vi "Tracker.vi"(8 "error in (no error)":errorcluster, 11 "Settings file path":path=path "D:/Users/Dmitriy/CData/CloudStation/Tracker_repository/SubVi's/Tracker_settings.tcf") -> (0 "error out":errorcluster)   [LabVIEW 2016]
uses:
  <vilib>/Utility/config.llb/Config Data RefNum.ctl
  <vilib>/Utility/miscctls.llb/LVPoint32TypeDef.ctl
  <vilib>/Utility/miscctls.llb/LVPointTypeDef.ctl
  <vilib>/Instr/_visa.llb/VISA Flush IO Buffer Mask.ctl
  <vilib>/Utility/miscctls.llb/LVRangeTypeDef.ctl
  <vilib>/Utility/miscctls.llb/LVBoundsTypeDef.ctl
  <vilib>/Utility/miscctls.llb/LVStringsAndValuesArrayTypeDef_U16.ctl
  <extravilib>/ChannelInstances/Lossy Stream-a[.,.](str)/Write With Abort.vi
  <extravilib>/ChannelInstances/Lossy Stream-a[.,.](str)/Read With Abort.vi
  <extravilib>/ChannelInstances/Lossy Stream-a[.,.](str)/Endpoint.vi
  SubVi's/SW_Globals.vi
  <vilib>/Utility/file.llb/Write Delimited Spreadsheet (string).vi
  <vilib>/Utility/file.llb/Read Delimited Spreadsheet (string).vi
  <extravilib>/ChannelInstances/Lossy Stream-a[.,.](str)/Instantiate.vi
  <extravilib>/ChannelInstances/Lossy Stream-a[.,.](str)/)Channel.vi
  <resource>/ChannelSupport/_ChannelSupport/WaitIfNeeded.vi
  <vilib>/Utility/config.llb/NI_LVConfig.lvlib
  <vilib>/Analysis/NI_AALBase.lvlib
  <extravilib>/ChannelInstances/Lossy Stream-a[.,.](str).lvlib
panel:
  in  "Map index (analysis)":i32
  in  "Full trace color":u32(colorbox)=16757314
  out "Current TTL status":u8
  out "TTL inputs":u8[](array[numeric])
  out "TTL outputs":u8[](array[numeric])
  out "Start/Stop in config":u32
  out "Start/Stop out pulses config":u32
  out "Changed IO":bool
  out "Sync capability":u8
  in  "IO parameters string":string
  out "Reset STIM":bool
  out "Reset REG":bool
  out "Init plot":bool=TRUE
  in  "Back to Settings":bool
  out "Zones preference array (loaded)":dbl[][](array[numeric])
  out "Current segment":dbl[](array[numeric])
  out "Absolute timestamp (rec)":dbl[](array[numeric])
  in  "Colors for Stim. setup":T1(array[cluster])=[{"Not Selected"=1143775, "Not Selected"=1143775}, {"Not Selected"=14517504, "Not Selected"=14517504}, {"Not Selected"=1976113, "Not Selected"=1976113}, {"Not Selected"=2575993, "Not Selected"=2575993}]
  out "Record":bool
  out "Stopped":bool
  out "Reset starting pulse":bool
  out "TTL is long enough":bool
  out "Started":bool
  out "Coords":T2={"Horizontal"=316, "Vertical"=127}
  out "Button":u16=1
  out "Settings file path":path
  out "Track path":path
  out "Index of the last recorded timepoint":i32
  out "ceil(x): smallest int >= x":dbl
  out "Application Directory":path
  out "Path to the settings file":path=path "D:/Users/Dmitriy/CData/CloudStation/Tracker_repository/Tracker_settings.tcf"
  out "Estim. res":dbl=0.2677563343586869
  in  "SD calc buffer length":u32=100
  out "Eff. save interval":sgl=7.981
  out "Relative timestamp (rec)":dbl[](array[numeric])
  out "FPS":dbl=27.77777777777778
  out "alpha rot. angle":dbl[](array[numeric])
  out "Y coord":dbl[](array[numeric])
  out "X coord":dbl[](array[numeric])
  out "Data column names":string[](array[string])
  out "Zones allocation array":i32[](array[numeric])
  out "Zones presence array":bool[](array[boolean])
  in  "Stop Button":bool
  out "Path to the latest saved temp file":path
  out "Temp file ready":bool
  out "Pixels per mm":dbl=1.1663076923076923
  out "Settings file refnum out":T3
  out "Current User":string="Researcher"
  in  "Main tab control":enum32{"Settings", "Recording", "Analysis"}(tab)
  out "IO status indicator":T4
  in  "Set IO config":bool
  in  "Jump to Analysis":bool
  in  "Reset stimuli":bool
  in  "Stimulus presets":T5(array[cluster]) {"TTL out" items=["1"=1, "2"=2, "1 + 2"=3]; "Stimulus, s" min=0 max=10000 step=0.1; "Time, s" min=0 max=10000 step=0.1; "Event type" items=["Time spent in zone", "Future options"]}
  in  "Stim. setup":T6(radio)=enum."Zone 13"
  out "Ready":bool=TRUE
  in  "Re-check HW connection":bool
  out "Board size":string="Large"
  in  "Reset regions":bool
  in  "Cage diameter, mm":u16(ring)=333 items=["180 mm"=180, "325 mm"=325, "333 mm"=333]
  in  "Start Tracking button":bool
  in  "Starting angle BORDER":i16
  in  "N segments BORDER":u8=5 max=8
  in  "N segments MIDFIELD":u8=3 min=1 max=4
  in  "Starting angle MIDFIELD":i16=30
  in  "Radius, mm MIDFIELD":u16=110
  in  "Radius, mm CENTER":u16=50 min=5 step=1
  out "Segments diagram":picture
  out "HW info":string
  out "Port":string="Large"
  in  "Bridge swap":bool
  in  "Reset barplot":bool
  out "Mouse speed digi":dbl=0.28949046360238656 caption="Mouse speed" format="%05.1f"
  out "Zone preference (normalized)":dbl[](graph)=[0.0, 0.0, 0.0, 0.0, 0.0, 0.0, 1.0, 0.0, 0.0, 0.0, 0.0]
  in  "Multiplyer of chart RX":u8(slide)=1 min=1 max=10 step=1 scale=1.0..6.0
  in  "Zones presence indicator":T7={"01"=TRUE, "02"=TRUE, "03"=TRUE, "04"=TRUE, "05"=TRUE, "06"=TRUE, "07"=TRUE, "08"=TRUE, "09"=TRUE, "10"=TRUE, "11"=TRUE, "12"=TRUE, "13"=TRUE}
  in  "Zones":bool=TRUE
  in  "Record/Stop":bool
  out "Diagram at recording":picture caption="Mouse track"
  in  "Trace, s":u16(slide)=5 max=30 step=1 scale=0.0..30.0
  in  "Data filtering":u16(ring)=5 items=["None"=0, "Kalman 1/3"=2, "Kalman 1/8"=3, "SG 3/5"=4, "SG 3/11"=5]
  out "Record timestamp":dbl format="%<%H:%M:%S%3u>t"
  out "Current Time":timestamp=timestamp(3610093053.229 s since 1904-01-01) format="%<%H:%M:%S %d.%m.%Y>T"
  in  "Exit 2":bool
  out "Mouse speed":waveform(dbl)(graph)={"t0"=timestamp(3610093053.229 s since 1904-01-01), "dt"=1.0, "Y"=[0.28949046360238656]}
  in  "Vertical offset":sgl caption="Bridge offset" min=-60 max=60 step=0.1 format="%#.1g"
  out "TTL IO 1 (recording)":bool caption="IO 1"
  out "TTL IO 2 (recording)":bool caption="IO 2"
  out "TTL IO 3 (recording)":bool caption="IO 3"
  out "TTL IO 4 (recording)":bool caption="IO 4"
  out "TTL REC":bool
  out "Data loading progress":dbl(slide) scale=0.0..100.0
  in  "Speed":u16(ring)=3 items=["25"=75, "10"=30, "6"=18, "4"=12, "2"=6, "1"=3, "2/3"=2, "1/3"=1]
  in  "Timeline":dbl(slide) min=0.0 step=1.0 scale=0.0..5.043 scale format="%<%H:%M:%S>t"
  in  "Multiplyer of chart RX 2":u8(slide)=1 min=1 max=10 step=1 scale=1.0..6.0
  out "Diagram at analysis":picture caption="Mouse track"
  in  "Play/Pause":bool
  out "Recorded at time":timestamp format="%<%H:%M:%S %d.%m.%Y>T"
  out "Recorded timestamp":dbl format="%<%H:%M:%S%3u>t"
  in  "Zones (analysis)":bool=TRUE caption="Zones"
  out "Mouse speed 2":waveform(dbl)(graph) caption="Mouse speed"
  out "Mouse speed digi 2":dbl format="%05.1f"
  out "Zones allocation (normalized) in analysis":dbl[](graph) caption="Zone preference (normalized)"
  out "Recorded by":string
  in  "Trace in analysis, s":u16(slide)=5 caption="Trace, s" max=30 step=1 scale=0.0..30.0
  in  "Open File":bool
  out "Mouse snout orientation swap (analysis)":bool caption="Swapped"
  in  "Show heatmap (analysis)":bool caption="Heat map"
  in  "Show full track (analysis)":bool caption="Full track"
  out "Vertical offset (analysis)":sgl caption="V. offset" min=-60 max=60 step=0.1 format="%#.1g"
  out "TTL IO 2 (analysis)":bool
  out "TTL IO 1 (analysis)":bool
  out "TTL IO 3 (analysis)":bool
  out "TTL IO 4 (analysis)":bool
  # "v.2.1.0"
  # "Cage segmentation"
  # "BORDER"
  # "CENTER"
  # "MIDFIELD"
  # "v.2.1.0"
  # "v.2.1.0"
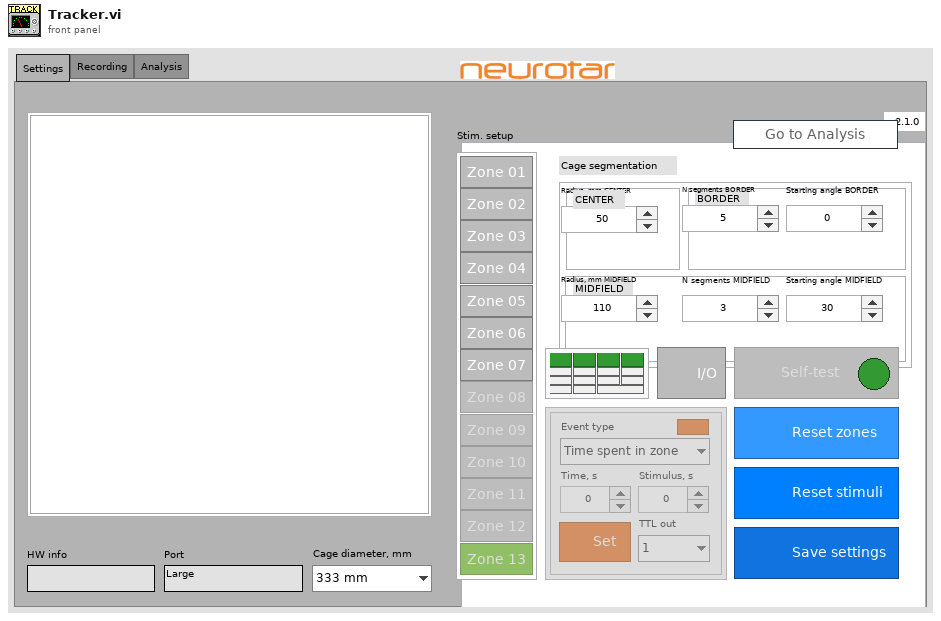
[diagram p1: front panel]
types:
  T1 = cluster{"Not Selected":u32, "Not Selected":u32}[]
  T2 = typedef "LVPoint32TypeDef.ctl" = cluster{"Horizontal":i32, "Vertical":i32}
  T3 = typedef "NI_LVConfig.lvlib/Config Data RefNum.ctl" = refnum<k1>
  T4 = cluster{"IO1":bool, "IO2":bool, "IO3":bool, "IO4":bool, "Z1":bool, "Z2":bool, "Z3":bool, "Z4":bool, "St1":bool, "St2":bool, "St3":bool, "St4":bool, "Syn1":bool, "Syn2":bool, "RS-232 ext. activated":bool}
  T5 = cluster{"Event type":u16, "Time, s":sgl, "Stimulus, s":sgl, "Set/Clear":bool, "TTL out":u16, "Stim. has been set":bool}[]
  T6 = enum32{"No Selection", "Zone 01", "Zone 02", "Zone 03", "Zone 04", "Zone 05", "Zone 06", "Zone 07", "Zone 08", "Zone 09", "Zone 10", "Zone 11", "Zone 12", "Zone 13"}
  T7 = cluster{"01":bool, "02":bool, "03":bool, "04":bool, "05":bool, "06":bool, "07":bool, "08":bool, "09":bool, "10":bool, "11":bool, "12":bool, "13":bool}
  T8 = cluster{"Numeric Control":u32, "Numeric Control":u32}[]
  T9 = enum8{"Enabled", "Disabled", "Disabled and Grayed Out"}
  T10 = cluster{"Read buffer":string, "Timestamp":timestamp}
  T11 = cluster{"Data acquisition status":refnum<notifier>, "Play/Pause status":refnum<notifier>, "Complete stop":refnum<notifier>, "Temp file ready for processing":refnum<notifier>, "Has been recorded":refnum<notifier>, "Recording now":refnum<notifier>, "Path to the latest complete temp file":refnum<notifier>, "Final CSV saved":refnum<notifier>, "Data loaded":refnum<notifier>}
  T12 = cluster{"SYNC configuration":u16, "IO 1 configuration":u16, "IO 2 configuration":u16, "IO 3 configuration":u16, "IO 4 configuration":u16, "Activate ext. RS-232":u16}
  T13 = typedef "VISA Flush IO Buffer Mask.ctl" = u16
  T14 = typedef "LVBoundsTypeDef.ctl" = cluster{"Width":u32, "Height":u32}
  T15 = cluster{"Amount of border segments":u8, "Border segments starting angle":i16, "Amount of midfield segments":u8, "Midfield segments starting angle":i16, "Midfield segments outer radius, mm":u16, "Amount of central segments":u8, "Center segment outer radius, mm":u16, "Diameter of the cage, mm":u16, "R-gap between segments, mm":u8}
  T16 = typedef "LVRangeTypeDef.ctl" = cluster{"Minimum":dbl, "Maximum":dbl, "Increment":dbl, "Minor Increment":dbl, "Start":dbl}
  T17 = cluster{"Width":u16, "Style":enum32{"Solid", "Dash", "Dot", "DashDot", "DashDotDot"}}
  T18 = cluster{"Temporary file output path":path, "Temporary csv output path":path, "Recording settings output path":path, "Final csv output path":path, "Background picture output path":path, "Path to the settings file":path}
  T19 = cluster{"Event type":u16, "Dur., s":sgl, "Stim., s":sgl, "Set/Clear":bool, "TTL out N":u16, "Stim. has been set":bool}[]
  T20 = cluster{"Researcher name":string, "Amount of midfield segments":u32, "Amount of border segments":u32, "Center segment outer radius, mm":u32, "Midfield segments outer radius, mm":u32, "Midfield segments starting angle":i32, "Border segments starting angle":i32, "Cage diameter, mm":u32, "Mouse snout orientation swap?":bool, "Vertical offset":dbl, "Settings loaded OK":bool}
  T21 = typedef "imagedata.ctl" = cluster{"image type":i32, "image depth":i32, "image":u8[], "mask":u8[], "colors":u32[], "Rectangle":cluster{"left":i16, "top":i16, "right":i16, "bottom":i16}}
  T22 = cluster{"Fonts scale factor":dbl, "Pixels per mm":dbl, "Radius of displayed outer segments, pix":dbl, "Radius of displayed midfield segments, pix":dbl, "Radius of displayed central segment, pix":dbl}
  T23 = typedef "Lossy Stream-a[.,.](str).lvlib/)Channel.ctl" = refnum<queue>
  T24 = cluster{"Read buffer":string, "Timestamp":timestamp}[]
  T25 = enum32{"No Selection", "Zone 01", "Zone 02", "Zone 03", "Zone 04", "Zone 05", "Zone 06", "Zone 07", "Zone 08", "Zone 09", "Zone 10", "Zone 11", "Zone 12", "Zone 13", "Zone 14"}
  T26 = enum32{"Page Enabled", "Page Disabled", "Page Disabled & Grayed"}
  T27 = typedef "LVPointTypeDef.ctl" = cluster{"Horizontal":i16, "Vertical":i16}
  T28 = enum32{"invalid app kind", "Development System", "Run Time System", "Student Edition", "Embedded LabVIEW", "Evaluation", "Custom"}
  T29 = cluster{"N segments BORDER":u8, "Starting angle BORDER":i16, "N segments MIDFIELD":u8, "Starting angle MIDFIELD":i16, "Radius, mm MIDFIELD":u16, "Amount of central segments":u8, "Radius, mm CENTER":u16}
  T30 = cluster{"Event type":u16, "Cond., s":sgl, "Stim., s":sgl, "Set/Clear":bool, "TTL out N":u16, "Stim. has been set":bool}
  T31 = cluster{"SYNC configuration":bool, "IO 1 configuration":bool, "IO 2 configuration":bool, "IO 3 configuration":bool, "IO 4 configuration":bool, "Activate ext. RS-232":bool}
  T32 = cluster{"Event type":u16, "Time, s":sgl, "Stimulus, s":sgl, "Set/Clear":bool, "TTL out":u16, "Stim. has been set":bool}
  T33 = typedef "LVStringsAndValuesArrayTypeDef_U16.ctl" = cluster{"String":string, "Value":u16}[]
  T34 = cluster{"N segments BORDER":u8, "Starting angle BORDER":i16, "N segments MIDFIELD":u8, "Starting angle MIDFIELD":i16, "Radius, mm MIDFIELD":u16, u8, "Radius, mm CENTER":u16, "Cage diameter, mm":u16, i32}
  T35 = cluster{"N segments BORDER":u8, "Starting angle BORDER":i16, "N segments MIDFIELD":u8, "Starting angle MIDFIELD":i16, "Radius, mm MIDFIELD":u16, "N segments CENTER":u8, "Radius, mm CENTER":u16, "Cage diameter, mm":u16, "R-gap":i32}
  T36 = cluster{"Zone[1]":bool, "Zone[2]":bool, "Zone[3]":bool, "Zone[4]":bool, "Zone[5]":bool, "Zone[6]":bool, "Zone[7]":bool, "Zone[8]":bool, "Zone[9]":bool, "Zone[10]":bool, "Zone[11]":bool, "Zone[12]":bool, "Zone[13]":bool}
  T37 = cluster{"Temporary file output path":path, "Temporary csv output path":path, "Recording settings output path":path, "Final output path":path, "Background picture output path":path, "Path to the settings file":path}
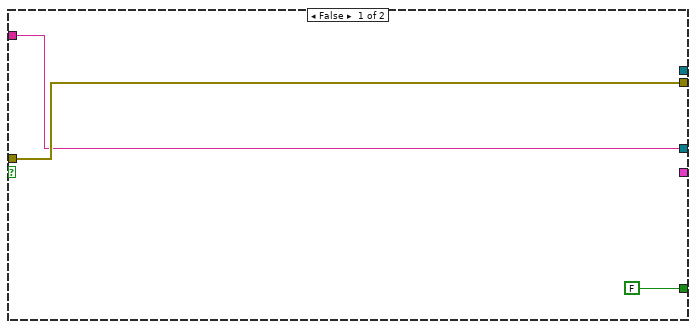
[diagram p2: hidden frame]
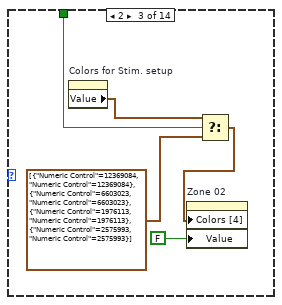
[diagram p4: hidden frame]
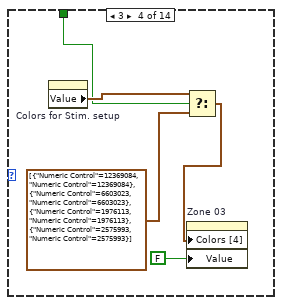
[diagram p5: hidden frame]
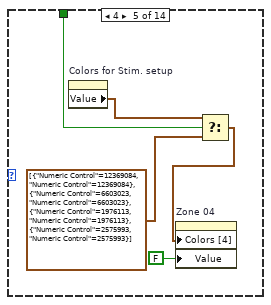
[diagram p6: hidden frame]
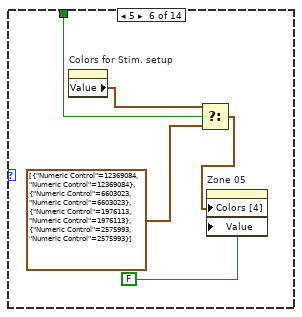
[diagram p7: hidden frame]
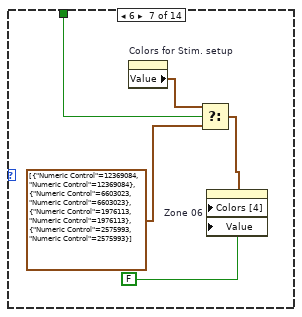
[diagram p8: hidden frame]
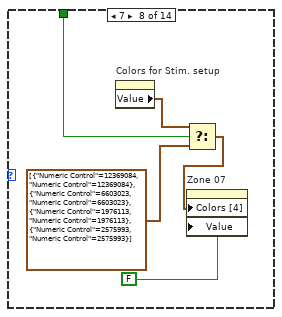
[diagram p9: hidden frame]
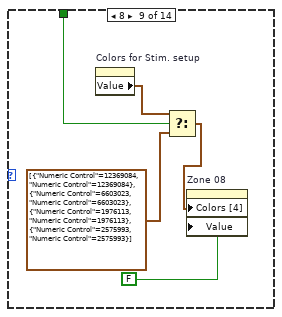
[diagram p10: hidden frame]
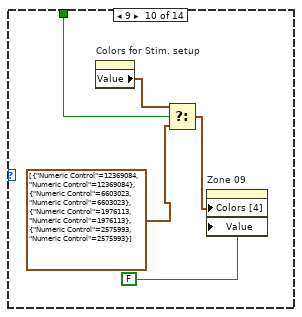
[diagram p11: hidden frame]
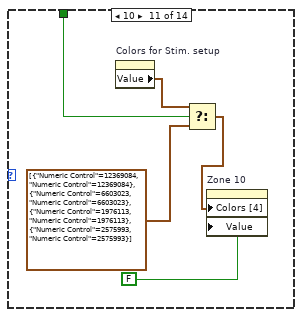
[diagram p12: hidden frame]
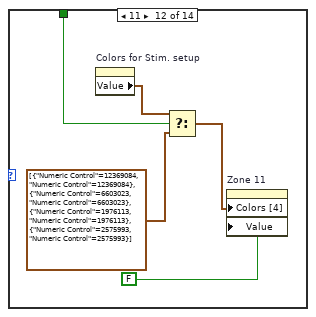
[diagram p13: hidden frame]
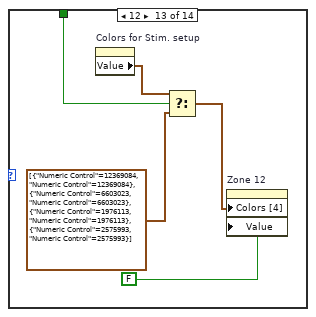
[diagram p14: hidden frame]
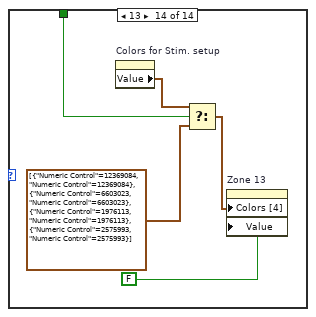
[diagram p15: hidden frame]
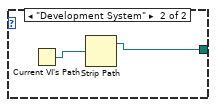
[diagram p16: hidden frame]
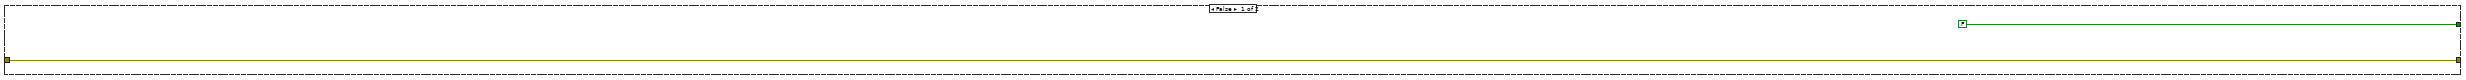
[diagram p20: hidden frame]
diagram:
  n1 = property on="Re-check HW connection" class="Bool"("DisabledEnum"=T9."Disabled and Grayed Out" ("Disabled")) -> (error out=w10:errorcluster)  [unwired: 2 in, 1 out]
  n2 = property on="Ready" class="Bool (strict)"(error in=w10, "Value"=FALSE ("Ready"), "Colors [4]"=T8 [{"Numeric Control"=16749459, "Numeric Control"=16749459}, {"Numeric Control"=1988894, "Numeric Control"=3381555}, {"Numeric Control"=4934475, "Numeric Control"=7895160}, {"Numeric Control"=994319, "Numeric Control"=1657881}]) -> (error out=w6:errorcluster)  [unwired: 1 in, 1 out]
  n3 = while {
    tunnel: w19 -> [w39]
    tunnel: [w36] -> w18
    tunnel: [w38] -> w3
    tunnel: [w21] -> w12
    tunnel: [w37] -> w5
    tunnel: w6 -> [w31]
    tunnel: [w24] -> w2
    stop <- w36 stop-if-true
    n4 = Wait Until Next ms Multiple(millisecond multiple=u32 1201) -> ()  [unwired: 1 out]
    n5 = property on="Re-check HW connection" class="Bool"(error in=w31, "DisabledEnum"=T9."Enabled" ("Disabled")) -> (error out=w30:errorcluster)  [unwired: 1 in, 1 out]
    n6 = First Call?() -> (First Call?: T/F=w22:bool)
    n7 = property on="Ready" class="Bool (strict)"(error in=w30) -> (error out=w35:errorcluster, "Value"=w34:bool)  [unwired: 1 in, 1 out]
    n8 = Or(x=w22, y="Re-check HW connection") -> (x .or. y?=w23:bool)
    n9 = Not(x=w34) -> (.not. x?=w29:bool)
    n10 = And(x=w29, y=w23) -> (x .and. y?=w28:bool)
    n11 = case shown="True" w28 {
      tunnel: w39 -> [w41 w68]
      tunnel: [_ w67] -> w38
      tunnel: [w41 w66] -> w21
      tunnel: [_ w65] -> w37
      tunnel: [w42 w51] -> w25
      tunnel: [FALSE ("Instrument OK?") w55] -> w36
      tunnel: w35 -> [w42 w53]
      frame False {
      }
      frame True {
        w64 = T10 {"Read buffer"="", "Timestamp"=timestamp(3605695211.9516535 s since 1904-01-01)}  # Data frame example
        n12 = property on="Ready" class="Bool (strict)"(error in=w53, "Colors [4]"=T8 [{"Numeric Control"=16749459, "Numeric Control"=16176658}, {"Numeric Control"=1988894, "Numeric Control"=3381555}, {"Numeric Control"=4934475, "Numeric Control"=7895160}, {"Numeric Control"=994319, "Numeric Control"=1657881}]) -> (error out=w52:errorcluster)  [unwired: 1 in, 1 out]
        n13 = Obtain Queue(name (unnamed)="Data flow", element data type=w64, error in (no error)=w52) -> (queue out=w67:refnum<queue>, error out=w62:errorcluster)  [unwired: 2 in, 1 out]
        n14 = call "HW_Setup.vi"("VISA resource name in"=w68, "Traget FPS"=80, "error in"=w62) -> ("error out"=w51:errorcluster, "Sensor board size"=w43:string, "VISA resource name out"=w66:refnum<visa-resource-name>, "Data flow controls"=w65:T11, "Version information"=w50:string, "Instrument OK?"=w55:bool)  [unwired: 1 in, 1 out]
        "Ready" <- w55
        "Board size" <- w43
        n15 = String Length(string=w50) -> (length=w59:i32)
        n16 = Equal?(x=w50, y="1.1.4") -> (x = y?=w47:bool)
        n17 = Greater Than 0?(x=w59) -> (x > 0?=w58:bool)
        n18 = Concatenate Strings(w43, ", FW: " ("string"), w50) -> (w57:string)
        n19 = Select(t=u8 0, s=w47, f=u8 1) -> (s? t:f=→"Sync capability":u8)
        n20 = Select(t=w57, s=w58, f="Not connected") -> (s? t:f=→"HW info":string)
      }
    }
    n21 = global write "SW_Globals.vi" "VISA resource name out"(w21) -> ()
    n22 = property on="Ready" class="Bool (strict)"(error in=w25, "Colors [4]"=T8 [{"Numeric Control"=16749459, "Numeric Control"=16749459}, {"Numeric Control"=1988894, "Numeric Control"=3381555}, {"Numeric Control"=4934475, "Numeric Control"=7895160}, {"Numeric Control"=994319, "Numeric Control"=1657881}]) -> (error out=w24:errorcluster)  [unwired: 1 in, 1 out]
  }
  n23 = property on="Re-check HW connection" class="Bool"(error in=w2, "DisabledEnum"=T9."Disabled and Grayed Out" ("Disabled")) -> (error out=w7:errorcluster)  [unwired: 1 in, 1 out]
  n24 = while "In this loop raw data from the device is obtained and TTLs are fired" {
    tunnel: w12 -> [w86]
    tunnel: w7 -> [w84]
    tunnel: [w93] -> w17
    tunnel: [w94] -> w16
    tunnel: [w107] -> w20
    tunnel: w5 -> [w105]
    tunnel: w3 -> [w87]
    stop <- w97 stop-if-true
    w74 = u16 4 ("y")
    n25 = Unbundle By Name(w105) -> ("Complete stop"=w104:refnum<notifier>, "Recording now"=w101:refnum<notifier>, "Has been recorded"=w100:refnum<notifier>)
    n26 = global read "SW_Globals.vi" "IO parameters cluster"() -> (w77:T12)
    n27 = property on="Start/Stop out pulses config" class="DigNum (strict)"() -> ("Value"=w78:u32)  [unwired: 2 in, 2 out]
    n28 = Greater Than 0?(x=w78) -> (x > 0?=w79:bool)
    n29 = Get Notifier Status(notifier=w100) -> (current notification=w99:bool)  [unwired: 1 in, 4 out]
    n30 = Get Notifier Status(notifier=w104) -> (current notification=w97:bool)  [unwired: 1 in, 4 out]
    n31 = Get Notifier Status(notifier=w101) -> (current notification=w88:bool)  [unwired: 1 in, 4 out]
    n32 = Unbundle By Name(w77) -> ("IO 1 configuration"=w76:u16, "IO 2 configuration"=w75:u16)
    n33 = local read "Sync capability"() -> (w73:u8)
    n34 = Not(x=w88) -> (.not. x?=w81:bool)
    n35 = And(x=w81, y=w99) -> (x .and. y?=w98:bool)
    n36 = Or(x=w98, y=w97) -> (x .or. y?=w92:bool)
    n37 = Greater Than 0?(x=w73) -> (x > 0?=w72:bool)
    n38 = Equal?(x=w76, y=w74) -> (x = y?=w71:bool)
    n39 = Equal?(x=w75, y=w74) -> (x = y?=w70:bool)
    n40 = Or(x=w71, y=w70) -> (x .or. y?=w69:bool)
    n41 = Compound Arithmetic op=AND(w81, w69, w72) -> (w82:bool)
    n42 = case shown="True" w82 {
      tunnel: w86 -> [w109 w114]
      tunnel: w84 -> [w108 w115]
      tunnel: [w109 w113] -> w85
      tunnel: [w108 w112] -> w83
      tunnel: w71 -> [_ w111]
      tunnel: w70 -> [_ w110]
      frame False {
      }
      frame True {
        n43 = First Call?() -> (First Call?: T/F=w116:bool)
        n44 = case shown="True" w116 {
          tunnel: w115 -> [w117 w134]
          tunnel: w114 -> [w118 w133]
          tunnel: [w118 w129] -> w113
          tunnel: [w117 w131] -> w112
          tunnel: w111 -> [_ w123]
          tunnel: w110 -> [_ w122]
          frame False {
          }
          frame True {
            w128 = T13 16 items=["Flush Receive Buffer"=16, "Write Transmit Buffer to Device"=32, "Flush Receive Buffer (No I/O)"=64, "Flush Transmit Buffer"=128] ("Mask")
            n45 = And(x=w123, y=w122) -> (x .and. y?=w127:bool)
            n46 = Greater?(x=w123, y=w122) -> (0:w121:bool)
            n47 = Select(t="SYNC=1" ("string"), s=w121, f="SYNC=2" ("string")) -> (s? t:f=w119:string)
            n48 = Select(t="SYNC=3" ("string"), s=w127, f=w119) -> (s? t:f=w125:string)
            n49 = Concatenate Strings(w125, "\r") -> (w136:string)
            n50 = VISA Write(VISA resource name=w133, write buffer=w136, error in (no error)=w134) -> (VISA resource name out=w130:refnum<visa-resource-name>, error out=w132:errorcluster)  [unwired: 1 out]
            n51 = VISA Flush I/O Buffer(VISA resource name=w130, mask (16)=w128, error in (no error)=w132) -> (VISA resource name out=w129:refnum<visa-resource-name>, error out=w131:errorcluster)
          }
        }
      }
    }
    n52 = case "Inside this case structure TTL can be fired at the start of the recording" shown="True" w88 {
      tunnel: w79 -> [_ w168]
      tunnel: w83 -> [w158 w167]
      tunnel: [w158 w166] -> w89
      tunnel: w85 -> [w159 w165]
      tunnel: [w159 w164] -> w91
      tunnel: [w157 w163] -> w90
      tunnel: w87 -> [w157 w162]
      tunnel: w78 -> [_ w161]
      frame False {
        n53 = First Call?() -> (First Call?: T/F=w156:bool)
        n54 = case shown="True" w156 {
          frame False {
          }
          frame True {
            n55 = Get Date/Time In Seconds() -> (seconds since 1Jan1904=w160:timestamp)
            n56 = global write "SW_Globals.vi" "Recording start timestamp"(w160) -> ()
          }
        }
      }
      frame True {
        n57 = First Call?() -> (First Call?: T/F=w169:bool)
        n58 = case shown="True" w169 {
          tunnel: w168 -> [_ w188]
          tunnel: w167 -> [w172 w187]
          tunnel: [w172 w182] -> w166
          tunnel: w165 -> [w171 w186]
          tunnel: [w171 w185] -> w164
          tunnel: [w170 w183] -> w163
          tunnel: w162 -> [w170 w184]
          tunnel: w161 -> [_ w174]
          tunnel: w161 -> [_ w173]
          frame False {
          }
          frame True {
            n59 = flat-sequence {
              tunnel: w184 -> [w201]
              tunnel: w186 -> [w202]
              tunnel: w187 -> [w199]
              tunnel: w188 -> [w200]
              tunnel: [w200] -> w181
              tunnel: [w199] -> w180
              tunnel: [w202] -> w179
              tunnel: [w201] -> w178
              tunnel: w173 -> [w189]
              tunnel: [w207] -> w177
              tunnel: [w212] -> w176
              tunnel: [w211] -> w175
              tunnel: w181 -> [w204]
              tunnel: w180 -> [w210]
              tunnel: w179 -> [w209]
              tunnel: w178 -> [w213]
              tunnel: w174 -> [w203]
              tunnel: [w224] -> w182
              tunnel: [w226] -> w183
              tunnel: [w227] -> w185
              tunnel: w175 -> [w224]
              tunnel: w176 -> [w226]
              tunnel: w177 -> [w227]
              frame #0 {
                n60 = Number To Boolean Array(number=w189) -> (Boolean array=w193:bool[])
                n61 = Index Array(array=w193, index=3) -> (element=w195:bool)
                n62 = Index Array(array=w193, index=2) -> (element=w196:bool)
                n63 = Index Array(array=w193, index=1) -> (element=w197:bool)
                n64 = Index Array(array=w193, index=0) -> (element=w198:bool)
                n65 = property on="TTL IO 4 (recording)" class="Bool (strict)"("Value"=w195) -> ()  [unwired: 2 in, 2 out]
                n66 = property on="TTL IO 3 (recording)" class="Bool (strict)"("Value"=w196) -> ()  [unwired: 2 in, 2 out]
                n67 = property on="TTL IO 2 (recording)" class="Bool (strict)"("Value"=w197) -> ()  [unwired: 2 in, 2 out]
                n68 = property on="TTL IO 1 (recording)" class="Bool (strict)"("Value"=w198) -> ()  [unwired: 2 in, 2 out]
              }
              frame #1 {
                n69 = call "SW_Fire_TTL_at_start_universal.vi"("TTL port(s) config to fire"=w203, "TTL pulse length, ms"=100.0, "error in (no error)"=w210, "Serial Port In"=w209, "Close VISA (T)"=FALSE, "Start/stop signaling (F)"=w204) -> ("error out"=w208:errorcluster, "Serial Port Out"=w207:refnum<visa-resource-name>)  [unwired: 3 in, 1 out]
                n70 = Flush Queue(queue=w213, error in (no error)=w208) -> (queue out=w212:refnum<queue>, error out=w211:errorcluster)  [unwired: 1 out]
              }
              frame #2 {
                n71 = Get Date/Time In Seconds() -> (seconds since 1Jan1904=w225:timestamp)
                n72 = Number To Boolean Array(number=u32 0) -> (Boolean array=w220:bool[])
                n73 = global write "SW_Globals.vi" "Recording start timestamp"(w225) -> ()
                n74 = Index Array(array=w220, index=3) -> (element=w218:bool)
                n75 = Index Array(array=w220, index=2) -> (element=w217:bool)
                n76 = Index Array(array=w220, index=1) -> (element=w216:bool)
                n77 = Index Array(array=w220, index=0) -> (element=w215:bool)
                n78 = property on="TTL IO 4 (recording)" class="Bool (strict)"("Value"=w218) -> ()  [unwired: 2 in, 2 out]
                n79 = property on="TTL IO 3 (recording)" class="Bool (strict)"("Value"=w217) -> ()  [unwired: 2 in, 2 out]
                n80 = property on="TTL IO 2 (recording)" class="Bool (strict)"("Value"=w216) -> ()  [unwired: 2 in, 2 out]
                n81 = property on="TTL IO 1 (recording)" class="Bool (strict)"("Value"=w215) -> ()  [unwired: 2 in, 2 out]
              }
            }
          }
        }
      }
    }
    n82 = call "HW_Stream_raw_data_enq.vi"("error in"=w89, "Queue in"=w90, "Data flow controls in"=w105, "VISA resource name in"=w91) -> ("error out"=w102:errorcluster, "Data flow controls out"=w107:T11, "VISA resource name out"=w103:refnum<visa-resource-name>)  [unwired: 4 in, 1 out]
    n83 = case "Inside this case structure TTL can be fired at the end of the recording" shown="True" w92 {
      selector: w92 -> [w228 w233]
      tunnel: w103 -> [w229 w237]
      tunnel: [w230 w239] -> w96
      tunnel: w102 -> [w230 w238]
      tunnel: [w229 w236] -> w95
      tunnel: w79 -> [_ w235]
      tunnel: [w228 w233] -> w80
      tunnel: w78 -> [_ w232]
      tunnel: w78 -> [_ w231]
      frame False {
      }
      frame True {
        n84 = First Call?() -> (First Call?: T/F=w234:bool)
        n85 = case shown="True" w234 {
          tunnel: [w241 w253] -> w239
          tunnel: w238 -> [w241 w252]
          tunnel: w237 -> [w240 w251]
          tunnel: [w240 w250] -> w236
          tunnel: w235 -> [_ w249]
          tunnel: w232 -> [_ w242]
          tunnel: w231 -> [_ w243]
          frame False {
          }
          frame True {
            n86 = flat-sequence {
              tunnel: w249 -> [w265]
              tunnel: w251 -> [w266]
              tunnel: w252 -> [w264]
              tunnel: [w264] -> w246
              tunnel: [w266] -> w245
              tunnel: [w265] -> w244
              tunnel: w243 -> [w254]
              tunnel: [w274] -> w248
              tunnel: [w273] -> w247
              tunnel: w246 -> [w271]
              tunnel: w245 -> [w268]
              tunnel: w244 -> [w269]
              tunnel: w242 -> [w267]
              tunnel: [w286] -> w250
              tunnel: [w285] -> w253
              tunnel: w248 -> [w285]
              tunnel: w247 -> [w286]
              frame #0 {
                n87 = Number To Boolean Array(number=w254) -> (Boolean array=w260:bool[])
                n88 = Index Array(array=w260, index=3) -> (element=w258:bool)
                n89 = Index Array(array=w260, index=2) -> (element=w257:bool)
                n90 = Index Array(array=w260, index=1) -> (element=w256:bool)
                n91 = Index Array(array=w260, index=0) -> (element=w255:bool)
                n92 = property on="TTL IO 4 (recording)" class="Bool (strict)"("Value"=w258) -> ()  [unwired: 2 in, 2 out]
                n93 = property on="TTL IO 3 (recording)" class="Bool (strict)"("Value"=w257) -> ()  [unwired: 2 in, 2 out]
                n94 = property on="TTL IO 2 (recording)" class="Bool (strict)"("Value"=w256) -> ()  [unwired: 2 in, 2 out]
                n95 = property on="TTL IO 1 (recording)" class="Bool (strict)"("Value"=w255) -> ()  [unwired: 2 in, 2 out]
              }
              frame #1 {
                n96 = call "SW_Fire_TTL_at_stop_universal.vi"("TTL port(s) config to fire"=w267, "TTL pulse length, ms"=200.0, "error in (no error)"=w271, "Serial Port In"=w268, "Close VISA (T)"=FALSE, "Start/stop signaling (F)"=w269) -> ("error out"=w274:errorcluster, "Serial Port Out"=w273:refnum<visa-resource-name>)  [unwired: 3 in, 1 out]
              }
              frame #2 {
                n97 = Number To Boolean Array(number=u32 0) -> (Boolean array=w278:bool[])
                n98 = Index Array(array=w278, index=3) -> (element=w280:bool)
                n99 = Index Array(array=w278, index=2) -> (element=w281:bool)
                n100 = Index Array(array=w278, index=1) -> (element=w282:bool)
                n101 = Index Array(array=w278, index=0) -> (element=w283:bool)
                n102 = property on="TTL IO 4 (recording)" class="Bool (strict)"("Value"=w280) -> ()  [unwired: 2 in, 2 out]
                n103 = property on="TTL IO 3 (recording)" class="Bool (strict)"("Value"=w281) -> ()  [unwired: 2 in, 2 out]
                n104 = property on="TTL IO 2 (recording)" class="Bool (strict)"("Value"=w282) -> ()  [unwired: 2 in, 2 out]
                n105 = property on="TTL IO 1 (recording)" class="Bool (strict)"("Value"=w283) -> ()  [unwired: 2 in, 2 out]
              }
            }
          }
        }
      }
    }
    n106 = Wait Until Next ms Multiple(millisecond multiple=u32 1) -> ()  [unwired: 1 out]
    n107 = case shown="True" w80 {
      tunnel: w95 -> [w138 w141]
      tunnel: w96 -> [w137 w142]
      tunnel: [w138 w140] -> w94
      tunnel: [w137 w139] -> w93
      frame False {
      }
      frame True {
        n108 = First Call?() -> (First Call?: T/F=w143:bool)
        n109 = case shown="True" w143 {
          tunnel: w142 -> [w144 w152]
          tunnel: w141 -> [w145 w151]
          tunnel: [w145 w147] -> w140
          tunnel: [w144 w149] -> w139
          frame False {
          }
          frame True {
            w146 = T13 16 items=["Flush Receive Buffer"=16, "Write Transmit Buffer to Device"=32, "Flush Receive Buffer (No I/O)"=64, "Flush Transmit Buffer"=128] ("Mask")
            n110 = Concatenate Strings("SYNC=0" ("string"), "\r") -> (w155:string)
            n111 = VISA Write(VISA resource name=w151, write buffer=w155, error in (no error)=w152) -> (VISA resource name out=w148:refnum<visa-resource-name>, error out=w150:errorcluster)  [unwired: 1 out]
            n112 = VISA Flush I/O Buffer(VISA resource name=w148, mask (16)=w146, error in (no error)=w150) -> (VISA resource name out=w147:refnum<visa-resource-name>, error out=w149:errorcluster)
          }
        }
      }
    }
  }
  n113 = case shown="False" w18 {
    frame False {
      n114 = property on="Start Tracking button" class="Bool"("DisabledEnum"=T9."Disabled and Grayed Out" ("Disabled")) -> ()  [unwired: 2 in, 2 out]
    }
    frame True {
      n115 = property on="Start Tracking button" class="Bool"("DisabledEnum"=T9."Enabled" ("Disabled")) -> ()  [unwired: 2 in, 2 out]
    }
  }
  n116 = call "HW_Stop_acq_and_close_VISA.vi"("error in"=w17, "Data flow controls in"=w20, "VISA resource name in"=w16) -> ()  [unwired: 2 out]
  n117 = while "This loop is used only for data loading purposes (that is why it is made relatively slow)" {
    tunnel: w5 -> [w294]
    stop <- w290 stop-if-true
    n118 = Unbundle By Name(w294) -> ("Has been recorded"=w292:refnum<notifier>, "Final CSV saved"=w300:refnum<notifier>, "Data loaded"=w299:refnum<notifier>, "Complete stop"=w291:refnum<notifier>)
    n119 = Wait Until Next ms Multiple(millisecond multiple=u32 139) -> ()  [unwired: 1 out]
    n120 = Get Notifier Status(notifier=w292) -> (current notification=w296:bool)  [unwired: 1 in, 4 out]
    n121 = Get Notifier Status(notifier=w300) -> (current notification=w298:bool)  [unwired: 1 in, 4 out]
    n122 = Get Notifier Status(notifier=w299) -> (current notification=w295:bool)  [unwired: 1 in, 4 out]
    n123 = Get Notifier Status(notifier=w291) -> (current notification=w290:bool)  [unwired: 1 in, 4 out]
    n124 = Not(x=w295) -> (.not. x?=w297:bool)
    n125 = Compound Arithmetic op=AND(w296, w298, w297) -> (w289:bool)
    n126 = case shown="True" w289 {
      tunnel: w294 -> [_ w391]
      frame False {
      }
      frame True {
        w303 = T17 {"Width"=2, "Style"=enum."Solid"} ("pen")
        n127 = property on="Zones (analysis)" class="Bool (strict)"("DisabledEnum"=T9."Enabled" ("Disabled")) -> (error out=w346:errorcluster)  [unwired: 2 in, 1 out]
        n128 = global read "SW_Globals.vi" "Array of the presence count"() -> (w322:u32[][])
        n129 = for {
          N: 256 -> [w417]
          tunnel: [w413] -> w353 mode=indexing
          i -> [w418]
          n130 = Decrement(x=w417) -> (x-1=w414:i32)
          n131 = Divide(x=w418, y=w414) -> (x/y=w416:dbl)
          n132 = Interpolate 1D Array(1:w416, 2:dbl[] [0.0, 4000000000.0] ("array of numbers or points")) -> (0:w415:dbl)
          n133 = To Unsigned Byte Integer(number=w415) -> (unsigned 8bit integer=w413:u8)
        }
        n134 = property on="Data loading progress" class="Slide (strict)"(error in=w346, "DisabledEnum"=T9."Disabled" ("Disabled"), "Value"=0.0 ("Data loading progress")) -> (error out=w389:errorcluster)  [unwired: 1 in, 1 out]
        n135 = control-ref of="Data loading progress"() -> (w393:refnum<vi>)
        n136 = Array Max & Min(array=w322) -> (max value=w358:u32)  [unwired: 3 out]
        n137 = global read "SW_Globals.vi" "Cluster of paths"() -> (w392:T18)
        n138 = Divide(x=w322, y=w358) -> (x/y=w357:dbl[][])
        n139 = property on="Play/Pause" class="Bool (strict)"(error in=w389, "DisabledEnum"=T9."Disabled and Grayed Out" ("Disabled")) -> (error out=w387:errorcluster)  [unwired: 1 in, 1 out]
        n140 = call "SW_Load_data_for_Analysis.vi"("Data flow controls"=w391, "Cluster of paths input"=w392, "Progress bar reference"=w393, "error in (no error)"=w387) -> ("Data column names"=→"Data column names":string[], "Stimulus presets array (loaded)"=w328:T19, "TTL inputs"=→"TTL inputs":u8[], "TTL outputs"=→"TTL outputs":u8[], "Absolute timestamp"=→"Absolute timestamp (rec)":dbl[], "Zones preference array (loaded)"=→"Zones preference array (loaded)":dbl[][], "Relative timestamp"=w381:dbl[], "Acquisition settings cluster out"=w374:T20, "X coord"=w313:dbl[], "Y coord"=w312:dbl[], "alpha rot. angle"=→"alpha rot. angle":dbl[], "Current zone"=→"Current segment":dbl[], "error out"=w326:errorcluster)  [unwired: 3 in]
        "Y coord" <- w312
        "X coord" <- w313
        "Relative timestamp (rec)" <- w381
        n141 = for {
          tunnel: w328 -> [w412] mode=indexing
          tunnel: [w410] -> w327 mode=indexing if=w409
          i -> [w411]
          n142 = Unbundle By Name(w412) -> ("Stim. has been set"=w409:bool)
          n143 = To Unsigned Byte Integer(number=w411) -> (unsigned 8bit integer=w410:u8)
        }
        n144 = global write "SW_Globals.vi" "Regions to track"(w327) -> ()
        n145 = Multiply(x=w357, y=255) -> (x*y=w355:dbl[][])
        n146 = call <vilib>:"Flatten Pixmap.vi"("colors"=w353, "8-bit pixmap"=w355) -> ("image data"=w323:T21)  [unwired: 9 in]
        n147 = property on="Data loading progress" class="Slide (strict)"(error in=w326, "DisabledEnum"=T9."Disabled and Grayed Out" ("Disabled")) -> (error out=w384:errorcluster)  [unwired: 1 in, 1 out]
        n148 = Unbundle By Name(w374) -> ("Vertical offset"=w344:dbl, "Mouse snout orientation swap?"=→"Mouse snout orientation swap (analysis)":bool, "Cage diameter, mm"=w338:u32, "Amount of border segments"=w337:u32, "Border segments starting angle"=w336:i32, "Amount of midfield segments"=w335:u32, "Midfield segments starting angle"=w334:i32, "Midfield segments outer radius, mm"=w332:u32, "Center segment outer radius, mm"=w331:u32, "Researcher name"=w371:string)
        "Vertical offset (analysis)" <- w344
        n149 = call <vilib>:"Draw Flattened Pixmap.vi"("image data"=w323) -> ("new picture"=w321:picture)  [unwired: 8 in]
        n150 = Array Max & Min(array=w381) -> (max value=w379:dbl, max index (indices)=→"Index of the last recorded timepoint":i32, min value=w378:dbl)  [unwired: 1 out]
        n151 = property on="Diagram at analysis" class="Pict"() -> ("Bounds"=w307:T14)  [unwired: 2 in, 2 out]
        n152 = property on="Vertical offset" class="DigNum (strict)"("Value"=w344) -> ()  [unwired: 2 in, 2 out]
        n153 = call <vilib>:"Picture to Pixmap.vi"("picture"=w321) -> ("image data"=w320:T21)  [unwired: 9 in, 1 out]
        n154 = call <vilib>:"Unflatten Pixmap.vi"("image data"=w320) -> ("24-bit pixmap"=w319:u32[][])  [unwired: 4 in, 6 out]
        n155 = Quotient & Remainder(x=w307, y=T14 {"Width"=2, "Height"=2}) -> (floor(x/y)=w306:T14)  [unwired: 1 out]
        n156 = Compound Arithmetic op=ADD(w337, w335, u32 1 ("value")) -> (w349:u32)
        n157 = global write "SW_Globals.vi" "Active segments amount"(w349) -> ()
        n158 = Increment(x=w349) -> (x+1=w348:u32)
        n159 = property on="Play/Pause" class="Bool (strict)"(error in=w384, "DisabledEnum"=T9."Enabled" ("Disabled")) -> (error out=w380:errorcluster)  [unwired: 1 in, 1 out]
        n160 = Concatenate Strings("Recorded by " ("string"), w371) -> (→"Recorded by":string)
        n161 = Round To Nearest(number=w378) -> (nearest integer value=w376:dbl)
        n162 = Bundle By Name(cluster=T16 {"Minimum"=0.0, "Maximum"=14.0, "Increment"=1.0, "Minor Increment"=1.0, "Start"=0.0} ("X Scale.Range"), "Maximum"=w348) -> (w347:T16)
        n163 = property on="Timeline" class="Slide (strict)"(error in=w380, "Scale.Maximum"=w379, "Scale.Minimum"=w376, "Value"=w376, "DisabledEnum"=T9."Disabled and Grayed Out" ("Disabled")) -> (error out=w372:errorcluster)  [unwired: 1 in, 1 out]
        n164 = property on="Zones allocation (normalized) in analysis" class="WFGraph (strict)"("XScale.Range"=w347) -> ()  [unwired: 2 in, 2 out]
        n165 = control-ref of="Zones allocation array"() -> (w362:refnum<vi>)
        n166 = property on="Diagram at analysis" class="Pict"(error in=w372) -> (error out=w330:errorcluster, "Bounds"=w340:T14)  [unwired: 1 in, 1 out]
        n167 = Bundle By Name(cluster=T15 {"Amount of border segments"=8, "Border segments starting angle"=0, "Amount of midfield segments"=4, "Midfield segments starting angle"=0, "Midfield segments outer radius, mm"=60, "Amount of central segments"=1, "Center segment outer radius, mm"=30, "Diameter of the cage, mm"=180, "R-gap between segments, mm"=10} ("Input cluster of parameters"), "Diameter of the cage, mm"=w338, "Amount of border segments"=w337, "Border segments starting angle"=w336, "Amount of midfield segments"=w335, "Midfield segments starting angle"=w334, "Midfield segments outer radius, mm"=w332, "Center segment outer radius, mm"=w331) -> (w333:T15)
        n168 = call "SW_Generate_Segmented_Plot_v3.vi"("Draw Area Size"=w340, "Regions to mark set"=w327, "Input cluster of parameters"=w333, "Error In"=w330) -> ("Zones layout output"=w311:picture, "No zones image"=w301:picture, "Array of the pixel to color correspondences"=w342:u32[][], "Array of the segment to color correspondences"=w343:u32[][], "Cluster of image geometrical and scaling parameters"=w341:T22, "Error Out"=w329:errorcluster)  [unwired: 6 in]
        n169 = call <vilib>:"Picture to Pixmap.vi"("picture"=w311) -> ("image data"=w318:T21)  [unwired: 9 in, 1 out]
        n170 = call <vilib>:"Unflatten Pixmap.vi"("image data"=w318) -> ("24-bit pixmap"=w317:u32[][])  [unwired: 4 in, 6 out]
        n171 = for {
          tunnel: w319 -> [w404] mode=indexing
          tunnel: w317 -> [w403] mode=indexing
          tunnel: [w402] -> w316 mode=indexing
          n172 = for {
            tunnel: w404 -> [w407] mode=indexing
            tunnel: w403 -> [w406] mode=indexing
            tunnel: [w405] -> w402 mode=indexing
            n173 = Greater Than 0?(x=w407) -> (x > 0?=w408:bool)
            n174 = Select(t=w407, s=w408, f=w406) -> (s? t:f=w405:u32)
          }
        }
        n175 = call <vilib>:"Flatten Pixmap.vi"("24-bit pixmap"=w316) -> ("image data"=w315:T21)  [unwired: 10 in]
        n176 = call <vilib>:"Draw Flattened Pixmap.vi"("image data"=w315) -> ("new picture"=w314:picture)  [unwired: 8 in]
        n177 = global write "SW_Globals.vi" "Density map"(w314) -> ()
        n178 = property class="Arr (strict)"(reference=w362, error in=w329) -> (reference out=w360:refnum<vi>, error out=w359:errorcluster, "Value"=w363:i32[])
        n179 = global write "SW_Globals.vi" "Diagram"(w311) -> ()
        n180 = Array Size(array=w363) -> (size(s)=w365:i32)
        n181 = global write "SW_Globals.vi" "Diagram no zones"(w301) -> ()
        n182 = global write "SW_Globals.vi" "Array of the segment to color correspondences"(w343) -> ()
        n183 = global write "SW_Globals.vi" "Array of the pixel to color correspondences"(w342) -> ()
        n184 = Unbundle By Name(w341) -> ("Pixels per mm"=w309:dbl)
        n185 = for {
          tunnel: w313 -> [w401] mode=indexing
          tunnel: w312 -> [w400] mode=indexing
          tunnel: [w395] -> w305 mode=indexing
          tunnel: w309 -> [w398]
          tunnel: w306 -> [w394]
          n186 = Multiply(x=w398, y=w401) -> (x*y=w397:dbl)
          n187 = Multiply(x=w398, y=w400) -> (x*y=w396:dbl)
          n188 = Bundle(w397, w396) -> (w399:cluster{dbl, dbl})  [unwired: 1 in]
          n189 = Add(x=w399, y=w394) -> (x+y=w395:cluster{dbl, dbl})
        }
        n190 = call <vilib>:"Draw Multiple Lines.vi"("picture"=w311, "line endpoints"=w305, "color(black)"="Full trace color", "pen"=w303) -> ("new picture"=w310:picture)  [unwired: 5 in]
        n191 = global write "SW_Globals.vi" "Full track with zones"(w310) -> ()
        n192 = call <vilib>:"Draw Multiple Lines.vi"("picture"=w301, "line endpoints"=w305, "color(black)"="Full trace color", "pen"=w303) -> ("new picture"=w302:picture)  [unwired: 5 in]
        n193 = global write "SW_Globals.vi" "Full track with no zones"(w302) -> ()
        n194 = Initialize Array(0 ("element"), w365) -> (w361:i32[])
        n195 = property class="Arr (strict)"(reference=w360, error in=w359, "Value"=w361) -> ()  [unwired: 2 out]
        n196 = local write "Pixels per mm"(w309) -> ()
      }
    }
  }
  n197 = while "This loop is all about temporary data processing and streaming to the interface part" {
    tunnel: w5 -> [w435]
    tunnel: w3 -> [w434]
    tunnel: [w420] -> w14
    i -> [w432]
    stop <- w429 stop-if-true
    w433 = u32 23 ("millisecond multiple")
    n198 = Unbundle By Name(w435) -> ("Complete stop"=w436:refnum<notifier>, "Play/Pause status"=w427:refnum<notifier>)
    n199 = Wait Until Next ms Multiple(millisecond multiple=w433) -> ()  [unwired: 1 out]
    n200 = flat-sequence {
      tunnel: w435 -> [w446]
      tunnel: w433 -> [w445]
      tunnel: w432 -> [w444]
      tunnel: w430 -> [w443]
      tunnel: w428 -> [w442]
      tunnel: [w441] -> w426
      tunnel: w424 -> [w440]
      tunnel: w423 -> [w439]
      tunnel: w421 -> [w438]
      tunnel: [w437] -> w420
      tunnel: w427 -> [w511]
      tunnel: w426 -> [w510]
      tunnel: [w509] -> w425
      frame #0 {
        n201 = case shown="\"Play\"" w440 {
          tunnel: w446 -> [_ w489]
          tunnel: w445 -> [_ w488]
          tunnel: w444 -> [_ w487]
          tunnel: w443 -> [_ w486]
          tunnel: w442 -> [_ w483]
          tunnel: [w447 w468] -> w441
          tunnel: w439 -> [w447 w479]
          tunnel: w438 -> [_ w482]
          tunnel: [_ w476] -> w437
          frame "Pause", Default {
          }
          frame "Play" {
            n202 = property on="Bridge swap" class="Bool (strict)"(error in=w479) -> (error out=w478:errorcluster, "Value"=w477:bool)  [unwired: 1 in, 1 out]
            n203 = local read "Pixels per mm"() -> (w480:dbl)
            n204 = property on="Diagram at recording" class="Pict"() -> ("Bounds"=w481:T14)  [unwired: 2 in, 2 out]
            n205 = call "FL_Preprocess_and_save_incrementally.vi"("Temporary file output path"=w483, "Loop iteration"=w487, "Mouse face dir. swap"=w477, "Loop speed in ms"=w488, "Save every N seconds"=u32 8, "error in (no error)"=w478, "Filter type"="Data filtering", "Sensor read input"=w486, "Offset"="Vertical offset", "Pixels per mm"=w480, "Data flow controls in"=w489, "Diagram at recording bounds"=w481, "Sensor board size"=w482) -> ("Eff. save interval"=→"Eff. save interval":sgl, "Latest sensor output (decoded)"=w459:string[][], "Fire TTL"=w466:bool, "TTL out N"=w465:u8, "Current TTL status"=w457:u8, "error out"=w469:errorcluster)  [unwired: 1 in]
            "Current TTL status" <- w457
            n206 = Index Array "TTL inputs"(array=w459, index (col)=14) -> (element=w460:string[])  [unwired: 1 in]
            n207 = property on="Start/Stop in config" class="DigNum (strict)"() -> ("Value"=w463:u32)  [unwired: 2 in, 2 out]
            n208 = Decimal String To Number(string=w460, default (0L)=u8 0 ("default (0 I32)")) -> (number=w464:u8[])  [unwired: 1 in, 1 out]
            n209 = call <extravilib>:"Write.vi"("size (1)"=5, "element"=w459) -> ("channel"=w476:T23)  [unwired: 7 in, 2 out]
            n210 = Greater Than 0?(x=w463) -> (x > 0?=w467:bool)
            n211 = Search 1D Array(1D array=w464, element=w463) -> (index of element=w462:i32)  [unwired: 1 in]
            n212 = Greater Or Equal To 0?(x=w462) -> (x >= 0?=w461:bool)
            n213 = And(x=w467, y=w461) -> (x .and. y?=w472:bool)
            n214 = case shown="True" w472 {
              tunnel: w460 -> [_ w508]
              frame False {
              }
              frame True {
                n215 = call "FL_Get_TTL_in_pulse_length.vi"("Latest sensor input (decoded)"=w508) -> ("TTL pulse length, ms"=w507:u32)
                n216 = global read "SW_Globals.vi" "TTL recording start signal has been successfully reset"() -> (w498:bool)
                n217 = global read "SW_Globals.vi" "Recording has been started with TTL"() -> (w501:bool)
                n218 = global read "SW_Globals.vi" "Recording has been stopped with TTL"() -> (w495:bool)
                n219 = feedback #1(FALSE) -> (w504:bool)
                n220 = Not(x=w504) -> (.not. x?=w505:bool)
                n221 = Greater Or Equal?(x=w507, y=u32 225) -> (x >= y?=w497:bool)
                "TTL is long enough" <- w497
                n222 = And(x=w505, y=w497) -> (x .and. y?=w502:bool)
                n223 = Not(x=w497) -> (.not. x?=w500:bool)
                n224 = And(x=w501, y=w500) -> (x .and. y?=w499:bool)
                n225 = Or(x=w502, y=w501) -> (x .or. y?=w494:bool)
                "Started" <- w494
                n226 = feedback-in #1(w494) -> ()
                n227 = Or(x=w498, y=w499) -> (x .or. y?=w493:bool)
                "Reset starting pulse" <- w493
                n228 = global write "SW_Globals.vi" "TTL recording start signal has been successfully reset"(w493) -> ()
                n229 = global write "SW_Globals.vi" "Recording has been started with TTL"(w494) -> ()
                n230 = Compound Arithmetic op=AND(w493, w494, w497) -> (w496:bool)
                n231 = Or(x=w496, y=w495) -> (x .or. y?=w492:bool)
                "Stopped" <- w492
                n232 = Not(x=w492) -> (.not. x?=w491:bool)
                n233 = global write "SW_Globals.vi" "Recording has been stopped with TTL"(w492) -> ()
                n234 = Compound Arithmetic op=AND(w494, w493, w491) -> (w490:bool)
                "Record" <- w490
                n235 = property on="Record/Stop" class="Bool (strict)"("Value"=w490) -> ()  [unwired: 2 in, 2 out]
                n236 = property on="TTL REC" class="Bool (strict)"("Value"=w490) -> ()  [unwired: 2 in, 2 out]
              }
            }
            n237 = Number To Boolean Array(number=w457) -> (Boolean array=w450:bool[])
            n238 = Index Array(array=w450, index=0) -> (element=→"TTL IO 1 (recording)":bool)
            n239 = Index Array(array=w450, index=1) -> (element=→"TTL IO 2 (recording)":bool)
            n240 = Index Array(array=w450, index=2) -> (element=→"TTL IO 3 (recording)":bool)
            n241 = Index Array(array=w450, index=3) -> (element=→"TTL IO 4 (recording)":bool)
            n242 = global read "SW_Globals.vi" "VISA resource name out"() -> (w470:refnum<visa-resource-name>)
            n243 = call "SW_Fire_TTL_during_the_acquisition_universal.vi"("error in (no error)"=w469, "Serial Port In"=w470, "TTL port(s) config to fire"=w465, "Fire TTL"=w466) -> ("error out"=w468:errorcluster)  [unwired: 7 in]
          }
        }
      }
      frame #1 {
        n244 = Get Notifier Status(notifier=w511, error in (no error)=w510) -> (current notification=w509:string)  [unwired: 4 out]
      }
    }
    n245 = Flush Queue(queue=w434) -> (remaining elements=w430:T24, error out=w423:errorcluster)  [unwired: 1 in, 1 out]
    n246 = local read "Board size"() -> (w421:string)
    n247 = global read "SW_Globals.vi" "Cluster of paths"() -> (w431:T18)
    n248 = Get Notifier Status(notifier=w436) -> (current notification=w429:bool)  [unwired: 1 in, 4 out]
    n249 = Unbundle By Name(w431) -> ("Temporary file output path"=w428:path)
    n250 = feedback-in #2(w425) -> ()
    n251 = feedback #2("Pause" ("String")) -> (w424:string)
  }
  n252 = flat-sequence "Things to run at the very beginning of the program" {
    tunnel: [w558] -> w19
    tunnel: [w570] -> w1
    frame #0 {
      w516 = T8 [{"Numeric Control"=9868950, "Numeric Control"=15790320}, {"Numeric Control"=8388608, "Numeric Control"=8388608}, {"Numeric Control"=4934475, "Numeric Control"=7895160}, {"Numeric Control"=994319, "Numeric Control"=1657881}]  # TTL IO In colors
      w517 = T8 [{"Numeric Control"=9868950, "Numeric Control"=15790320}, {"Numeric Control"=1988894, "Numeric Control"=3381555}, {"Numeric Control"=4934475, "Numeric Control"=7895160}, {"Numeric Control"=994319, "Numeric Control"=1657881}]  # TTL IO Out colors
      w545 = T9."Enabled" ("Disabled")
      w580 = FALSE ("Recording has been started with TTL")
      w598 = "Researcher"
      w621 = enum32{"Settings", "Recording", "Analysis"}."Settings" ("Main tab control")
      w628 = enum32{"Settings", "Recording", "Analysis"}."Analysis" ("Main tab control")
      w636 = enum32{"Settings", "Recording", "Analysis"}."Recording" ("Main tab control")
      n253 = property on="IO parameters string" class="Str"(error in="error in (no error)", "Value"="[12,1,1,0,0,0]" ("IO parameters string")) -> (error out=w541:errorcluster)  [unwired: 1 in, 1 out]
      n254 = property on="Pane" class="Pane"(error in=w541) -> (error out=w554:errorcluster, "Decos[]"=w555:refnum<vi>[])  [unwired: 1 in, 1 out]
      n255 = for {
        tunnel: w555 -> [w652] mode=indexing
        tunnel: w554 -> [w650]
        tunnel: [w649] -> w547
        n256 = property class="Decor"(reference=w652, error in=w650, "Visible"=FALSE) -> (error out=w649:errorcluster)  [unwired: 1 out]
      }
      n257 = property on="Vertical offset" class="DigNum (strict)"(error in=w547, "DisabledEnum"=w545) -> (error out=w546:errorcluster)  [unwired: 1 in, 1 out]
      n258 = property on="Back to Settings" class="Bool"(error in=w546, "DisabledEnum"=w545, "Visible"=FALSE) -> (error out=w557:errorcluster)  [unwired: 1 in, 1 out]
      n259 = property class="App"() -> ("App.Kind"=w596:T28)  [unwired: 2 in, 2 out]
      n260 = property on="Ready" class="Bool (strict)"(error in=w557, "Value"=FALSE ("Ready")) -> (error out=w544:errorcluster)  [unwired: 1 in, 1 out]
      n261 = case shown="\"invalid app kind\", Default" w596 {
        tunnel: [w732 w733] -> w588
        frame "invalid app kind", Default {
          n262 = call <vilib>:"Application Directory.vi"() -> ("Application Directory"=w732:path)
          "Application Directory" <- w732
        }
        frame "Development System" {
          n263 = Current VI's Path() -> (path=w734:path)
          n264 = Strip Path(path=w734) -> (stripped path=w733:path)  [unwired: 1 out]
        }
      }
      n265 = property on="Start Tracking button" class="Bool"(error in=w544, "DisabledEnum"=T9."Disabled and Grayed Out" ("Disabled")) -> (error out=w579:errorcluster)  [unwired: 1 in, 1 out]
      n266 = call "SW_Generate_Color_Ramp.vi"() -> ("Colors array"=w604:u32[])  [unwired: 2 in]
      n267 = property on="Stim. setup" class="RadioBtnsControl (strict)"(error in=w579, "Value"=T25."No Selection" ("Stimulus")) -> (error out=w578:errorcluster)  [unwired: 1 in, 1 out]
      n268 = property on="Pane" class="Pane"("Origin"=T27 {"Horizontal"=0, "Vertical"=0}) -> ()  [unwired: 2 in, 2 out]
      n269 = global write "SW_Globals.vi" "Color ramp array"(w604) -> ()
      n270 = Build Path(base path=w588, name or relative path=path "Tracker_settings.tcf") -> (appended path=w582:path)
      "Path to the settings file" <- w582
      n271 = global read "SW_Globals.vi" "Cluster of paths"() -> (w583:T18)
      n272 = global write "SW_Globals.vi" "Recording start timestamp"(timestamp(0 s since 1904-01-01) ("Recording start timestamp")) -> ()
      n273 = call <vilib>:"Open Config Data.vi"("error in (no error)"=w578, "create file if necessary (T)"=FALSE, "configuration file path"=w582) -> ("error out"=w646:errorcluster, "refnum"=w645:T3)  [unwired: 6 in, 1 out]
      n274 = Bundle By Name(cluster=w583, "Path to the settings file"=w582) -> (w581:T18)
      n275 = call <vilib>:"Get Key Names.vi"("section"="Users", "error in (no error)"=w646, "refnum"=w645) -> ("error out"=w642:errorcluster, "key names"=w638:string[], "refnum out"=w643:T3)  [unwired: 5 in, 1 out]
      n276 = call <vilib>:"Read Key (U32).vi"("section"="Defaults", "error in (no error)"=w642, "key"="Default User", "refnum"=w643) -> ("error out"=w617:errorcluster, "value"=w639:u32, "refnum out"=w616:T3)  [unwired: 4 in, 1 out]
      n277 = global write "SW_Globals.vi" "Cluster of paths"(w581) -> ()
      n278 = Index Array(array=w638, index=w639) -> ()  [unwired: 1 out]
      n279 = call "SW_Load_settings_to_main_tab.vi"("Refnum in"=w616, "User Name"=w598, "error in (no error)"=w617) -> ("VISA resource name"=w558:string, "Vertical offset"=w548:dbl, "Midfield segments outer radius, mm"=w605:i32, "Cage diameter, mm"=w612:i32, "Midfield segments starting angle"=w607:i32, "Border segments starting angle"=w608:i32, "Stimulus presets array"=w536:T19, "IO parameters cluster"=w528:T12, "Refnum out"=→"Settings file refnum out":T3, "Amount of midfield segments"=w614:i32, "Mouse snout orientation swap?"=w586:bool, "Amount of border segments"=w613:i32, "Center segment outer radius, mm"=w606:i32, "error out"=w532:errorcluster)  [unwired: 11 in]
      "Port" <- w558
      n280 = local write "Vertical offset"(w548) -> ()
      n281 = Unbundle By Name(w528) -> ("SYNC configuration"=w535:u16)
      n282 = local write "Radius, mm CENTER"(w606) -> ()
      n283 = local write "Radius, mm MIDFIELD"(w605) -> ()
      n284 = local write "Cage diameter, mm"(w612) -> ()
      n285 = local write "Starting angle BORDER"(w608) -> ()
      n286 = local write "N segments MIDFIELD"(w614) -> ()
      n287 = local write "N segments BORDER"(w613) -> ()
      n288 = local write "Starting angle MIDFIELD"(w607) -> ()
      n289 = call "SW_get_config_of_Zones_and_IO.vi"("Sync parameters cluster input"=w528) -> ("Zones out config bin"=w527:bool[], "Ports IO config (OUT is FALSE)"=w525:bool[])  [unwired: 1 out]
      n290 = property on="Bridge swap" class="Bool (strict)"(error in=w532, "DisabledEnum"=T9."Enabled" ("Disabled"), "Value"=w586) -> (error out=w585:errorcluster)  [unwired: 1 in, 1 out]
      n291 = call "SW_get_config_for_Start_Stop_pulses.vi"("Sync parameters cluster input"=w528) -> ("Start/Stop out pulses config"=→"Start/Stop out pulses config":u32, "Start/Stop in config"=→"Start/Stop in config":u32, "Start/Stop in config bin"=w530:bool[], "Start/Stop out pulses config bin"=w529:bool[])
      n292 = call "SW_Gen_Available_TTL_outputs_array.vi"("SYNC configuration"=w535) -> ("Available TTL outputs array"=w534:cluster{"String":string, "Value":i32}[])
      n293 = global write "SW_Globals.vi" "IO parameters cluster"(w528) -> ()
      n294 = global write "SW_Globals.vi" "Start/Stop out pulses config bin"(w529) -> ()
      n295 = property on="TTL out" class="Ring (strict)"("StringsAndValues[]"=w534) -> ()  [unwired: 2 in, 2 out]
      n296 = global write "SW_Globals.vi" "Zones out config bin"(w527) -> ()
      n297 = global write "SW_Globals.vi" "Start/Stop in config bin"(w530) -> ()
      n298 = global write "SW_Globals.vi" "IO ports config"(w525) -> ()
      n299 = call "SW_get_IO_ports_representation.vi"("Sync parameters cluster input"=w528) -> ("IO status indicator"=→"IO status indicator":T4)
      n300 = property on="Main tab control" class="TabCtl (strict)"(error in=w585, "Value"=w636) -> (error out=w633:errorcluster, "Pages"=w637:refnum<vi>[])  [unwired: 1 in, 1 out]
      n301 = Index Array(array=w525, index=0) -> (element=w521:bool)
      n302 = Index Array(array=w525, index=1) -> (element=w520:bool)
      n303 = Index Array(array=w525, index=2) -> (element=w519:bool)
      n304 = Index Array(array=w525, index=3) -> (element=w518:bool)
      n305 = To Long Integer(number=w636) -> (32bit integer=w635:i32)
      n306 = Select(t=w516, s=w521, f=w517) -> (s? t:f=w515:T8)
      n307 = Select(t=w516, s=w520, f=w517) -> (s? t:f=w514:T8)
      n308 = Select(t=w516, s=w518, f=w517) -> (s? t:f=w512:T8)
      n309 = Index Array(array=w637, index=w635) -> (element=w634:refnum<vi>)
      n310 = Select(t=w516, s=w519, f=w517) -> (s? t:f=w513:T8)
      n311 = property class="Page"(reference=w634, error in=w633, "PageEnb"=T26."Page Disabled & Grayed" ("Page Enabled State")) -> (error out=w631:errorcluster)  [unwired: 1 out]
      n312 = property on="TTL IO 1 (recording)" class="Bool (strict)"("Colors [4]"=w515) -> ()  [unwired: 2 in, 2 out]
      n313 = property on="TTL IO 3 (recording)" class="Bool (strict)"("Colors [4]"=w513) -> ()  [unwired: 2 in, 2 out]
      n314 = property on="TTL IO 2 (recording)" class="Bool (strict)"("Colors [4]"=w514) -> ()  [unwired: 2 in, 2 out]
      n315 = property on="TTL IO 1 (analysis)" class="Bool"("Colors [4]"=w515) -> ()  [unwired: 2 in, 2 out]
      n316 = property on="TTL IO 4 (recording)" class="Bool (strict)"("Colors [4]"=w512) -> ()  [unwired: 2 in, 2 out]
      n317 = property on="Main tab control" class="TabCtl (strict)"(error in=w631, "Value"=w628) -> (error out=w630:errorcluster, "Pages"=w629:refnum<vi>[])  [unwired: 1 in, 1 out]
      n318 = To Long Integer(number=w628) -> (32bit integer=w627:i32)
      n319 = property on="TTL IO 3 (analysis)" class="Bool"("Colors [4]"=w513) -> ()  [unwired: 2 in, 2 out]
      n320 = property on="TTL IO 2 (analysis)" class="Bool"("Colors [4]"=w514) -> ()  [unwired: 2 in, 2 out]
      n321 = Index Array(array=w629, index=w627) -> (element=w626:refnum<vi>)
      n322 = property on="TTL IO 4 (analysis)" class="Bool"("Colors [4]"=w512) -> ()  [unwired: 2 in, 2 out]
      n323 = global write "SW_Globals.vi" "TTL recording start signal has been successfully reset"(w580) -> ()
      n324 = property class="Page"(reference=w626, error in=w630, "PageEnb"=T26."Page Disabled & Grayed" ("Page Enabled State")) -> (error out=w618:errorcluster)  [unwired: 1 out]
      n325 = global write "SW_Globals.vi" "Recording has been stopped with TTL"(w580) -> ()
      n326 = global write "SW_Globals.vi" "Recording has been started with TTL"(w580) -> ()
      n327 = property on="Main tab control" class="TabCtl (strict)"(error in=w618, "Value"=w621) -> (error out=w619:errorcluster, "Pages"=w620:refnum<vi>[])  [unwired: 1 in, 1 out]
      n328 = To Long Integer(number=w621) -> (32bit integer=w622:i32)
      n329 = for {
        N: 14 -> [_]
        tunnel: w536 -> [w656] mode=indexing
        tunnel: [w654] -> w559 mode=indexing if=w653
        i -> [w655]
        n330 = Unbundle By Name(w656) -> ("Stim. has been set"=w653:bool)
        n331 = case shown="1" w655 {
          tunnel: w653 -> [_ w657 w662 w667 w672 w677 w682 w687 w692 w697 w703 w707 w713 w718]
          frame 0, Default {
          }
          frame 1 {
            n332 = property on="Colors for Stim. setup" class="Arr (strict)"() -> ("Value"=w660:T1)  [unwired: 2 in, 2 out]
            n333 = Select(t=w660, s=w657, f=T8 [{"Numeric Control"=12369084, "Numeric Control"=12369084}, {"Numeric Control"=6603023, "Numeric Control"=6603023}, {"Numeric Control"=1976113, "Numeric Control"=1976113}, {"Numeric Control"=2575993, "Numeric Control"=2575993}] ("Colors [4] 2")) -> (s? t:f=w658:T8)
            n334 = property on="Zone 01" class="Bool (strict)"("Colors [4]"=w658, "Value"=FALSE) -> ()  [unwired: 2 in, 2 out]
          }
          frame 2 {
            n335 = property on="Colors for Stim. setup" class="Arr (strict)"() -> ("Value"=w665:T1)  [unwired: 2 in, 2 out]
            n336 = Select(t=w665, s=w662, f=T8 [{"Numeric Control"=12369084, "Numeric Control"=12369084}, {"Numeric Control"=6603023, "Numeric Control"=6603023}, {"Numeric Control"=1976113, "Numeric Control"=1976113}, {"Numeric Control"=2575993, "Numeric Control"=2575993}] ("Colors [4] 2")) -> (s? t:f=w663:T8)
            n337 = property on="Zone 02" class="Bool (strict)"("Colors [4]"=w663, "Value"=FALSE) -> ()  [unwired: 2 in, 2 out]
          }
          frame 3 {
            n338 = property on="Colors for Stim. setup" class="Arr (strict)"() -> ("Value"=w670:T1)  [unwired: 2 in, 2 out]
            n339 = Select(t=w670, s=w667, f=T8 [{"Numeric Control"=12369084, "Numeric Control"=12369084}, {"Numeric Control"=6603023, "Numeric Control"=6603023}, {"Numeric Control"=1976113, "Numeric Control"=1976113}, {"Numeric Control"=2575993, "Numeric Control"=2575993}] ("Colors [4] 2")) -> (s? t:f=w668:T8)
            n340 = property on="Zone 03" class="Bool (strict)"("Colors [4]"=w668, "Value"=FALSE) -> ()  [unwired: 2 in, 2 out]
          }
          frame 4 {
            n341 = property on="Colors for Stim. setup" class="Arr (strict)"() -> ("Value"=w675:T1)  [unwired: 2 in, 2 out]
            n342 = Select(t=w675, s=w672, f=T8 [{"Numeric Control"=12369084, "Numeric Control"=12369084}, {"Numeric Control"=6603023, "Numeric Control"=6603023}, {"Numeric Control"=1976113, "Numeric Control"=1976113}, {"Numeric Control"=2575993, "Numeric Control"=2575993}] ("Colors [4] 2")) -> (s? t:f=w673:T8)
            n343 = property on="Zone 04" class="Bool (strict)"("Colors [4]"=w673, "Value"=FALSE) -> ()  [unwired: 2 in, 2 out]
          }
          frame 5 {
            n344 = property on="Colors for Stim. setup" class="Arr (strict)"() -> ("Value"=w680:T1)  [unwired: 2 in, 2 out]
            n345 = Select(t=w680, s=w677, f=T8 [{"Numeric Control"=12369084, "Numeric Control"=12369084}, {"Numeric Control"=6603023, "Numeric Control"=6603023}, {"Numeric Control"=1976113, "Numeric Control"=1976113}, {"Numeric Control"=2575993, "Numeric Control"=2575993}] ("Colors [4] 2")) -> (s? t:f=w678:T8)
            n346 = property on="Zone 05" class="Bool (strict)"("Colors [4]"=w678, "Value"=FALSE) -> ()  [unwired: 2 in, 2 out]
          }
          frame 6 {
            n347 = property on="Colors for Stim. setup" class="Arr (strict)"() -> ("Value"=w685:T1)  [unwired: 2 in, 2 out]
            n348 = Select(t=w685, s=w682, f=T8 [{"Numeric Control"=12369084, "Numeric Control"=12369084}, {"Numeric Control"=6603023, "Numeric Control"=6603023}, {"Numeric Control"=1976113, "Numeric Control"=1976113}, {"Numeric Control"=2575993, "Numeric Control"=2575993}] ("Colors [4] 2")) -> (s? t:f=w683:T8)
            n349 = property on="Zone 06" class="Bool (strict)"("Colors [4]"=w683, "Value"=FALSE) -> ()  [unwired: 2 in, 2 out]
          }
          frame 7 {
            n350 = property on="Colors for Stim. setup" class="Arr (strict)"() -> ("Value"=w690:T1)  [unwired: 2 in, 2 out]
            n351 = Select(t=w690, s=w687, f=T8 [{"Numeric Control"=12369084, "Numeric Control"=12369084}, {"Numeric Control"=6603023, "Numeric Control"=6603023}, {"Numeric Control"=1976113, "Numeric Control"=1976113}, {"Numeric Control"=2575993, "Numeric Control"=2575993}] ("Colors [4] 2")) -> (s? t:f=w688:T8)
            n352 = property on="Zone 07" class="Bool (strict)"("Colors [4]"=w688, "Value"=FALSE) -> ()  [unwired: 2 in, 2 out]
          }
          frame 8 {
            n353 = property on="Colors for Stim. setup" class="Arr (strict)"() -> ("Value"=w695:T1)  [unwired: 2 in, 2 out]
            n354 = Select(t=w695, s=w692, f=T8 [{"Numeric Control"=12369084, "Numeric Control"=12369084}, {"Numeric Control"=6603023, "Numeric Control"=6603023}, {"Numeric Control"=1976113, "Numeric Control"=1976113}, {"Numeric Control"=2575993, "Numeric Control"=2575993}] ("Colors [4] 2")) -> (s? t:f=w693:T8)
            n355 = property on="Zone 08" class="Bool (strict)"("Colors [4]"=w693, "Value"=FALSE) -> ()  [unwired: 2 in, 2 out]
          }
          frame 9 {
            n356 = property on="Colors for Stim. setup" class="Arr (strict)"() -> ("Value"=w700:T1)  [unwired: 2 in, 2 out]
            n357 = Select(t=w700, s=w697, f=T8 [{"Numeric Control"=12369084, "Numeric Control"=12369084}, {"Numeric Control"=6603023, "Numeric Control"=6603023}, {"Numeric Control"=1976113, "Numeric Control"=1976113}, {"Numeric Control"=2575993, "Numeric Control"=2575993}] ("Colors [4] 2")) -> (s? t:f=w698:T8)
            n358 = property on="Zone 09" class="Bool (strict)"("Colors [4]"=w698, "Value"=FALSE) -> ()  [unwired: 2 in, 2 out]
          }
          frame 10 {
            n359 = property on="Colors for Stim. setup" class="Arr (strict)"() -> ("Value"=w705:T1)  [unwired: 2 in, 2 out]
            n360 = Select(t=w705, s=w703, f=T8 [{"Numeric Control"=12369084, "Numeric Control"=12369084}, {"Numeric Control"=6603023, "Numeric Control"=6603023}, {"Numeric Control"=1976113, "Numeric Control"=1976113}, {"Numeric Control"=2575993, "Numeric Control"=2575993}] ("Colors [4] 2")) -> (s? t:f=w702:T8)
            n361 = property on="Zone 10" class="Bool (strict)"("Colors [4]"=w702, "Value"=FALSE) -> ()  [unwired: 2 in, 2 out]
          }
          frame 11 {
            n362 = property on="Colors for Stim. setup" class="Arr (strict)"() -> ("Value"=w710:T1)  [unwired: 2 in, 2 out]
            n363 = Select(t=w710, s=w707, f=T8 [{"Numeric Control"=12369084, "Numeric Control"=12369084}, {"Numeric Control"=6603023, "Numeric Control"=6603023}, {"Numeric Control"=1976113, "Numeric Control"=1976113}, {"Numeric Control"=2575993, "Numeric Control"=2575993}] ("Colors [4] 2")) -> (s? t:f=w709:T8)
            n364 = property on="Zone 11" class="Bool (strict)"("Colors [4]"=w709, "Value"=FALSE) -> ()  [unwired: 2 in, 2 out]
          }
          frame 12 {
            n365 = property on="Colors for Stim. setup" class="Arr (strict)"() -> ("Value"=w715:T1)  [unwired: 2 in, 2 out]
            n366 = Select(t=w715, s=w713, f=T8 [{"Numeric Control"=12369084, "Numeric Control"=12369084}, {"Numeric Control"=6603023, "Numeric Control"=6603023}, {"Numeric Control"=1976113, "Numeric Control"=1976113}, {"Numeric Control"=2575993, "Numeric Control"=2575993}] ("Colors [4] 2")) -> (s? t:f=w712:T8)
            n367 = property on="Zone 12" class="Bool (strict)"("Colors [4]"=w712, "Value"=FALSE) -> ()  [unwired: 2 in, 2 out]
          }
          frame 13 {
            n368 = property on="Colors for Stim. setup" class="Arr (strict)"() -> ("Value"=w720:T1)  [unwired: 2 in, 2 out]
            n369 = Select(t=w720, s=w718, f=T8 [{"Numeric Control"=12369084, "Numeric Control"=12369084}, {"Numeric Control"=6603023, "Numeric Control"=6603023}, {"Numeric Control"=1976113, "Numeric Control"=1976113}, {"Numeric Control"=2575993, "Numeric Control"=2575993}] ("Colors [4] 2")) -> (s? t:f=w717:T8)
            n370 = property on="Zone 13" class="Bool (strict)"("Colors [4]"=w717, "Value"=FALSE) -> ()  [unwired: 2 in, 2 out]
          }
        }
        n371 = To Unsigned Byte Integer(number=w655) -> (unsigned 8bit integer=w654:u8)
      }
      n372 = global write "SW_Globals.vi" "Regions to track"(u8[] [] ("Regions to track")) -> ()
      n373 = Index Array(array=w620, index=w622) -> (element=w623:refnum<vi>)
      n374 = property class="Page"(reference=w623, error in=w619, "PageEnb"=T26."Page Enabled" ("Page Enabled State")) -> (error out=w611:errorcluster)  [unwired: 1 out]
      n375 = property on="Record/Stop" class="Bool (strict)"(error in=w611, "Value"=FALSE ("Record/Stop")) -> (error out=w610:errorcluster)  [unwired: 1 in, 1 out]
      n376 = Flatten To String(anything="Zones presence indicator") -> (data string=w593:string)  [unwired: 3 in, 2 out]
      n377 = String Length(string=w593) -> (length=w591:i32)
      n378 = global write "SW_Globals.vi" "Regions to track"(w559) -> ()
      n379 = property on="Play/Pause" class="Bool (strict)"(error in=w610, "Value"=FALSE ("Play/Pause")) -> (error out=w587:errorcluster)  [unwired: 1 in, 1 out]
      n380 = property on="Stimulus presets" class="Arr (strict)"("Value"=w536) -> (error out=w565:errorcluster)  [unwired: 2 in, 1 out]
      n381 = global write "SW_Globals.vi" "Stimulus presets"(w536) -> ()
      n382 = Initialize Array(FALSE, w591) -> (→"Zones presence array":bool[])
      n383 = Initialize Array(0, w591) -> (→"Zones allocation array":i32[])
      n384 = property on="Stimulus presets" class="Arr (strict)"(error in=w565, "Index Values"=u32[] [0], "DisabledEnum"=T9."Disabled and Grayed Out" ("Disabled")) -> (error out=w540:errorcluster)  [unwired: 1 in, 1 out]
      n385 = property on="Record timestamp" class="DigNum (strict)"(error in=w587, "DisabledEnum"=T9."Disabled and Grayed Out" ("Disabled"), "Value"=0.0 ("Record timestamp")) -> (error out=w570:errorcluster)  [unwired: 1 in, 1 out]
      n386 = property on="Data filtering" class="Ring (strict)"(error in=w540, "DisabledEnum"=T9."Enabled" ("Disabled")) -> (error out=w539:errorcluster)  [unwired: 1 in, 1 out]
      n387 = property on="N segments BORDER" class="DigNum (strict)"(error in=w539) -> (error out=w571:errorcluster, "Value"=w575:u8)  [unwired: 1 in, 1 out]
      n388 = property on="N segments MIDFIELD" class="DigNum (strict)"(error in=w571) -> (error out=w562:errorcluster, "Value"=w574:u8)  [unwired: 1 in, 1 out]
      n389 = property on="Stim. setup" class="RadioBtnsControl (strict)"(error in=w562) -> (error out=w568:errorcluster, "Controls[]"=w573:refnum<vi>[])  [unwired: 1 in, 1 out]
      n390 = Compound Arithmetic op=ADD(w575, w574, u8 1 ("value")) -> (w572:u8)
      n391 = for {
        tunnel: w573 -> [w731] mode=indexing
        tunnel: w572 -> [w727]
        tunnel: w568 -> [w722]
        tunnel: [w724] -> w567
        i -> [w723]
        n392 = Increment(x=w723) -> (x+1=w726:i32)
        n393 = Greater Or Equal?(x=w727, y=w726) -> (x >= y?=w725:bool)
        n394 = Select(t=T9."Enabled" ("Disabled"), s=w725, f=T9."Disabled and Grayed Out") -> (s? t:f=w729:T9)
        n395 = property class="Ctl"(reference=w731, error in=w722, "DisabledEnum"=w729) -> (error out=w724:errorcluster)  [unwired: 1 out]
      }
      n396 = property on="Stim. setup" class="RadioBtnsControl (strict)"(error in=w567, "Value"=T6."No Selection" ("Stim. setup")) -> (error out=w553:errorcluster)  [unwired: 1 in, 1 out]
      n397 = property on="Pane" class="Pane"(error in=w553) -> ("Decos[]"=w552:refnum<vi>[])  [unwired: 1 in, 2 out]
      n398 = Index Array(array=w552, index=2) -> (element=w550:refnum<vi>)
      n399 = property class="Decor"(reference=w550, "Visible"=TRUE) -> ()  [unwired: 1 in, 2 out]
      "Current User" <- w598
    }
  }
  n400 = while "Loop where temporary files are transferred to permanent location and data saved" {
    tunnel: w5 -> [w760]
    tunnel: [w745] -> w13
    stop <- w746 stop-if-true
    n401 = flat-sequence {
      tunnel: w760 -> [w975]
      tunnel: [w975] -> w759
      tunnel: w759 -> [w976]
      tunnel: [w978] -> w757
      tunnel: [w977] -> w756
      tunnel: [w976] -> w758
      frame #0 {
        n402 = Wait (ms)(milliseconds to wait=u32 521) -> ()  [unwired: 1 out]
      }
      frame #1 {
        n403 = Unbundle By Name(w976) -> ("Path to the latest complete temp file"=w978:refnum<notifier>, "Temp file ready for processing"=w977:refnum<notifier>)
      }
    }
    n404 = Get Notifier Status(notifier=w756) -> (error out=w755:errorcluster)  [unwired: 1 in, 4 out]
    n405 = Get Notifier Status(notifier=w757, error in (no error)=w755) -> (current notification=w751:path)  [unwired: 4 out]
    n406 = feedback-in #3(w751) -> ()
    n407 = feedback #3(path "") -> (w753:path)
    n408 = local read "Starting angle MIDFIELD"() -> (w741:i16)
    n409 = local read "Starting angle BORDER"() -> (w743:i16)
    n410 = local read "N segments MIDFIELD"() -> (w742:u8)
    n411 = local read "Radius, mm MIDFIELD"() -> (w740:u16)
    n412 = local read "N segments BORDER"() -> (w744:u8)
    n413 = local read "Radius, mm CENTER"() -> (w738:u16)
    n414 = Not Equal?(x=w753, y=w751) -> (x != y?=w752:bool)
    n415 = Not Equal?(x=path "", y=w751) -> (x != y?=w750:bool)
    n416 = Bundle By Name(cluster=T29 {"N segments BORDER"=0, "Starting angle BORDER"=0, "N segments MIDFIELD"=0, "Starting angle MIDFIELD"=0, "Radius, mm MIDFIELD"=0, "Amount of central segments"=0, "Radius, mm CENTER"=0} ("output cluster 2"), "N segments BORDER"=w744, "Starting angle BORDER"=w743, "N segments MIDFIELD"=w742, "Starting angle MIDFIELD"=w741, "Radius, mm MIDFIELD"=w740, "Amount of central segments"=u8 1, "Radius, mm CENTER"=w738) -> (w737:T29)
    n417 = And(x=w750, y=w752) -> (x .and. y?=w747:bool)
    n418 = local read "Cage diameter, mm"() -> (w736:u16)
    n419 = global read "SW_Globals.vi" "Cluster of paths"() -> (w761:T18)
    n420 = case shown="True" w747 {
      tunnel: w761 -> [_ w778]
      tunnel: w758 -> [_ w777]
      tunnel: errorcluster {"status"=FALSE, "code"=0, "source"=""} ("error constant") -> [w763 w776]
      tunnel: w747 -> [_ w775]
      tunnel: w751 -> [_ w774]
      tunnel: [FALSE w770] -> w746
      tunnel: [w763 w769] -> w745
      tunnel: w737 -> [_ w765]
      tunnel: w736 -> [_ w764]
      frame False {
      }
      frame True {
        n421 = flat-sequence {
          tunnel: w774 -> [w819]
          tunnel: w775 -> [w818]
          tunnel: w778 -> [w803]
          tunnel: w776 -> [w817]
          tunnel: [w816] -> w782
          tunnel: w777 -> [w815]
          tunnel: [w815] -> w781
          tunnel: [w803] -> w768
          tunnel: w765 -> [w802]
          tunnel: w764 -> [w801]
          tunnel: w782 -> [w954]
          tunnel: [w954] -> w780
          tunnel: [w953] -> w779
          tunnel: w781 -> [w953]
          tunnel: w768 -> [w952]
          tunnel: [w952] -> w767
          tunnel: [w963] -> w771
          tunnel: [w966] -> w773
          tunnel: w780 -> [w962]
          tunnel: [w961] -> w772
          tunnel: w779 -> [w961]
          tunnel: w767 -> [w958]
          tunnel: [w958] -> w766
          frame #0 {
            n422 = Unbundle By Name(w803) -> ("Temporary csv output path"=w808:path, "Background picture output path"=w811:path, "Recording settings output path"=w810:path, "Final csv output path"=w809:path, "Path to the settings file"=w800:path)
            n423 = First Call?() -> (First Call?: T/F=w814:bool)
            n424 = case shown="True" w814 {
              selector: w814 -> [w820 w824]
              tunnel: [w823 w931] -> w807
              tunnel: w819 -> [w823 w931]
              tunnel: w808 -> [w821 w917]
              tunnel: w811 -> [_ w915]
              tunnel: w810 -> [_ w913]
              tunnel: w809 -> [_ w885]
              tunnel: w817 -> [w822 w882]
              tunnel: [w822 w881] -> w806
              tunnel: [w821 w880] -> w804
              tunnel: w802 -> [_ w841]
              tunnel: w801 -> [_ w839]
              tunnel: w800 -> [_ w860]
              tunnel: [w820 w824] -> w799
              frame False {
              }
              frame True {
                w859 = "Vertical offset" ("key")
                w852 = "Mouse snout orientation swap?" ("key")
                w825 = "Recording settings" ("key")
                n425 = Unbundle By Name(w841) -> ("N segments BORDER"=w840:u8, "Starting angle BORDER"=w838:i16, "N segments MIDFIELD"=w837:u8, "Starting angle MIDFIELD"=w836:i16, "Radius, mm MIDFIELD"=w835:u16, "Radius, mm CENTER"=w833:u16)
                n426 = Build Array("X1_raw", "Y1_raw", "X2_raw", "Y2_raw", "Absolute_timestamp", "Relative_timestamp", "R", "phi", "alpha", "X", "Y", "w", "Current_zone", "Zones_preference", "TTL_inputs", "TTL_outputs", "Frame_OK") -> (w918:string[])
                n427 = Bundle By Name(cluster=T15 {"Amount of border segments"=8, "Border segments starting angle"=0, "Amount of midfield segments"=4, "Midfield segments starting angle"=0, "Midfield segments outer radius, mm"=60, "Amount of central segments"=1, "Center segment outer radius, mm"=30, "Diameter of the cage, mm"=180, "R-gap between segments, mm"=10} ("Input cluster of parameters"), "Diameter of the cage, mm"=w839, "Amount of border segments"=w840, "Border segments starting angle"=w838, "Amount of midfield segments"=w837, "Midfield segments starting angle"=w836, "Midfield segments outer radius, mm"=w835, "Center segment outer radius, mm"=w833) -> (w834:T15)
                n428 = call-poly <vilib>:"Write Delimited Spreadsheet.vi"("file path (dialog if empty)"=w917, "1D data"=w918, "append to file? (new file:F)"=FALSE, "error in (no error)"=w882) -> ("new file path (Not A Path if cancelled)"=w880:path, "error out"=w847:errorcluster)  [unwired: 10 in]
                n429 = global read "SW_Globals.vi" "Regions to track"() -> (w844:u8[])
                n430 = call "SW_Generate_Segmented_Plot_v3.vi"("Draw Area Size"=cluster{"Width":dbl, "Height":dbl} {"Width"=1200.0, "Height"=1200.0}, "Regions to mark set"=w844, "Input cluster of parameters"=w834, "Error In"=w847) -> ("Zones layout output"=w845:picture, "Error Out"=w846:errorcluster)  [unwired: 6 in, 4 out]
                n431 = call <vilib>:"Picture to Pixmap.vi"("picture"=w845) -> ("image data"=w914:T21)  [unwired: 9 in, 1 out]
                n432 = local read "Current User"() -> (w888:string)
                n433 = call <vilib>:"Write PNG File.vi"("error in (no error)"=w846, "image data"=w914, "path to PNG file"=w915) -> ("error out"=w895:errorcluster)  [unwired: 7 in, 1 out]
                n434 = call <vilib>:"Open Config Data.vi"("error in (no error)"=w895, "configuration file path"=w913) -> ("refnum"=w893:T3)  [unwired: 7 in, 2 out]
                n435 = Strip Path(path=w885) -> (name=w884:string)  [unwired: 1 out]
                n436 = call <vilib>:"Write Key (String).vi"("section"=w825, "value"=w888, "key"="Researcher", "refnum"=w893) -> ("error out"=w890:errorcluster, "refnum out"=w892:T3)  [unwired: 5 in, 1 out]
                n437 = Unbundle By Name(w841) -> ("N segments MIDFIELD"=w879:u8, "N segments BORDER"=w878:u8, "Radius, mm CENTER"=w877:u16, "Radius, mm MIDFIELD"=w876:u16, "Starting angle MIDFIELD"=w875:i16, "Starting angle BORDER"=w874:i16)
                n438 = call <vilib>:"Write Key (String).vi"("section"=w825, "error in (no error)"=w890, "value"=w884, "key"="Track name", "refnum"=w892) -> ("error out"=w889:errorcluster, "refnum out"=w891:T3)  [unwired: 4 in, 1 out]
                n439 = call <vilib>:"Write Key (I32).vi"("section"=w825, "error in (no error)"=w889, "value"=w879, "key"="Amount of midfield segments", "refnum"=w891) -> ("error out"=w911:errorcluster, "refnum out"=w910:T3)  [unwired: 4 in, 1 out]
                n440 = call <vilib>:"Write Key (I32).vi"("section"=w825, "error in (no error)"=w911, "value"=w878, "key"="Amount of border segments", "refnum"=w910) -> ("error out"=w907:errorcluster, "refnum out"=w908:T3)  [unwired: 4 in, 1 out]
                n441 = call <vilib>:"Write Key (I32).vi"("section"=w825, "error in (no error)"=w907, "value"=w877, "key"="Center segment outer radius, mm", "refnum"=w908) -> ("error out"=w904:errorcluster, "refnum out"=w905:T3)  [unwired: 4 in, 1 out]
                n442 = call <vilib>:"Write Key (I32).vi"("section"=w825, "error in (no error)"=w904, "value"=w876, "key"="Midfield segments outer radius, mm", "refnum"=w905) -> ("error out"=w901:errorcluster, "refnum out"=w902:T3)  [unwired: 4 in, 1 out]
                n443 = call <vilib>:"Write Key (I32).vi"("section"=w825, "error in (no error)"=w901, "value"=w875, "key"="Midfield segments starting angle", "refnum"=w902) -> ("error out"=w899:errorcluster, "refnum out"=w898:T3)  [unwired: 4 in, 1 out]
                n444 = call <vilib>:"Write Key (I32).vi"("section"=w825, "error in (no error)"=w899, "value"=w874, "key"="Border segments starting angle", "refnum"=w898) -> ("error out"=w897:errorcluster, "refnum out"=w896:T3)  [unwired: 4 in, 1 out]
                n445 = local read "Current User"() -> (w851:string)
                n446 = call <vilib>:"Write Key (I32).vi"("section"=w825, "error in (no error)"=w897, "value"=w839, "key"="Cage diameter, mm", "refnum"=w896) -> ("error out"=w865:errorcluster, "refnum out"=w862:T3)  [unwired: 4 in, 1 out]
                n447 = property on="Vertical offset" class="DigNum (strict)"() -> ("Value"=w858:sgl)  [unwired: 2 in, 2 out]
                n448 = call <vilib>:"Open Config Data.vi"("configuration file path"=w860) -> ("error out"=w857:errorcluster, "refnum"=w855:T3)  [unwired: 8 in, 1 out]
                n449 = call <vilib>:"Write Key (Double).vi"("use system decimal point (T)"=FALSE, "section"=w825, "error in (no error)"=w865, "value"=w858, "key"=w859, "refnum"=w862) -> ("error out"=w864:errorcluster, "refnum out"=w863:T3)  [unwired: 3 in, 1 out]
                n450 = call <vilib>:"Write Key (Double).vi"("use system decimal point (T)"=FALSE, "section"=w851, "error in (no error)"=w857, "value"=w858, "key"=w859, "refnum"=w855) -> ("error out"=w854:errorcluster, "refnum out"=w850:T3)  [unwired: 3 in, 1 out]
                n451 = property on="Bridge swap" class="Bool (strict)"() -> ("Value"=w853:bool)  [unwired: 2 in, 2 out]
                n452 = call <vilib>:"Write Key (Boolean).vi"("section"=w851, "error in (no error)"=w854, "value"=w853, "key"=w852, "refnum"=w850) -> ("error out"=w849:errorcluster, "refnum out"=w848:T3)  [unwired: 4 in, 1 out]
                n453 = call <vilib>:"Write Key (Boolean).vi"("section"=w825, "error in (no error)"=w864, "value"=w853, "key"=w852, "refnum"=w863) -> ("error out"=w870:errorcluster, "refnum out"=w871:T3)  [unwired: 4 in, 1 out]
                n454 = call <vilib>:"Close Config Data.vi"("error in (no error)"=w849, "refnum"=w848) -> ()  [unwired: 8 in, 2 out]
                n455 = property on="Stimulus presets" class="Arr (strict)"(error in=w870) -> (error out=w828:errorcluster, "Value"=w872:T5)  [unwired: 1 in, 1 out]
                n456 = for {
                  tunnel: w872 -> [w944] mode=indexing
                  tunnel: w871 -> [w937]
                  tunnel: [w941] -> w829
                  tunnel: w825 -> [w932]
                  i -> [w940]
                  n457 = Unbundle By Name(w944) -> ("Stim. has been set"=w942:bool)
                  n458 = Flatten To JSON(anything=w944) -> (JSON string=w943:string, 11:w934:errorcluster)  [unwired: 2 in]
                  n459 = Format Value(string ("")="Zone " ("string"), format string="%02d", value (0)=w940) -> (output string=w935:string)
                  n460 = call <vilib>:"Remove Key.vi"("section"=w932, "error in (no error)"=w934, "key"=w935, "refnum"=w937) -> ("error out"=w933:errorcluster, "refnum out"=w936:T3)  [unwired: 5 in, 1 out]
                  n461 = case shown="True" w942 {
                    tunnel: w943 -> [_ w951]
                    tunnel: w933 -> [_ w950]
                    tunnel: [w945 w949] -> w941
                    tunnel: w935 -> [_ w948]
                    tunnel: w936 -> [w945 w947]
                    tunnel: w932 -> [_ w946]
                    frame False {
                    }
                    frame True {
                      n462 = call <vilib>:"Write Key (String).vi"("section"=w946, "error in (no error)"=w950, "value"=w951, "key"=w948, "refnum"=w947) -> ("refnum out"=w949:T3)  [unwired: 4 in, 2 out]
                    }
                  }
                }
                n463 = property on="IO parameters string" class="Str"(error in=w828) -> (error out=w830:errorcluster, "Value"=w831:string)  [unwired: 1 in, 1 out]
                n464 = call <vilib>:"Write Key (String).vi"("section"=w825, "error in (no error)"=w830, "value"=w831, "key"="IO ports configuration", "refnum"=w829) -> ("error out"=w827:errorcluster, "refnum out"=w826:T3)  [unwired: 4 in, 1 out]
                n465 = call <vilib>:"Close Config Data.vi"("error in (no error)"=w827, "refnum"=w826) -> ("error out"=w881:errorcluster)  [unwired: 8 in, 1 out]
              }
            }
            n466 = call-poly <vilib>:"Read Delimited Spreadsheet.vi"("file path (dialog if empty)"=w807, "error in (no error)"=w806) -> ("all rows"=w797:string[][], "error out"=w805:errorcluster)  [unwired: 8 in, 4 out]
            n467 = Array Subset(array=w797, index (row)=1 ("index")) -> (w796:string[][])  [unwired: 3 in]
            n468 = Select(t=w796, s=w799, f=w797) -> (s? t:f=w798:string[][])
            n469 = call-poly <vilib>:"Write Delimited Spreadsheet.vi"("file path (dialog if empty)"=w804, "format (%s)"="%s", "2D data"=w798, "append to file? (new file:F)"=TRUE, "error in (no error)"=w805) -> ("error out"=w816:errorcluster)  [unwired: 9 in, 1 out]
            "Path to the latest saved temp file" <- w819
            "Temp file ready" <- w818
          }
          frame #1 {
            n470 = Wait (ms)(milliseconds to wait=u32 257 ("millisecond multiple")) -> ()  [unwired: 1 out]
          }
          frame #2 {
            n471 = Unbundle By Name(w961) -> ("Recording now"=w957:refnum<notifier>, "Has been recorded"=w956:refnum<notifier>, "Path to the latest complete temp file"=w972:refnum<notifier>, "Temp file ready for processing"=w973:refnum<notifier>)
            n472 = Send Notification(notification=FALSE, notifier=w973, error in (no error)=w962) -> (error out=w971:errorcluster)  [unwired: 1 out]
            n473 = Get Notifier Status(notifier=w972, error in (no error)=w971) -> (current notification=w959:path, error out=w970:errorcluster)  [unwired: 3 out]
            n474 = Delete(path (use dialog)=w959, error in=w970) -> (error out=w965:errorcluster)  [unwired: 3 in, 2 out]
            n475 = Get Notifier Status(notifier=w956, error in (no error)=w965) -> (current notification=w967:bool, error out=w964:errorcluster)  [unwired: 3 out]
            n476 = Get Notifier Status(notifier=w957, error in (no error)=w964) -> (current notification=w969:bool, error out=w963:errorcluster)  [unwired: 3 out]
            n477 = Not(x=w969) -> (.not. x?=w968:bool)
            n478 = And(x=w968, y=w967) -> (x .and. y?=w966:bool)
          }
        }
        n479 = case "Here data saving will be finalized" shown="True" w773 {
          selector: w773 -> [w784 w794]
          tunnel: [w784 w794] -> w770
          tunnel: w771 -> [w783 w792]
          tunnel: [w783 w786] -> w769
          tunnel: w772 -> [_ w790]
          tunnel: w766 -> [_ w785]
          frame False {
          }
          frame True {
            n480 = Unbundle By Name(w785) -> ("Final csv output path"=w793:path, "Temporary csv output path"=w791:path)
            n481 = Unbundle By Name(w790) -> ("Final CSV saved"=w789:refnum<notifier>)
            n482 = Move(source path=w791, error in=w792, 10:w793) -> (error out=w787:errorcluster)  [unwired: 2 in, 2 out]
            n483 = Send Notification(notification=TRUE, notifier=w789, error in (no error)=w787) -> (error out=w786:errorcluster)  [unwired: 1 out]
          }
        }
      }
    }
  }
  "error out" <- w13
  n484 = Tick Count (ms)() -> (millisecond timer value=w15:u32)
  n485 = while {
    tunnel: w5 -> [w989]
    tunnel: w3 -> [w993]
    tunnel: w5 -> [w990]
    tunnel: w5 -> [w988]
    tunnel: w1 -> [w987]
    tunnel: w15 -> [w986]
    tunnel: w14 -> [w985]
    i -> [w991]
    stop <- w982 stop-if-true
    w992 = u32 37 ("milliseconds to wait")
    n486 = property on="Main tab control" class="TabCtl (strict)"(error in=w987) -> (error out=w994:errorcluster, "Value"=w995:enum32{"Settings", "Recording", "Analysis"})  [unwired: 1 in, 1 out]
    n487 = case shown="\"Analysis\"" w995 {
      tunnel: w994 -> [w1000 _ _]
      tunnel: w993 -> [_ w1503 _]
      tunnel: w992 -> [_ w1505 w1670]
      tunnel: w991 -> [_ _ _]
      tunnel: w990 -> [_ w1488 w1672]
      tunnel: w989 -> [w998 _ _]
      tunnel: w986 -> [_ w1500 _]
      tunnel: w985 -> [_ w1492 _]
      frame "Settings", Default {
        n488 = flat-sequence {
          tunnel: w1000 -> [w1002]
          tunnel: [w1002] -> w996
          tunnel: [w1024] -> w997
          tunnel: w996 -> [w1024]
          tunnel: [w1209] -> w999
          tunnel: w997 -> [w1209]
          tunnel: w999 -> [w1242]
          tunnel: w998 -> [w1241]
          frame #0 {
            n489 = case shown="True" "Set IO config" {
              frame False {
              }
              frame True {
                n490 = global read "SW_Globals.vi" "IO parameters cluster"() -> (w1016:T12)
                n491 = local read "Sync capability"() -> (w1017:u8)
                n492 = call "HW_set_IO_ports_3-pos.vi"("Sync capability"=w1017, "Sync parameters cluster input"=w1016) -> ("Sync parameters cluster output"=w1006:T12)
                n493 = call "SW_get_config_of_Zones_and_IO.vi"("Sync parameters cluster input"=w1006) -> ("Zones out config bin"=w1005:bool[], "Ports IO config (OUT is FALSE)"=w1004:bool[])  [unwired: 1 out]
                n494 = global write "SW_Globals.vi" "IO ports config"(w1004) -> ()
                n495 = global write "SW_Globals.vi" "Zones out config bin"(w1005) -> ()
                n496 = global write "SW_Globals.vi" "IO parameters cluster"(w1006) -> ()
                n497 = call "SW_get_config_for_Start_Stop_pulses.vi"("Sync parameters cluster input"=w1006) -> ("Start/Stop out pulses config"=w1010:u32, "Start/Stop in config"=w1009:u32, "Start/Stop in config bin"=w1008:bool[], "Start/Stop out pulses config bin"=w1007:bool[])
                n498 = global write "SW_Globals.vi" "Start/Stop out pulses config bin"(w1007) -> ()
                n499 = global write "SW_Globals.vi" "Start/Stop in config bin"(w1008) -> ()
                n500 = Cluster To Array(cluster=w1006) -> (array=w1003:u16[])
                n501 = call "SW_get_IO_ports_representation.vi"("Sync parameters cluster input"=w1006) -> ("IO status indicator"=w1019:T4)
                n502 = property on="Start/Stop out pulses config" class="DigNum (strict)"("Value"=w1010) -> ()  [unwired: 2 in, 2 out]
                n503 = Equal?(x=w1016, y=w1006) -> (x = y?=w1015:T31)
                n504 = property on="Start/Stop in config" class="DigNum (strict)"("Value"=w1009) -> ()  [unwired: 2 in, 2 out]
                n505 = Cluster To Array(cluster=w1015) -> (array=w1014:bool[])
                n506 = Not(x=w1014) -> (.not. x?=w1013:bool[])
                n507 = Boolean Array To Number(Boolean array=w1013) -> (number=w1012:u32)
                n508 = To Variant(anything=w1019) -> (Variant=w1018:variant)
                n509 = Flatten To JSON(anything=w1003) -> (JSON string=w1021:string, 11:w1020:errorcluster)  [unwired: 2 in]
                n510 = Equal To 0?(x=w1012) -> (x = 0?=w1011:bool)
                n511 = property on="IO status indicator" class="Clust"("Value"=w1018) -> ()  [unwired: 2 in, 2 out]
                n512 = property on="IO parameters string" class="Str"(error in=w1020, "Value"=w1021) -> ()  [unwired: 1 in, 2 out]
                n513 = case shown="False" w1011 {
                  frame False {
                    n514 = property on="Changed IO" class="Bool (strict)"("Val(Sgnl)"=TRUE ("Value (Signaling)")) -> ()  [unwired: 2 in, 2 out]
                  }
                  frame True {
                  }
                }
              }
            }
          }
          frame #1 {
            n515 = event shown="[5] \"Reset stimuli\", \"Changed IO\": Value Change" {
              selector: _ -> [_ _ _ _ _ _ _]
              dyn-events: _ -> [_ _ _ _ _ _ _]
              timeout: 1 -> [_ _ _ _ _ _ _]
              event Timeout {
                n516 = event-data() -> ()  [unwired: 1 in, 3 out]
              }
              event "Segments diagram": Mouse Down {
                n517 = event-data() -> ("Coords"=→"Coords":T2, "Button"=→"Button":u16)  [unwired: 1 in, 6 out]
              }
              event "N segments BORDER", "N segments MIDFIELD": Value Change {
                n518 = event-data() -> ()  [unwired: 1 in, 6 out]
                n519 = property on="N segments BORDER" class="DigNum (strict)"() -> (error out=w1029:errorcluster, "Value"=w1032:u8)  [unwired: 2 in, 1 out]
                n520 = property on="N segments MIDFIELD" class="DigNum (strict)"(error in=w1029) -> (error out=w1028:errorcluster, "Value"=w1031:u8)  [unwired: 1 in, 1 out]
                n521 = property on="Stim. setup" class="RadioBtnsControl (strict)"(error in=w1028) -> ("Controls[]"=w1030:refnum<vi>[])  [unwired: 1 in, 2 out]
                n522 = Compound Arithmetic op=ADD(w1032, w1031, u8 1 ("value")) -> (w1027:u8)
                n523 = for {
                  tunnel: w1030 -> [w1041] mode=indexing
                  tunnel: w1027 -> [w1037]
                  i -> [w1036]
                  n524 = Increment(x=w1036) -> (x+1=w1035:i32)
                  n525 = Greater Or Equal?(x=w1037, y=w1035) -> (x >= y?=w1034:bool)
                  n526 = Select(t=T9."Enabled" ("Disabled"), s=w1034, f=T9."Disabled and Grayed Out") -> (s? t:f=w1039:T9)
                  n527 = property class="Ctl"(reference=w1041, "DisabledEnum"=w1039) -> ()  [unwired: 1 in, 2 out]
                }
              }
              event "Stim. setup": Value Change {
                n528 = event-data() -> ("NewVal"=w1043:T6)  [unwired: 1 in, 5 out]
                n529 = To Unsigned Byte Integer(number=w1043) -> (unsigned 8bit integer=w1042:u8)
                n530 = case shown="1.." w1042 {
                  selector: w1042 -> [w1044 w1047]
                  frame 0, Default {
                    n531 = Build Array(w1044) -> (w1046:u8[])
                    n532 = property on="Stimulus presets" class="Arr (strict)"("Index Values"=w1046, "DisabledEnum"=T9."Disabled and Grayed Out" ("Disabled")) -> ()  [unwired: 2 in, 2 out]
                  }
                  frame 1.. {
                    n533 = Build Array(w1047) -> (w1049:u8[])
                    n534 = property on="Stimulus presets" class="Arr (strict)"("Index Values"=w1049, "DisabledEnum"=T9."Enabled" ("Disabled")) -> ()  [unwired: 2 in, 2 out]
                  }
                }
              }
              event "Stimulus presets": Value Change {
                n535 = event-data() -> ("NewVal"=w1065:T5)  [unwired: 1 in, 5 out]
                n536 = property on="Stimulus presets" class="Arr (strict)"() -> ("Index Values"=w1067:u32[])  [unwired: 2 in, 2 out]
                n537 = Index Array(array=w1067, index=0) -> (element=w1050:u32)
                n538 = Index Array(array=w1065, index=w1050) -> (element=w1059:T32)
                n539 = Unbundle By Name(w1059) -> ("Set/Clear"=w1060:bool, "Time, s"=w1054:sgl, "Stimulus, s"=w1052:sgl)
                n540 = property on="Stim. setup" class="RadioBtnsControl (strict)"() -> ("Value"=w1064:T6)  [unwired: 2 in, 2 out]
                n541 = Format Into String(w1064) -> ()  [unwired: 3 in, 2 out]
                n542 = Greater Than 0?(x=w1054) -> (x > 0?=w1062:bool)
                n543 = Greater Than 0?(x=w1052) -> (x > 0?=w1061:bool)
                n544 = expression code="floor(x * 100) / 100"(w1054) -> (w1053:sgl)
                n545 = expression code="floor(x * 100) / 100"(w1052) -> (w1051:sgl)
                n546 = To Unsigned Byte Integer(number=w1064) -> (unsigned 8bit integer=w1063:u8)
                n547 = Compound Arithmetic op=AND(w1060, w1062, w1061) -> (w1057:bool)
                n548 = case shown="1" w1063 {
                  tunnel: w1057 -> [_ w1073 w1077 w1081 w1085 w1089 w1093 w1097 w1101 w1105 w1109 w1113 w1117 w1121]
                  frame 0, Default {
                  }
                  frame 1 {
                    n549 = property on="Colors for Stim. setup" class="Arr (strict)"() -> ("Value"=w1072:T1)  [unwired: 2 in, 2 out]
                    n550 = Select(t=w1072, s=w1073, f=T8 [{"Numeric Control"=12369084, "Numeric Control"=12369084}, {"Numeric Control"=6603023, "Numeric Control"=6603023}, {"Numeric Control"=1976113, "Numeric Control"=1976113}, {"Numeric Control"=2575993, "Numeric Control"=2575993}] ("Colors [4] 2")) -> (s? t:f=w1075:T8)
                    n551 = property on="Zone 01" class="Bool (strict)"("Colors [4]"=w1075) -> ()  [unwired: 2 in, 2 out]
                  }
                  frame 2 {
                    n552 = property on="Colors for Stim. setup" class="Arr (strict)"() -> ("Value"=w1076:T1)  [unwired: 2 in, 2 out]
                    n553 = Select(t=w1076, s=w1077, f=T8 [{"Numeric Control"=12369084, "Numeric Control"=12369084}, {"Numeric Control"=6603023, "Numeric Control"=6603023}, {"Numeric Control"=1976113, "Numeric Control"=1976113}, {"Numeric Control"=2575993, "Numeric Control"=2575993}] ("Colors [4] 2")) -> (s? t:f=w1079:T8)
                    n554 = property on="Zone 02" class="Bool (strict)"("Colors [4]"=w1079) -> ()  [unwired: 2 in, 2 out]
                  }
                  frame 3 {
                    n555 = property on="Colors for Stim. setup" class="Arr (strict)"() -> ("Value"=w1080:T1)  [unwired: 2 in, 2 out]
                    n556 = Select(t=w1080, s=w1081, f=T8 [{"Numeric Control"=12369084, "Numeric Control"=12369084}, {"Numeric Control"=6603023, "Numeric Control"=6603023}, {"Numeric Control"=1976113, "Numeric Control"=1976113}, {"Numeric Control"=2575993, "Numeric Control"=2575993}] ("Colors [4] 2")) -> (s? t:f=w1083:T8)
                    n557 = property on="Zone 03" class="Bool (strict)"("Colors [4]"=w1083) -> ()  [unwired: 2 in, 2 out]
                  }
                  frame 4 {
                    n558 = property on="Colors for Stim. setup" class="Arr (strict)"() -> ("Value"=w1084:T1)  [unwired: 2 in, 2 out]
                    n559 = Select(t=w1084, s=w1085, f=T8 [{"Numeric Control"=12369084, "Numeric Control"=12369084}, {"Numeric Control"=6603023, "Numeric Control"=6603023}, {"Numeric Control"=1976113, "Numeric Control"=1976113}, {"Numeric Control"=2575993, "Numeric Control"=2575993}] ("Colors [4] 2")) -> (s? t:f=w1087:T8)
                    n560 = property on="Zone 04" class="Bool (strict)"("Colors [4]"=w1087) -> ()  [unwired: 2 in, 2 out]
                  }
                  frame 5 {
                    n561 = property on="Colors for Stim. setup" class="Arr (strict)"() -> ("Value"=w1088:T1)  [unwired: 2 in, 2 out]
                    n562 = Select(t=w1088, s=w1089, f=T8 [{"Numeric Control"=12369084, "Numeric Control"=12369084}, {"Numeric Control"=6603023, "Numeric Control"=6603023}, {"Numeric Control"=1976113, "Numeric Control"=1976113}, {"Numeric Control"=2575993, "Numeric Control"=2575993}] ("Colors [4] 2")) -> (s? t:f=w1091:T8)
                    n563 = property on="Zone 05" class="Bool (strict)"("Colors [4]"=w1091) -> ()  [unwired: 2 in, 2 out]
                  }
                  frame 6 {
                    n564 = property on="Colors for Stim. setup" class="Arr (strict)"() -> ("Value"=w1092:T1)  [unwired: 2 in, 2 out]
                    n565 = Select(t=w1092, s=w1093, f=T8 [{"Numeric Control"=12369084, "Numeric Control"=12369084}, {"Numeric Control"=6603023, "Numeric Control"=6603023}, {"Numeric Control"=1976113, "Numeric Control"=1976113}, {"Numeric Control"=2575993, "Numeric Control"=2575993}] ("Colors [4] 2")) -> (s? t:f=w1095:T8)
                    n566 = property on="Zone 06" class="Bool (strict)"("Colors [4]"=w1095) -> ()  [unwired: 2 in, 2 out]
                  }
                  frame 7 {
                    n567 = property on="Colors for Stim. setup" class="Arr (strict)"() -> ("Value"=w1096:T1)  [unwired: 2 in, 2 out]
                    n568 = Select(t=w1096, s=w1097, f=T8 [{"Numeric Control"=12369084, "Numeric Control"=12369084}, {"Numeric Control"=6603023, "Numeric Control"=6603023}, {"Numeric Control"=1976113, "Numeric Control"=1976113}, {"Numeric Control"=2575993, "Numeric Control"=2575993}] ("Colors [4] 2")) -> (s? t:f=w1099:T8)
                    n569 = property on="Zone 07" class="Bool (strict)"("Colors [4]"=w1099) -> ()  [unwired: 2 in, 2 out]
                  }
                  frame 8 {
                    n570 = property on="Colors for Stim. setup" class="Arr (strict)"() -> ("Value"=w1100:T1)  [unwired: 2 in, 2 out]
                    n571 = Select(t=w1100, s=w1101, f=T8 [{"Numeric Control"=12369084, "Numeric Control"=12369084}, {"Numeric Control"=6603023, "Numeric Control"=6603023}, {"Numeric Control"=1976113, "Numeric Control"=1976113}, {"Numeric Control"=2575993, "Numeric Control"=2575993}] ("Colors [4] 2")) -> (s? t:f=w1103:T8)
                    n572 = property on="Zone 08" class="Bool (strict)"("Colors [4]"=w1103) -> ()  [unwired: 2 in, 2 out]
                  }
                  frame 9 {
                    n573 = property on="Colors for Stim. setup" class="Arr (strict)"() -> ("Value"=w1104:T1)  [unwired: 2 in, 2 out]
                    n574 = Select(t=w1104, s=w1105, f=T8 [{"Numeric Control"=12369084, "Numeric Control"=12369084}, {"Numeric Control"=6603023, "Numeric Control"=6603023}, {"Numeric Control"=1976113, "Numeric Control"=1976113}, {"Numeric Control"=2575993, "Numeric Control"=2575993}] ("Colors [4] 2")) -> (s? t:f=w1107:T8)
                    n575 = property on="Zone 09" class="Bool (strict)"("Colors [4]"=w1107) -> ()  [unwired: 2 in, 2 out]
                  }
                  frame 10 {
                    n576 = property on="Colors for Stim. setup" class="Arr (strict)"() -> ("Value"=w1108:T1)  [unwired: 2 in, 2 out]
                    n577 = Select(t=w1108, s=w1109, f=T8 [{"Numeric Control"=12369084, "Numeric Control"=12369084}, {"Numeric Control"=6603023, "Numeric Control"=6603023}, {"Numeric Control"=1976113, "Numeric Control"=1976113}, {"Numeric Control"=2575993, "Numeric Control"=2575993}] ("Colors [4] 2")) -> (s? t:f=w1111:T8)
                    n578 = property on="Zone 10" class="Bool (strict)"("Colors [4]"=w1111) -> ()  [unwired: 2 in, 2 out]
                  }
                  frame 11 {
                    n579 = property on="Colors for Stim. setup" class="Arr (strict)"() -> ("Value"=w1112:T1)  [unwired: 2 in, 2 out]
                    n580 = Select(t=w1112, s=w1113, f=T8 [{"Numeric Control"=12369084, "Numeric Control"=12369084}, {"Numeric Control"=6603023, "Numeric Control"=6603023}, {"Numeric Control"=1976113, "Numeric Control"=1976113}, {"Numeric Control"=2575993, "Numeric Control"=2575993}] ("Colors [4] 2")) -> (s? t:f=w1115:T8)
                    n581 = property on="Zone 11" class="Bool (strict)"("Colors [4]"=w1115) -> ()  [unwired: 2 in, 2 out]
                  }
                  frame 12 {
                    n582 = property on="Colors for Stim. setup" class="Arr (strict)"() -> ("Value"=w1116:T1)  [unwired: 2 in, 2 out]
                    n583 = Select(t=w1116, s=w1117, f=T8 [{"Numeric Control"=12369084, "Numeric Control"=12369084}, {"Numeric Control"=6603023, "Numeric Control"=6603023}, {"Numeric Control"=1976113, "Numeric Control"=1976113}, {"Numeric Control"=2575993, "Numeric Control"=2575993}] ("Colors [4] 2")) -> (s? t:f=w1119:T8)
                    n584 = property on="Zone 12" class="Bool (strict)"("Colors [4]"=w1119) -> ()  [unwired: 2 in, 2 out]
                  }
                  frame 13 {
                    n585 = property on="Colors for Stim. setup" class="Arr (strict)"() -> ("Value"=w1120:T1)  [unwired: 2 in, 2 out]
                    n586 = Select(t=w1120, s=w1121, f=T8 [{"Numeric Control"=12369084, "Numeric Control"=12369084}, {"Numeric Control"=6603023, "Numeric Control"=6603023}, {"Numeric Control"=1976113, "Numeric Control"=1976113}, {"Numeric Control"=2575993, "Numeric Control"=2575993}] ("Colors [4] 2")) -> (s? t:f=w1123:T8)
                    n587 = property on="Zone 13" class="Bool (strict)"("Colors [4]"=w1123) -> ()  [unwired: 2 in, 2 out]
                  }
                }
                n588 = Bundle By Name(cluster=w1059, "Stim. has been set"=w1057, "Set/Clear"=w1057, "Time, s"=w1053, "Stimulus, s"=w1051) -> (w1058:T32)
                n589 = Replace Array Subset(array=w1065, new element=w1058, index=w1050) -> (w1055:T5)
                n590 = global write "SW_Globals.vi" "Stimulus presets"(w1055) -> ()
                n591 = property on="Stimulus presets" class="Arr (strict)"("Value"=w1055) -> ()  [unwired: 2 in, 2 out]
                n592 = for {
                  tunnel: w1055 -> [w1071] mode=indexing
                  tunnel: [w1068] -> w1056 mode=indexing if=w1069
                  i -> [w1070]
                  n593 = Unbundle By Name(w1071) -> ("Stim. has been set"=w1069:bool)
                  n594 = To Unsigned Byte Integer(number=w1070) -> (unsigned 8bit integer=w1068:u8)
                }
                n595 = global write "SW_Globals.vi" "Regions to track"(w1056) -> ()
              }
              event "Reset stimuli", "Changed IO": Value Change {
                n596 = event-data() -> ("OldVal"=w1125:bool, "NewVal"=w1126:bool)  [unwired: 1 in, 4 out]
                n597 = property on="Reset stimuli" class="Bool (strict)"("Value"=w1125) -> ()  [unwired: 2 in, 2 out]
                n598 = property on="Changed IO" class="Bool (strict)"("Value"=FALSE ("Changed IO")) -> ()  [unwired: 2 in, 2 out]
                n599 = case shown="True" w1126 {
                  selector: w1126 -> [_ w1145]
                  frame False {
                  }
                  frame True {
                    w1132 = T8 [{"Numeric Control"=9868950, "Numeric Control"=15790320}, {"Numeric Control"=8388608, "Numeric Control"=8388608}, {"Numeric Control"=4934475, "Numeric Control"=7895160}, {"Numeric Control"=994319, "Numeric Control"=1657881}]  # TTL IO In colors
                    w1133 = T8 [{"Numeric Control"=9868950, "Numeric Control"=15790320}, {"Numeric Control"=1988894, "Numeric Control"=3381555}, {"Numeric Control"=4934475, "Numeric Control"=7895160}, {"Numeric Control"=994319, "Numeric Control"=1657881}]  # TTL IO Out colors
                    (unwired) T33 [{"String"="1", "Value"=1}, {"String"="2", "Value"=2}, {"String"="1+2", "Value"=3}, {"String"="5+6", "Value"=4}] ("Strings And Values")
                    n600 = global read "SW_Globals.vi" "IO parameters cluster"() -> (w1144:T12)
                    n601 = Unbundle By Name(w1144) -> ("SYNC configuration"=w1143:u16)
                    n602 = global write "SW_Globals.vi" "Regions to track"(u8[] []) -> ()
                    n603 = for {
                      N: 14 -> [_]
                      tunnel: [T30 {"Event type"=0, "Cond., s"=0.0, "Stim., s"=0.0, "Set/Clear"=FALSE, "TTL out N"=1, "Stim. has been set"=FALSE} ("Cluster of the stimuls settings")] -> w1150 mode=indexing
                      tunnel: [w1151] -> w1146
                      tunnel: w1145 -> [w1151]
                      i -> [w1152]
                      n604 = case shown="5" w1152 {
                        frame 0, Default {
                        }
                        frame 1 {
                          n605 = property on="Zone 01" class="Bool (strict)"("Colors [4]"=T8 [{"Numeric Control"=12369084, "Numeric Control"=12369084}, {"Numeric Control"=6603023, "Numeric Control"=6603023}, {"Numeric Control"=1976113, "Numeric Control"=1976113}, {"Numeric Control"=2575993, "Numeric Control"=2575993}] ("Colors [4] 2"), "Value"=FALSE) -> ()  [unwired: 2 in, 2 out]
                        }
                        frame 2 {
                          n606 = property on="Zone 02" class="Bool (strict)"("Colors [4]"=T8 [{"Numeric Control"=12369084, "Numeric Control"=12369084}, {"Numeric Control"=6603023, "Numeric Control"=6603023}, {"Numeric Control"=1976113, "Numeric Control"=1976113}, {"Numeric Control"=2575993, "Numeric Control"=2575993}] ("Colors [4] 2"), "Value"=FALSE) -> ()  [unwired: 2 in, 2 out]
                        }
                        frame 3 {
                          n607 = property on="Zone 03" class="Bool (strict)"("Colors [4]"=T8 [{"Numeric Control"=12369084, "Numeric Control"=12369084}, {"Numeric Control"=6603023, "Numeric Control"=6603023}, {"Numeric Control"=1976113, "Numeric Control"=1976113}, {"Numeric Control"=2575993, "Numeric Control"=2575993}] ("Colors [4] 2"), "Value"=FALSE) -> ()  [unwired: 2 in, 2 out]
                        }
                        frame 4 {
                          n608 = property on="Zone 04" class="Bool (strict)"("Colors [4]"=T8 [{"Numeric Control"=12369084, "Numeric Control"=12369084}, {"Numeric Control"=6603023, "Numeric Control"=6603023}, {"Numeric Control"=1976113, "Numeric Control"=1976113}, {"Numeric Control"=2575993, "Numeric Control"=2575993}] ("Colors [4] 2"), "Value"=FALSE) -> ()  [unwired: 2 in, 2 out]
                        }
                        frame 5 {
                          n609 = property on="Zone 05" class="Bool (strict)"("Colors [4]"=T8 [{"Numeric Control"=12369084, "Numeric Control"=12369084}, {"Numeric Control"=6603023, "Numeric Control"=6603023}, {"Numeric Control"=1976113, "Numeric Control"=1976113}, {"Numeric Control"=2575993, "Numeric Control"=2575993}] ("Colors [4] 2"), "Value"=FALSE) -> ()  [unwired: 2 in, 2 out]
                        }
                        frame 6 {
                          n610 = property on="Zone 06" class="Bool (strict)"("Colors [4]"=T8 [{"Numeric Control"=12369084, "Numeric Control"=12369084}, {"Numeric Control"=6603023, "Numeric Control"=6603023}, {"Numeric Control"=1976113, "Numeric Control"=1976113}, {"Numeric Control"=2575993, "Numeric Control"=2575993}] ("Colors [4] 2"), "Value"=FALSE) -> ()  [unwired: 2 in, 2 out]
                        }
                        frame 7 {
                          n611 = property on="Zone 07" class="Bool (strict)"("Colors [4]"=T8 [{"Numeric Control"=12369084, "Numeric Control"=12369084}, {"Numeric Control"=6603023, "Numeric Control"=6603023}, {"Numeric Control"=1976113, "Numeric Control"=1976113}, {"Numeric Control"=2575993, "Numeric Control"=2575993}] ("Colors [4] 2"), "Value"=FALSE) -> ()  [unwired: 2 in, 2 out]
                        }
                        frame 8 {
                          n612 = property on="Zone 08" class="Bool (strict)"("Colors [4]"=T8 [{"Numeric Control"=12369084, "Numeric Control"=12369084}, {"Numeric Control"=6603023, "Numeric Control"=6603023}, {"Numeric Control"=1976113, "Numeric Control"=1976113}, {"Numeric Control"=2575993, "Numeric Control"=2575993}] ("Colors [4] 2"), "Value"=FALSE) -> ()  [unwired: 2 in, 2 out]
                        }
                        frame 9 {
                          n613 = property on="Zone 09" class="Bool (strict)"("Colors [4]"=T8 [{"Numeric Control"=12369084, "Numeric Control"=12369084}, {"Numeric Control"=6603023, "Numeric Control"=6603023}, {"Numeric Control"=1976113, "Numeric Control"=1976113}, {"Numeric Control"=2575993, "Numeric Control"=2575993}] ("Colors [4] 2"), "Value"=FALSE) -> ()  [unwired: 2 in, 2 out]
                        }
                        frame 10 {
                          n614 = property on="Zone 10" class="Bool (strict)"("Colors [4]"=T8 [{"Numeric Control"=12369084, "Numeric Control"=12369084}, {"Numeric Control"=6603023, "Numeric Control"=6603023}, {"Numeric Control"=1976113, "Numeric Control"=1976113}, {"Numeric Control"=2575993, "Numeric Control"=2575993}] ("Colors [4] 2"), "Value"=FALSE) -> ()  [unwired: 2 in, 2 out]
                        }
                        frame 11 {
                          n615 = property on="Zone 11" class="Bool (strict)"("Colors [4]"=T8 [{"Numeric Control"=12369084, "Numeric Control"=12369084}, {"Numeric Control"=6603023, "Numeric Control"=6603023}, {"Numeric Control"=1976113, "Numeric Control"=1976113}, {"Numeric Control"=2575993, "Numeric Control"=2575993}] ("Colors [4] 2"), "Value"=FALSE) -> ()  [unwired: 2 in, 2 out]
                        }
                        frame 12 {
                          n616 = property on="Zone 12" class="Bool (strict)"("Colors [4]"=T8 [{"Numeric Control"=12369084, "Numeric Control"=12369084}, {"Numeric Control"=6603023, "Numeric Control"=6603023}, {"Numeric Control"=1976113, "Numeric Control"=1976113}, {"Numeric Control"=2575993, "Numeric Control"=2575993}] ("Colors [4] 2"), "Value"=FALSE) -> ()  [unwired: 2 in, 2 out]
                        }
                        frame 13 {
                          n617 = property on="Zone 13" class="Bool (strict)"("Colors [4]"=T8 [{"Numeric Control"=12369084, "Numeric Control"=12369084}, {"Numeric Control"=6603023, "Numeric Control"=6603023}, {"Numeric Control"=1976113, "Numeric Control"=1976113}, {"Numeric Control"=2575993, "Numeric Control"=2575993}] ("Colors [4] 2"), "Value"=FALSE) -> ()  [unwired: 2 in, 2 out]
                        }
                      }
                    }
                    n618 = call "SW_Gen_Available_TTL_outputs_array.vi"("SYNC configuration"=w1143) -> ("Available TTL outputs array"=w1142:cluster{"String":string, "Value":i32}[])
                    n619 = property on="TTL out" class="Ring (strict)"("StringsAndValues[]"=w1142) -> ()  [unwired: 2 in, 2 out]
                    n620 = global read "SW_Globals.vi" "IO ports config"() -> (w1131:bool[])
                    n621 = Index Array(array=w1131, index=0) -> (element=w1137:bool)
                    n622 = Index Array(array=w1131, index=1) -> (element=w1136:bool)
                    n623 = Index Array(array=w1131, index=2) -> (element=w1135:bool)
                    n624 = Index Array(array=w1131, index=3) -> (element=w1134:bool)
                    n625 = Select(t=w1132, s=w1137, f=w1133) -> (s? t:f=w1130:T8)
                    n626 = Select(t=w1132, s=w1136, f=w1133) -> (s? t:f=w1129:T8)
                    n627 = Select(t=w1132, s=w1134, f=w1133) -> (s? t:f=w1127:T8)
                    n628 = Select(t=w1132, s=w1135, f=w1133) -> (s? t:f=w1128:T8)
                    n629 = property on="TTL IO 1 (recording)" class="Bool (strict)"("Colors [4]"=w1130) -> ()  [unwired: 2 in, 2 out]
                    n630 = property on="TTL IO 3 (recording)" class="Bool (strict)"("Colors [4]"=w1128) -> ()  [unwired: 2 in, 2 out]
                    n631 = property on="TTL IO 2 (recording)" class="Bool (strict)"("Colors [4]"=w1129) -> ()  [unwired: 2 in, 2 out]
                    n632 = property on="TTL IO 4 (recording)" class="Bool (strict)"("Colors [4]"=w1127) -> ()  [unwired: 2 in, 2 out]
                    n633 = property on="TTL IO 1 (analysis)" class="Bool"("Colors [4]"=w1130) -> ()  [unwired: 2 in, 2 out]
                    n634 = property on="TTL IO 3 (analysis)" class="Bool"("Colors [4]"=w1128) -> ()  [unwired: 2 in, 2 out]
                    n635 = property on="TTL IO 2 (analysis)" class="Bool"("Colors [4]"=w1129) -> ()  [unwired: 2 in, 2 out]
                    n636 = property on="TTL IO 4 (analysis)" class="Bool"("Colors [4]"=w1127) -> ()  [unwired: 2 in, 2 out]
                    n637 = global write "SW_Globals.vi" "Stimulus presets"(w1150) -> ()
                    n638 = property on="Stimulus presets" class="Arr (strict)"("Value"=w1150) -> (error out=w1147:errorcluster)  [unwired: 2 in, 1 out]
                    n639 = property on="Reset STIM" class="Bool (strict)"(error in=w1147, "Val(Sgnl)"=w1146) -> ()  [unwired: 1 in, 2 out]
                  }
                }
              }
              event "Reset regions": Value Change {
                n640 = event-data() -> ("OldVal"=w1180:bool, "NewVal"=w1181:bool)  [unwired: 1 in, 4 out]
                n641 = property on="Reset regions" class="Bool (strict)"("Value"=w1180) -> ()  [unwired: 2 in, 2 out]
                n642 = case shown="True" w1181 {
                  selector: w1181 -> [_ w1183]
                  frame False {
                  }
                  frame True {
                    n643 = local read "Cage diameter, mm"() -> (w1184:u16)
                    n644 = case shown="333" w1184 {
                      tunnel: w1183 -> [w1185 w1192 w1199]
                      tunnel: [w1185 w1192 w1199] -> w1182
                      frame 180, Default {
                        n645 = local write "Starting angle BORDER"(i16 0 ("Starting angle")) -> ()
                        n646 = local write "Starting angle MIDFIELD"(i16 0 ("Starting angle")) -> ()
                        n647 = local write "N segments MIDFIELD"(u8 2 ("N segments")) -> ()
                        n648 = local write "N segments BORDER"(u8 4 ("N segments")) -> ()
                        n649 = local write "Radius, mm CENTER"(u16 30 ("Radius, mm")) -> ()
                        n650 = local write "Radius, mm MIDFIELD"(u16 75 ("Radius, mm")) -> ()
                      }
                      frame 325 {
                        n651 = local write "Starting angle BORDER"(i16 0 ("Starting angle")) -> ()
                        n652 = local write "Starting angle MIDFIELD"(i16 0 ("Starting angle")) -> ()
                        n653 = local write "N segments MIDFIELD"(u8 2 ("N segments")) -> ()
                        n654 = local write "N segments BORDER"(u8 4 ("N segments")) -> ()
                        n655 = local write "Radius, mm CENTER"(u16 50 ("Radius, mm")) -> ()
                        n656 = local write "Radius, mm MIDFIELD"(u16 148 ("Radius, mm")) -> ()
                      }
                      frame 333 {
                        n657 = local write "Starting angle BORDER"(i16 0 ("Starting angle")) -> ()
                        n658 = local write "Starting angle MIDFIELD"(i16 0 ("Starting angle")) -> ()
                        n659 = local write "N segments MIDFIELD"(u8 2 ("N segments")) -> ()
                        n660 = local write "N segments BORDER"(u8 4 ("N segments")) -> ()
                        n661 = local write "Radius, mm CENTER"(u16 50 ("Radius, mm")) -> ()
                        n662 = local write "Radius, mm MIDFIELD"(u16 152 ("Radius, mm")) -> ()
                      }
                    }
                    n663 = property on="Reset REG" class="Bool (strict)"("Val(Sgnl)"=w1182) -> ()  [unwired: 2 in, 2 out]
                  }
                }
              }
            }
          }
          frame #2 {
            # "Segments scheme can be reset here"
            n664 = First Call?() -> (First Call?: T/F=w1207:bool)
            n665 = case shown="True" w1207 {
              selector: w1207 -> [_ w1211]
              tunnel: [_ w1210] -> w1208
              frame False {
              }
              frame True {
                n666 = property on="Init plot" class="Bool (strict)"("Val(Sgnl)"=w1211) -> (error out=w1210:errorcluster)  [unwired: 2 in, 1 out]
              }
            }
            n667 = event shown="[0] \"Init plot\", \"Stim. setup\", \"N segments MIDFIELD\", \"N segments BORDER\", \"Starting angle MIDFIELD\", \"Starting angle BORDER\", \"Radius, mm MIDFIELD\", \"Radius, mm CENTER\", \"Cage diameter, mm\", \"Reset stimuli\", \"Reset regions\", \"Reset REG\", \"Reset STIM\": Value Change" {
              selector: _ -> [_ _]
              dyn-events: _ -> [_ _]
              timeout: 1 -> [_ _]
              tunnel: w1208 -> [_ _]
              event "Init plot", "Stim. setup", "N segments MIDFIELD", "N segments BORDER", "Starting angle MIDFIELD", "Starting angle BORDER", "Radius, mm MIDFIELD", "Radius, mm CENTER", "Cage diameter, mm", "Reset stimuli", "Reset regions", "Reset REG", "Reset STIM": Value Change {
                n668 = event-data() -> ()  [unwired: 1 in, 6 out]
                n669 = local read "Cage diameter, mm"() -> (w1220:u16)
                n670 = global read "SW_Globals.vi" "Regions to track"() -> (w1234:u8[])
                n671 = To Unsigned Byte Integer(number="Stim. setup") -> (unsigned 8bit integer=w1235:u8)
                n672 = property on="Segments diagram" class="Pict"() -> ("Bounds"=w1232:T14)  [unwired: 2 in, 2 out]
                n673 = Bundle("N segments BORDER"="N segments BORDER", "Starting angle BORDER"="Starting angle BORDER", "N segments MIDFIELD"="N segments MIDFIELD", "Starting angle MIDFIELD"="Starting angle MIDFIELD", "Radius, mm MIDFIELD"="Radius, mm MIDFIELD", u8 1, "Radius, mm CENTER"="Radius, mm CENTER", "Cage diameter, mm"=w1220, 10) -> (w1219:T34)  [unwired: 1 in]
                n674 = Build Array(w1235) -> (w1229:u8[])
                n675 = Build Array (concatenate)(w1229, w1234) -> (w1233:u8[])
                n676 = call "SW_Gen_Check_segments_parameters.vi"("Image plotting parameters"=w1219) -> ("Corrected image plotting parameters"=w1218:T35)  [unwired: 2 in]
                n677 = Unbundle By Name(w1218) -> ("N segments BORDER"=w1217:u8, "N segments MIDFIELD"=w1215:u8, "Radius, mm MIDFIELD"=w1214:u16, "Radius, mm CENTER"=w1216:u16)
                n678 = call "SW_Generate_Segmented_Plot_v3.vi"("Draw Area Size"=w1232, "Regions to mark set"=w1233, "Regions to mark selected"=w1229, "Input cluster of parameters"=w1218) -> ("Zones layout output"=w1231:picture, "No zones image"=w1230:picture, "Array of the pixel to color correspondences"=w1212:u32[][], "Array of the segment to color correspondences"=w1213:u32[][])  [unwired: 6 in, 2 out]
                "Segments diagram" <- w1231
                n679 = global write "SW_Globals.vi" "Diagram"(w1231) -> ()
                n680 = global write "SW_Globals.vi" "Diagram no zones"(w1230) -> ()
                n681 = global write "SW_Globals.vi" "Array of the pixel to color correspondences"(w1212) -> ()
                n682 = global write "SW_Globals.vi" "Array of the segment to color correspondences"(w1213) -> ()
                n683 = property on="N segments BORDER" class="DigNum (strict)"("Value"=w1217) -> ()  [unwired: 2 in, 2 out]
                n684 = property on="N segments MIDFIELD" class="DigNum (strict)"("Value"=w1215) -> ()  [unwired: 2 in, 2 out]
                n685 = property on="Radius, mm MIDFIELD" class="DigNum (strict)"("Value"=w1214) -> ()  [unwired: 2 in, 2 out]
                n686 = property on="Radius, mm CENTER" class="DigNum (strict)"("Value"=w1216) -> ()  [unwired: 2 in, 2 out]
              }
              event Timeout {
                n687 = event-data() -> ()  [unwired: 1 in, 3 out]
              }
            }
          }
          frame #3 {
            # "Save settings and set important variables befor actual start of the recording. Also initial \"Play\" command is sent from here."
            n688 = Build Array("Start Tracking button", "Jump to Analysis") -> (w1239:bool[])
            n689 = Boolean Array To Number(Boolean array=w1239) -> (number=w1237:u32)
            n690 = case shown="1" w1237 {
              tunnel: w1242 -> [_ w1300 w1405]
              tunnel: w1241 -> [_ w1299 _]
              frame 0, Default {
              }
              frame 1 {
                w1334 = enum32{"Settings", "Recording", "Analysis"}."Recording" ("Main tab control")
                w1338 = enum32{"Settings", "Recording", "Analysis"}."Analysis" ("Main tab control")
                w1347 = enum32{"Settings", "Recording", "Analysis"}."Settings" ("Main tab control")
                n691 = flat-sequence {
                  tunnel: w1300 -> [w1383]
                  tunnel: w1299 -> [w1377]
                  tunnel: [w1383] -> w1298
                  tunnel: w1298 -> [w1385]
                  tunnel: [w1385] -> w1245
                  tunnel: [w1386] -> w1275
                  tunnel: w1245 -> [w1386]
                  frame #0 {
                    n692 = Unbundle By Name(w1377) -> ("Play/Pause status"=w1381:refnum<notifier>)
                    n693 = Select(t="Play", s=TRUE, f="Pause") -> (s? t:f=w1380:string)
                    n694 = Send Notification(notification=w1380, notifier=w1381) -> ()  [unwired: 1 in, 2 out]
                  }
                  frame #1 {
                    n695 = Wait (ms)(milliseconds to wait=u32 1500) -> ()  [unwired: 1 out]
                  }
                  frame #2 {
                    n696 = global read "SW_Globals.vi" "Zones allocation array"() -> (w1388:i32[])
                    n697 = Array Size(array=w1388) -> (size(s)=w1387:i32)
                    n698 = Initialize Array(0 ("element"), w1387) -> (w1390:i32[])
                    n699 = global write "SW_Globals.vi" "Zones allocation array"(w1390) -> ()
                  }
                }
                n700 = property on="Pane" class="Pane"(error in=w1275) -> (error out=w1274:errorcluster, "Decos[]"=w1276:refnum<vi>[])  [unwired: 1 in, 1 out]
                n701 = Index Array(array=w1276, index=2) -> (element=w1281:refnum<vi>)
                n702 = property class="Decor"(reference=w1281, error in=w1274, "Visible"=FALSE) -> (error out=w1273:errorcluster)  [unwired: 1 out]
                n703 = Index Array(array=w1276, index=1) -> (element=w1278:refnum<vi>)
                n704 = property class="Decor"(reference=w1278, error in=w1273, "Visible"=TRUE) -> (error out=w1272:errorcluster)  [unwired: 1 out]
                n705 = property on="Main tab control" class="TabCtl (strict)"(error in=w1272, "Value"=w1347) -> (error out=w1343:errorcluster, "Pages"=w1348:refnum<vi>[])  [unwired: 1 in, 1 out]
                n706 = To Long Integer(number=w1347) -> (32bit integer=w1346:i32)
                n707 = Index Array(array=w1348, index=w1346) -> (element=w1345:refnum<vi>)
                n708 = property class="Page"(reference=w1345, error in=w1343, "PageEnb"=T26."Page Disabled & Grayed" ("Page Enabled State")) -> (error out=w1336:errorcluster)  [unwired: 1 out]
                n709 = property on="Main tab control" class="TabCtl (strict)"(error in=w1336, "Value"=w1338) -> (error out=w1342:errorcluster, "Pages"=w1337:refnum<vi>[])  [unwired: 1 in, 1 out]
                n710 = To Long Integer(number=w1338) -> (32bit integer=w1339:i32)
                n711 = Index Array(array=w1337, index=w1339) -> (element=w1340:refnum<vi>)
                n712 = property class="Page"(reference=w1340, error in=w1342, "PageEnb"=T26."Page Disabled & Grayed" ("Page Enabled State")) -> (error out=w1329:errorcluster)  [unwired: 1 out]
                n713 = property on="Main tab control" class="TabCtl (strict)"(error in=w1329, "Value"=w1334) -> (error out=w1330:errorcluster, "Pages"=w1335:refnum<vi>[])  [unwired: 1 in, 1 out]
                n714 = To Long Integer(number=w1334) -> (32bit integer=w1333:i32)
                n715 = local read "Settings file refnum out"() -> (w1328:T3)
                n716 = local read "N segments MIDFIELD"() -> (w1326:u8)
                n717 = Index Array(array=w1335, index=w1333) -> (element=w1332:refnum<vi>)
                n718 = local read "Current User"() -> (w1250:string)
                n719 = local read "N segments BORDER"() -> (w1321:u8)
                n720 = property class="Page"(reference=w1332, error in=w1330, "PageEnb"=T26."Page Enabled" ("Page Enabled State")) -> (error out=w1325:errorcluster)  [unwired: 1 out]
                n721 = local read "Radius, mm CENTER"() -> (w1320:u16)
                n722 = call <vilib>:"Write Key (I32).vi"("section"=w1250, "error in (no error)"=w1325, "value"=w1326, "key"="Amount of midfield segments", "refnum"=w1328) -> ("error out"=w1323:errorcluster, "refnum out"=w1322:T3)  [unwired: 4 in, 1 out]
                n723 = local read "Radius, mm MIDFIELD"() -> (w1313:u16)
                n724 = call <vilib>:"Write Key (I32).vi"("section"=w1250, "error in (no error)"=w1323, "value"=w1321, "key"="Amount of border segments", "refnum"=w1322) -> ("error out"=w1317:errorcluster, "refnum out"=w1318:T3)  [unwired: 4 in, 1 out]
                n725 = local read "Starting angle MIDFIELD"() -> (w1312:i16)
                n726 = call <vilib>:"Write Key (I32).vi"("section"=w1250, "error in (no error)"=w1317, "value"=w1320, "key"="Center segment outer radius, mm", "refnum"=w1318) -> ("error out"=w1314:errorcluster, "refnum out"=w1315:T3)  [unwired: 4 in, 1 out]
                n727 = local read "Starting angle BORDER"() -> (w1305:i16)
                n728 = call <vilib>:"Write Key (I32).vi"("section"=w1250, "error in (no error)"=w1314, "value"=w1313, "key"="Midfield segments outer radius, mm", "refnum"=w1315) -> ("error out"=w1309:errorcluster, "refnum out"=w1310:T3)  [unwired: 4 in, 1 out]
                n729 = local read "Cage diameter, mm"() -> (w1284:u16)
                n730 = call <vilib>:"Write Key (I32).vi"("section"=w1250, "error in (no error)"=w1309, "value"=w1312, "key"="Midfield segments starting angle", "refnum"=w1310) -> ("error out"=w1307:errorcluster, "refnum out"=w1306:T3)  [unwired: 4 in, 1 out]
                n731 = call <vilib>:"Write Key (I32).vi"("section"=w1250, "error in (no error)"=w1307, "value"=w1305, "key"="Border segments starting angle", "refnum"=w1306) -> ("error out"=w1304:errorcluster, "refnum out"=w1303:T3)  [unwired: 4 in, 1 out]
                n732 = call <vilib>:"Write Key (I32).vi"("section"=w1250, "error in (no error)"=w1304, "value"=w1284, "key"="Cage diameter, mm", "refnum"=w1303) -> ("error out"=w1243:errorcluster, "refnum out"=w1244:T3)  [unwired: 4 in, 1 out]
                n733 = property on="Stimulus presets" class="Arr (strict)"(error in=w1243) -> (error out=w1247:errorcluster, "Value"=w1283:T5)  [unwired: 1 in, 1 out]
                n734 = for {
                  tunnel: w1283 -> [w1361] mode=indexing
                  tunnel: w1244 -> [w1354]
                  tunnel: [w1358] -> w1253
                  tunnel: w1250 -> [w1352]
                  i -> [w1357]
                  n735 = Unbundle By Name(w1361) -> ("Stim. has been set"=w1359:bool)
                  n736 = Flatten To JSON(anything=w1361) -> (JSON string=w1360:string, 11:w1350:errorcluster)  [unwired: 2 in]
                  n737 = Format Value(string ("")="Zone " ("string"), format string="%02d", value (0)=w1357) -> (output string=w1351:string)
                  n738 = call <vilib>:"Remove Key.vi"("section"=w1352, "error in (no error)"=w1350, "key"=w1351, "refnum"=w1354) -> ("error out"=w1349:errorcluster, "refnum out"=w1353:T3)  [unwired: 5 in, 1 out]
                  n739 = case shown="True" w1359 {
                    tunnel: w1360 -> [_ w1368]
                    tunnel: w1349 -> [_ w1367]
                    tunnel: [w1362 w1366] -> w1358
                    tunnel: w1352 -> [_ w1365]
                    tunnel: w1351 -> [_ w1364]
                    tunnel: w1353 -> [w1362 w1363]
                    frame False {
                    }
                    frame True {
                      n740 = call <vilib>:"Write Key (String).vi"("section"=w1365, "error in (no error)"=w1367, "value"=w1368, "key"=w1364, "refnum"=w1363) -> ("refnum out"=w1366:T3)  [unwired: 4 in, 2 out]
                    }
                  }
                }
                n741 = property on="IO parameters string" class="Str"(error in=w1247) -> (error out=w1246:errorcluster, "Value"=w1248:string)  [unwired: 1 in, 1 out]
                n742 = local read "Starting angle MIDFIELD"() -> (w1260:i16)
                n743 = local read "Starting angle BORDER"() -> (w1261:i16)
                n744 = local read "N segments MIDFIELD"() -> (w1255:u8)
                n745 = local read "Radius, mm MIDFIELD"() -> (w1259:u16)
                n746 = local read "N segments BORDER"() -> (w1256:u8)
                n747 = local read "Radius, mm CENTER"() -> (w1257:u16)
                n748 = local read "Cage diameter, mm"() -> (w1254:u16)
                n749 = call <vilib>:"Write Key (String).vi"("section"=w1250, "error in (no error)"=w1246, "value"=w1248, "key"="IO ports configuration", "refnum"=w1253) -> ("error out"=w1252:errorcluster, "refnum out"=w1251:T3)  [unwired: 4 in, 1 out]
                n750 = call <vilib>:"Close Config Data.vi"("error in (no error)"=w1252, "refnum"=w1251) -> ("error out"=w1301:errorcluster)  [unwired: 8 in, 1 out]
                n751 = property on="Zones presence indicator" class="Clust"() -> ("Controls[]"=w1297:refnum<vi>[])  [unwired: 2 in, 2 out]
                n752 = property on="Diagram at recording" class="Pict"(error in=w1301) -> ("Bounds"=w1271:T14)  [unwired: 1 in, 2 out]
                n753 = Compound Arithmetic op=ADD(w1256, w1255, u8 1 ("value")) -> (w1293:u8)
                n754 = Bundle By Name(cluster=T15 {"Amount of border segments"=8, "Border segments starting angle"=0, "Amount of midfield segments"=4, "Midfield segments starting angle"=0, "Midfield segments outer radius, mm"=60, "Amount of central segments"=1, "Center segment outer radius, mm"=30, "Diameter of the cage, mm"=180, "R-gap between segments, mm"=10} ("Input cluster of parameters"), "Amount of border segments"=w1256, "Border segments starting angle"=w1261, "Amount of midfield segments"=w1255, "Midfield segments starting angle"=w1260, "Midfield segments outer radius, mm"=w1259, "Amount of central segments"=u8 1, "Center segment outer radius, mm"=w1257, "Diameter of the cage, mm"=w1254) -> (w1262:T15)
                n755 = for {
                  tunnel: w1297 -> [w1376] mode=indexing
                  tunnel: w1293 -> [w1370]
                  i -> [w1375]
                  n756 = Increment(x=w1375) -> (x+1=w1369:i32)
                  n757 = Less Or Equal?(x=w1369, y=w1370) -> (x <= y?=w1374:bool)
                  n758 = Select(t=T9."Disabled" ("Disabled"), s=w1374, f=T9."Disabled and Grayed Out" ("Disabled")) -> (s? t:f=w1372:T9)
                  n759 = property class="Ctl"(reference=w1376, "DisabledEnum"=w1372) -> ()  [unwired: 1 in, 2 out]
                }
                n760 = global write "SW_Globals.vi" "Active segments amount"(w1293) -> ()
                n761 = Increment(x=w1293) -> (x+1=w1292:u8)
                n762 = global read "SW_Globals.vi" "Regions to track"() -> (w1270:u8[])
                n763 = call "SW_Generate_Segmented_Plot_v3.vi"("Draw Area Size"=w1271, "Regions to mark set"=w1270, "Input cluster of parameters"=w1262) -> ("Zones layout output"=w1268:picture, "No zones image"=w1269:picture, "Array of the pixel to color correspondences"=w1264:u32[][], "Array of the segment to color correspondences"=w1267:u32[][], "Cluster of image geometrical and scaling parameters"=w1266:T22)  [unwired: 7 in, 1 out]
                n764 = global write "SW_Globals.vi" "Diagram"(w1268) -> ()
                n765 = local write "Diagram at recording"(w1268) -> ()
                n766 = global write "SW_Globals.vi" "Diagram no zones"(w1269) -> ()
                n767 = global write "SW_Globals.vi" "Array of the pixel to color correspondences"(w1264) -> ()
                n768 = global write "SW_Globals.vi" "Array of the segment to color correspondences"(w1267) -> ()
                n769 = Unbundle By Name(w1266) -> ("Pixels per mm"=→"Pixels per mm":dbl)
                n770 = Bundle By Name(cluster=T16 {"Minimum"=0.0, "Maximum"=14.0, "Increment"=1.0, "Minor Increment"=1.0, "Start"=0.0} ("X Scale.Range"), "Maximum"=w1292) -> (w1294:T16)
                n771 = Array Size(array=w1264) -> (size(s)=w1289:i32[])
                n772 = property on="Zone preference (normalized)" class="WFGraph (strict)"("XScale.Range"=w1294) -> ()  [unwired: 2 in, 2 out]
                n773 = Index Array(array=w1289, index=0) -> (element=w1288:i32)
                n774 = Index Array(array=w1289, index=1) -> (element=w1287:i32)
                n775 = Initialize Array(u32 0 ("element"), w1288, w1287) -> (w1285:u32[][])
                n776 = global write "SW_Globals.vi" "Array of the presence count"(w1285) -> ()
              }
              frame 2 {
                w1401 = T9."Disabled and Grayed Out" ("Disabled")
                w1411 = enum32{"Settings", "Recording", "Analysis"}."Analysis" ("Main tab control")
                w1415 = enum32{"Settings", "Recording", "Analysis"}."Recording" ("Main tab control")
                w1424 = enum32{"Settings", "Recording", "Analysis"}."Settings" ("Main tab control")
                n777 = property on="Main tab control" class="TabCtl (strict)"(error in=w1405, "Value"=w1424) -> (error out=w1420:errorcluster, "Pages"=w1425:refnum<vi>[])  [unwired: 1 in, 1 out]
                n778 = To Long Integer(number=w1424) -> (32bit integer=w1423:i32)
                n779 = Index Array(array=w1425, index=w1423) -> (element=w1422:refnum<vi>)
                n780 = property class="Page"(reference=w1422, error in=w1420, "PageEnb"=T26."Page Disabled & Grayed" ("Page Enabled State")) -> (error out=w1413:errorcluster)  [unwired: 1 out]
                n781 = property on="Main tab control" class="TabCtl (strict)"(error in=w1413, "Value"=w1415) -> (error out=w1419:errorcluster, "Pages"=w1414:refnum<vi>[])  [unwired: 1 in, 1 out]
                n782 = To Long Integer(number=w1415) -> (32bit integer=w1416:i32)
                n783 = Index Array(array=w1414, index=w1416) -> (element=w1417:refnum<vi>)
                n784 = property class="Page"(reference=w1417, error in=w1419, "PageEnb"=T26."Page Disabled & Grayed" ("Page Enabled State")) -> (error out=w1406:errorcluster)  [unwired: 1 out]
                n785 = property on="Main tab control" class="TabCtl (strict)"(error in=w1406, "Value"=w1411) -> (error out=w1407:errorcluster, "Pages"=w1412:refnum<vi>[])  [unwired: 1 in, 1 out]
                n786 = To Long Integer(number=w1411) -> (32bit integer=w1410:i32)
                n787 = Index Array(array=w1412, index=w1410) -> (element=w1409:refnum<vi>)
                n788 = property class="Page"(reference=w1409, error in=w1407, "PageEnb"=T26."Page Enabled" ("Page Enabled State")) -> (error out=w1404:errorcluster)  [unwired: 1 out]
                n789 = property on="Zones (analysis)" class="Bool (strict)"(error in=w1404, "Value"=FALSE ("Zones an."), "DisabledEnum"=w1401) -> (error out=w1402:errorcluster)  [unwired: 1 in, 1 out]
                n790 = property on="Play/Pause" class="Bool (strict)"(error in=w1402, "DisabledEnum"=w1401) -> (error out=w1400:errorcluster)  [unwired: 1 in, 1 out]
                n791 = property on="Back to Settings" class="Bool"(error in=w1400, "Visible"=FALSE) -> (error out=w1395:errorcluster)  [unwired: 1 in, 1 out]
                n792 = property on="Pane" class="Pane"(error in=w1395) -> ("Decos[]"=w1391:refnum<vi>[])  [unwired: 1 in, 2 out]
                n793 = Index Array(array=w1391, index=0) -> (element=w1393:refnum<vi>)
                n794 = Index Array(array=w1391, index=2) -> (element=w1397:refnum<vi>)
                n795 = property class="Decor"(reference=w1393, "Visible"=TRUE) -> ()  [unwired: 1 in, 2 out]
                n796 = property class="Decor"(reference=w1397, "Visible"=FALSE) -> ()  [unwired: 1 in, 2 out]
              }
            }
          }
        }
      }
      frame "Recording" {
        w1466 = FALSE ("use system decimal point (T)")
        n797 = global read "SW_Globals.vi" "Zones normalized allocation array"() -> (→"Zone preference (normalized)":dbl[])
        n798 = global read "SW_Globals.vi" "Zones presence indicator"() -> (w1427:T36)
        n799 = call <extravilib>:"Read.vi"("channel"=w1492) -> ("element"=w1430:string[][])  [unwired: 5 in, 5 out]
        n800 = Divide(x=u32 1000, y=w1505) -> (x/y=w1504:dbl)
        n801 = property on="Zones presence indicator" class="Clust"("Value"=w1427) -> ()  [unwired: 2 in, 2 out]
        n802 = call "FL_Last_N_Samples_2D_array_of_strings.vi"("BufferLengthSamples"=u32 5, "Input Array of strings"=w1430) -> ("Output Array of strings"=w1429:string[][])
        n803 = event shown="[1] \"Multiplyer of chart RX\": Value Change" {
          selector: _ -> [_ _]
          dyn-events: _ -> [_ _]
          timeout: 1 -> [_ _]
          event Timeout {
            n804 = event-data() -> ()  [unwired: 1 in, 3 out]
          }
          event "Multiplyer of chart RX": Value Change {
            n805 = event-data() -> ("NewVal"=w1527:u8)  [unwired: 1 in, 5 out]
            n806 = Multiply(x=w1527, y=10.0) -> (x*y=w1528:dbl)
            n807 = property on="Mouse speed" class="WFChart (strict)"() -> (error out=w1529:errorcluster, "XScale.Maximum"=w1532:dbl)  [unwired: 2 in, 1 out]
            n808 = Subtract(x=w1532, y=w1528) -> (x-y=w1530:dbl)
            n809 = property on="Mouse speed" class="WFChart (strict)"(error in=w1529, "XScale.Minimum"=w1530) -> ()  [unwired: 1 in, 2 out]
          }
        }
        n810 = Multiply(x=w1504, y="Trace, s") -> (x*y=w1508:dbl)
        n811 = Array Size(array=w1429) -> (size(s)=w1482:i32[])
        n812 = Index Array(array=w1482, index=0) -> (element=w1480:i32)
        n813 = Decrement(x=w1480) -> (x-1=w1479:i32)
        n814 = Round To Nearest(number=w1508) -> (nearest integer value=w1507:dbl)
        n815 = Index Array(array=w1429, index (row)=w1479) -> (element=w1471:string[])  [unwired: 1 in]
        n816 = global read "SW_Globals.vi" "Diagram no zones"() -> (w1514:picture)
        n817 = Index Array "w (mouse rot. angle)"(array=w1471, index=8) -> (element=w1467:string)
        n818 = Index Array "X (filtered)"(array=w1471, index=9) -> (element=w1469:string)
        n819 = Index Array "Y (filtered)"(array=w1471, index=10) -> (element=w1468:string)
        n820 = Index Array "Timestamp"(array=w1471, index=4) -> (element=w1477:string)
        n821 = global read "SW_Globals.vi" "Diagram"() -> (w1515:picture)
        n822 = Select(t=w1515, s="Zones", f=w1514) -> (s? t:f=w1516:picture)
        n823 = Not(x="Zones") -> (.not. x?=w1510:bool)
        n824 = String Length(string=w1477) -> (length=w1476:i32)
        n825 = Fract/Exp String To Number(use system decimal point (T)=w1466, string=w1467) -> (number=w1465:dbl)  [unwired: 2 in, 1 out]
        n826 = Fract/Exp String To Number(use system decimal point (T)=w1466, string=w1469) -> (number=w1454:dbl)  [unwired: 2 in, 1 out]
        n827 = Fract/Exp String To Number(use system decimal point (T)=w1466, string=w1468) -> (number=w1452:dbl)  [unwired: 2 in, 1 out]
        n828 = property on="Diagram at recording" class="Pict"() -> ("Bounds"=w1512:T14)  [unwired: 2 in, 2 out]
        n829 = local read "Pixels per mm"() -> (w1513:dbl)
        n830 = Greater Than 0?(x=w1476) -> (x > 0?=w1475:bool)
        n831 = Build Array(w1454) -> (w1455:dbl[])
        n832 = Build Array(w1452) -> (w1453:dbl[])
        n833 = case shown="True" w1475 {
          tunnel: [w1517 w1520] -> w1474
          tunnel: w1477 -> [_ w1519]
          frame False {
            n834 = Get Date/Time In Seconds() -> (seconds since 1Jan1904=w1517:timestamp)
          }
          frame True {
            n835 = Get Date/Time In Seconds() -> (seconds since 1Jan1904=w1518:timestamp)
            n836 = Scan From String(format string="%<%H:%M:%S%3u%p%d.%m.%Y>T", input string=w1519, default 1=w1518) -> (output 1=w1520:timestamp)  [unwired: 2 in, 3 out]
          }
        }
        n837 = call "SW_Draw_mouse_br.vi"("Input picture (background)"=w1516, "Size of the image"=w1512, "Pixels per mm"=w1513, "Mouse coord cartesian X, mm"=w1454, "Mouse coord cartesian Y, mm"=w1452, "Mouse angle of rotation, deg"=w1465, "Show mouse lineout"=w1510, "Trace length, samples"=w1507) -> ("Output picture (with mouse overlay)"=→"Diagram at recording":picture)  [unwired: 6 in, 1 out]
        n838 = call "FL_Last_N_Samples_1D.vi"("BufferLengthSamples"="SD calc buffer length", "Input Array of strings"=w1455) -> ("Output Array of strings"=w1490:dbl[])
        n839 = call "FL_Last_N_Samples_1D.vi"("BufferLengthSamples"="SD calc buffer length", "Input Array of strings"=w1453) -> ("Output Array of strings"=w1489:dbl[])
        n840 = call <vilib>:"Std Deviation and Variance.vi"("X"=w1490) -> ("mean"=w1459:dbl, "standard deviation"=w1464:dbl)  [unwired: 1 in, 1 out]
        n841 = call <vilib>:"Std Deviation and Variance.vi"("X"=w1489) -> ("mean"=w1445:dbl, "standard deviation"=w1444:dbl)  [unwired: 1 in, 1 out]
        n842 = Square Root(x=1.0) -> (sqrt(x)=w1463:dbl)
        n843 = Square Root(x=1.0) -> (sqrt(x)=w1446:dbl)
        n844 = Divide(x=w1464, y=w1463) -> (x/y=w1462:dbl)
        n845 = Divide(x=w1444, y=w1446) -> (x/y=w1447:dbl)
        n846 = Multiply(x=w1462, y=1.96) -> (x*y=w1460:dbl)
        n847 = Multiply(x=w1447, y=1.96) -> (x*y=w1449:dbl)
        n848 = Add(x=w1459, y=w1460) -> (x+y=w1457:dbl)
        n849 = Subtract(x=w1459, y=w1460) -> (x-y=w1458:dbl)
        n850 = Add(x=w1445, y=w1449) -> (x+y=w1451:dbl)
        n851 = Subtract(x=w1445, y=w1449) -> (x-y=w1450:dbl)
        n852 = Subtract(x=w1457, y=w1458) -> (x-y=w1442:dbl)
        n853 = Subtract(x=w1451, y=w1450) -> (x-y=w1441:dbl)
        n854 = Tick Count (ms)() -> (millisecond timer value=w1502:u32)
        n855 = Square(x=w1442) -> (x^2=w1440:dbl)
        n856 = Square(x=w1441) -> (x^2=w1439:dbl)
        n857 = Add(x=w1440, y=w1439) -> (x+y=w1438:dbl)
        n858 = Not(x="Exit 2") -> (.not. x?=w1485:bool)
        n859 = Square Root(x=w1438) -> (sqrt(x)=w1437:dbl)
        n860 = Divide(x=w1437, y=2.0) -> (x/y=→"Estim. res":dbl)
        n861 = property on="Current Time" class="AbsTime (strict)"("Value"=w1474) -> ()  [unwired: 2 in, 2 out]
        n862 = And(x=w1485, y="Record/Stop") -> (x .and. y?=w1486:bool)
        n863 = case shown="True" w1486 {
          tunnel: w1488 -> [w1534 w1621]
          tunnel: w1474 -> [_ w1619]
          tunnel: [w1537 w1620] -> _
          tunnel: w1503 -> [_ w1618]
          tunnel: [w1536 w1616] -> w1494
          tunnel: "Exit 2" -> [w1533 _]
          frame False {
            n864 = Unbundle By Name(w1534) -> ("Has been recorded"=w1540:refnum<notifier>)
            n865 = Get Notifier Status(notifier=w1540) -> (current notification=w1539:bool, error out=w1538:errorcluster)  [unwired: 1 in, 3 out]
            n866 = Or(x=w1533, y=w1539) -> (x .or. y?=w1535:bool)
            n867 = case shown="True" w1535 {
              tunnel: w1534 -> [_ w1604]
              tunnel: w1538 -> [_ w1583]
              tunnel: [w1551 w1577] -> w1537
              tunnel: [FALSE FALSE] -> w1536
              frame False {
                n868 = global read "SW_Globals.vi" "Cluster of paths"() -> (w1552:T18)
                n869 = Unbundle By Name(w1552) -> ("Temporary file output path"=w1551:path, "Path to the settings file"=w1542:path)
                n870 = local read "Current User"() -> (w1541:string)
                n871 = property on="Bridge swap" class="Bool (strict)" props=["Value"]() -> (error out=w1543:errorcluster)  [unwired: 2 in, 2 out]
                n872 = call <vilib>:"Open Config Data.vi"("error in (no error)"=w1543, "create file if necessary (T)"=FALSE, "configuration file path"=w1542) -> ("error out"=w1547:errorcluster, "refnum"=w1549:T3)  [unwired: 6 in, 1 out]
                n873 = call <vilib>:"Write Key (Boolean).vi"("section"=w1541, "error in (no error)"=w1547, "key"="Mouse snout orientation swap?", "refnum"=w1549) -> ("error out"=w1546:errorcluster, "refnum out"=w1548:T3)  [unwired: 5 in, 1 out]
                n874 = call <vilib>:"Close Config Data.vi"("error in (no error)"=w1546, "refnum"=w1548) -> ()  [unwired: 8 in, 2 out]
              }
              frame True {
                w1589 = enum32{"Settings", "Recording", "Analysis"}."Analysis" ("Main tab control")
                w1593 = enum32{"Settings", "Recording", "Analysis"}."Recording" ("Main tab control")
                w1602 = enum32{"Settings", "Recording", "Analysis"}."Settings" ("Main tab control")
                n875 = flat-sequence {
                  tunnel: w1604 -> [w1612]
                  tunnel: w1583 -> [w1608]
                  tunnel: [w1605] -> w1582
                  tunnel: [w1614] -> w1581
                  tunnel: w1582 -> [w1614]
                  frame #0 {
                    n876 = Unbundle By Name(w1612) -> ("Play/Pause status"=w1613:refnum<notifier>, "Recording now"=w1610:refnum<notifier>)
                    n877 = Send Notification(notification=FALSE, notifier=w1610, error in (no error)=w1608) -> (error out=w1606:errorcluster)  [unwired: 1 out]
                    n878 = Send Notification(notification="Pause" ("f"), notifier=w1613) -> (error out=w1607:errorcluster)  [unwired: 1 in, 1 out]
                    n879 = Merge Errors(w1607, w1606) -> (w1605:errorcluster)
                  }
                  frame #1 {
                    n880 = Wait (ms)(milliseconds to wait=u32 500) -> ()  [unwired: 1 out]
                  }
                }
                n881 = property on="Exit 2" class="Bool"(error in=w1581, "DisabledEnum"=T9."Enabled" ("Disabled")) -> (error out=w1580:errorcluster)  [unwired: 1 in, 1 out]
                n882 = property on="Main tab control" class="TabCtl (strict)"(error in=w1580, "Value"=w1602) -> (error out=w1598:errorcluster, "Pages"=w1603:refnum<vi>[])  [unwired: 1 in, 1 out]
                n883 = To Long Integer(number=w1602) -> (32bit integer=w1601:i32)
                n884 = Index Array(array=w1603, index=w1601) -> (element=w1600:refnum<vi>)
                n885 = property class="Page"(reference=w1600, error in=w1598, "PageEnb"=T26."Page Disabled & Grayed" ("Page Enabled State")) -> (error out=w1591:errorcluster)  [unwired: 1 out]
                n886 = property on="Main tab control" class="TabCtl (strict)"(error in=w1591, "Value"=w1593) -> (error out=w1597:errorcluster, "Pages"=w1592:refnum<vi>[])  [unwired: 1 in, 1 out]
                n887 = To Long Integer(number=w1593) -> (32bit integer=w1594:i32)
                n888 = Index Array(array=w1592, index=w1594) -> (element=w1595:refnum<vi>)
                n889 = property class="Page"(reference=w1595, error in=w1597, "PageEnb"=T26."Page Disabled & Grayed" ("Page Enabled State")) -> (error out=w1584:errorcluster)  [unwired: 1 out]
                n890 = property on="Main tab control" class="TabCtl (strict)"(error in=w1584, "Value"=w1589) -> (error out=w1585:errorcluster, "Pages"=w1590:refnum<vi>[])  [unwired: 1 in, 1 out]
                n891 = To Long Integer(number=w1589) -> (32bit integer=w1588:i32)
                n892 = Index Array(array=w1590, index=w1588) -> (element=w1587:refnum<vi>)
                n893 = property class="Page"(reference=w1587, error in=w1585, "PageEnb"=T26."Page Enabled" ("Page Enabled State")) -> (error out=w1556:errorcluster)  [unwired: 1 out]
                n894 = property on="Pane" class="Pane"(error in=w1556) -> (error out=w1555:errorcluster, "Decos[]"=w1557:refnum<vi>[])  [unwired: 1 in, 1 out]
                n895 = Index Array(array=w1557, index=1) -> (element=w1562:refnum<vi>)
                n896 = property class="Decor"(reference=w1562, error in=w1555, "Visible"=FALSE) -> (error out=w1554:errorcluster)  [unwired: 1 out]
                n897 = Index Array(array=w1557, index=0) -> (element=w1559:refnum<vi>)
                n898 = property class="Decor"(reference=w1559, error in=w1554, "Visible"=TRUE) -> (error out=w1553:errorcluster)  [unwired: 1 out]
                n899 = global read "SW_Globals.vi" "Cluster of paths"() -> (w1578:T18)
                n900 = property on="Back to Settings" class="Bool"(error in=w1553, "Visible"=FALSE) -> (error out=w1565:errorcluster)  [unwired: 1 in, 1 out]
                n901 = Unbundle By Name(w1578) -> ("Temporary file output path"=w1577:path, "Path to the settings file"=w1571:path)
                n902 = property on="Bridge swap" class="Bool (strict)"(error in=w1565) -> (error out=w1568:errorcluster, "Value"=w1567:bool)  [unwired: 1 in, 1 out]
                n903 = local read "Current User"() -> (w1566:string)
                n904 = call <vilib>:"Open Config Data.vi"("error in (no error)"=w1568, "create file if necessary (T)"=FALSE, "configuration file path"=w1571) -> ("error out"=w1573:errorcluster, "refnum"=w1575:T3)  [unwired: 6 in, 1 out]
                n905 = call <vilib>:"Write Key (Boolean).vi"("section"=w1566, "error in (no error)"=w1573, "value"=w1567, "key"="Mouse snout orientation swap?", "refnum"=w1575) -> ("error out"=w1572:errorcluster, "refnum out"=w1574:T3)  [unwired: 4 in, 1 out]
                n906 = call <vilib>:"Close Config Data.vi"("error in (no error)"=w1572, "refnum"=w1574) -> ()  [unwired: 8 in, 2 out]
              }
            }
          }
          frame True {
            n907 = flat-sequence {
              tunnel: w1619 -> [w1625]
              tunnel: [w1633] -> w1622
              tunnel: w1621 -> [w1630]
              tunnel: [w1628] -> w1620
              tunnel: w1619 -> [w1627]
              tunnel: [w1627] -> w1617
              tunnel: w1618 -> [w1626]
              tunnel: [w1624] -> w1616
              frame #0 {
                n908 = First Call?() -> (First Call?: T/F=w1636:bool)
                n909 = case shown="True" w1636 {
                  tunnel: w1625 -> [_ w1658]
                  tunnel: [w1642 w1658] -> w1633
                  tunnel: [w1640 w1656] -> w1628
                  tunnel: [_ w1647] -> w1629
                  tunnel: w1626 -> [_ w1655]
                  tunnel: [FALSE TRUE] -> w1624
                  frame False {
                    n910 = global read "SW_Globals.vi" "Cluster of paths"() -> (w1641:T18)
                    n911 = global read "SW_Globals.vi" "Recording start timestamp"() -> (w1642:timestamp)
                    n912 = Unbundle By Name(w1641) -> ("Temporary file output path"=w1640:path)
                  }
                  frame True {
                    w1646 = T9."Disabled and Grayed Out" ("Disabled")
                    n913 = global read "SW_Globals.vi" "Cluster of paths"() -> (w1649:T18)
                    n914 = Flush Queue(queue=w1655) -> (error out=w1653:errorcluster)  [unwired: 1 in, 2 out]
                    n915 = call "SW_Get_save_paths.vi"("Input cluster of paths"=w1649) -> ("error out"=w1652:errorcluster, "Output cluster of paths"=w1657:T37)  [unwired: 4 in]
                    n916 = global write "SW_Globals.vi" "Cluster of paths"(w1657) -> ()
                    n917 = Unbundle By Name(w1657) -> ("Temporary file output path"=w1656:path)
                    n918 = Merge Errors(w1653, w1652) -> (w1645:errorcluster)
                    n919 = property on="Data filtering" class="Ring (strict)"(error in=w1645, "DisabledEnum"=T9."Disabled and Grayed Out" ("Disabled")) -> (error out=w1644:errorcluster)  [unwired: 1 in, 1 out]
                    n920 = property on="Exit 2" class="Bool"(error in=w1644, "DisabledEnum"=T9."Enabled" ("Disabled")) -> (error out=w1651:errorcluster)  [unwired: 1 in, 1 out]
                    n921 = property on="Bridge swap" class="Bool (strict)"(error in=w1651, "DisabledEnum"=w1646) -> (error out=w1648:errorcluster)  [unwired: 1 in, 1 out]
                    n922 = property on="Vertical offset" class="DigNum (strict)"(error in=w1648, "DisabledEnum"=w1646) -> (error out=w1647:errorcluster)  [unwired: 1 in, 1 out]
                  }
                }
                n923 = Unbundle By Name(w1630) -> ("Recording now"=w1632:refnum<notifier>, "Has been recorded"=w1638:refnum<notifier>)
                n924 = Send Notification(notification=TRUE, notifier=w1632, error in (no error)=w1629) -> ()  [unwired: 2 out]
                n925 = Send Notification(notification=TRUE, notifier=w1638, error in (no error)=w1629) -> (error out=w1634:errorcluster)  [unwired: 1 out]
                n926 = property on="Record timestamp" class="DigNum (strict)"(error in=w1634, "DisabledEnum"=T9."Enabled" ("Disabled")) -> ()  [unwired: 1 in, 2 out]
              }
            }
            n927 = Subtract(x=w1617, y=w1622) -> (x-y=→"Record timestamp":dbl)
          }
        }
        n928 = case shown="True" w1494 {
          frame False {
          }
          frame True {
            w1522 = waveform(dbl)[] [] ("History Data")
            n929 = property on="Mouse speed" class="WFChart (strict)"("History Data"=w1522) -> ()  [unwired: 2 in, 2 out]
            n930 = property on="Mouse speed 2" class="WFChart (strict)"("History Data"=w1522) -> ()  [unwired: 2 in, 2 out]
          }
        }
        n931 = Or(x="Reset barplot", y=w1494) -> (x .or. y?=w1495:bool)
        n932 = case shown="True" w1495 {
          frame False {
          }
          frame True {
            n933 = global read "SW_Globals.vi" "Zones allocation array"() -> (w1524:i32[])
            n934 = Array Size(array=w1524) -> (size(s)=w1526:i32)
            n935 = Initialize Array(0 ("element"), w1526) -> (w1523:i32[])
            n936 = global write "SW_Globals.vi" "Zones allocation array"(w1523) -> ()
          }
        }
        n937 = feedback-in #4(w1502) -> ()
        n938 = feedback #4(w1500) -> (w1501:u32)
        n939 = Subtract(x=w1502, y=w1501) -> (x-y=w1499:u32)
        n940 = Divide(x=w1499, y=u32 1000) -> (x/y=w1493:dbl)
        n941 = Reciprocal(x=w1493) -> (1/x=→"FPS":dbl)
        n942 = call "FL_Calc_speed_on_the_fly.vi"("Y coord, mm"=w1452, "X coord, mm"=w1454, "Time per frame, s"=w1493) -> ("Mouse speed, mm/s"=w1431:dbl)
        "Mouse speed digi" <- w1431
        n943 = Build Array(w1431) -> (w1491:dbl[])
        n944 = Bundle By Name("t0"=w1474, "Y"=w1491) -> (→"Mouse speed":waveform(dbl))  [unwired: 1 in]
      }
      frame "Analysis" {
        n945 = Unbundle By Name(w1672) -> ("Has been recorded"=w1674:refnum<notifier>)
        n946 = Unbundle By Name(w1672) -> ("Data loaded"=w1681:refnum<notifier>)
        n947 = disable-structure shown="Disabled" {
          frame Disabled {
            n948 = event shown="[0] Timeout" {
              selector: _ -> [_ _ _]
              dyn-events: _ -> [_ _ _]
              timeout: 1 -> [_ _ _]
              event Timeout {
                n949 = event-data() -> ()  [unwired: 1 in, 3 out]
              }
              event "Play/Pause": Value Change {
                n950 = event-data() -> ("NewVal"=w1702:bool)  [unwired: 1 in, 5 out]
                n951 = case shown="True" w1702 {
                  frame False {
                    n952 = property on="Back to Settings" class="Bool"("DisabledEnum"=T9."Enabled" ("Disabled")) -> ()  [unwired: 2 in, 2 out]
                  }
                  frame True {
                    n953 = property on="Back to Settings" class="Bool"("DisabledEnum"=T9."Disabled and Grayed Out" ("Disabled")) -> ()  [unwired: 2 in, 2 out]
                  }
                }
              }
              event "Back to Settings": Value Change {
                n954 = event-data() -> ("NewVal"=w1705:bool)  [unwired: 1 in, 5 out]
                n955 = case shown="True" w1705 {
                  frame False {
                  }
                  frame True {
                    w1723 = enum32{"Settings", "Recording", "Analysis"}."Settings" ("Main tab control")
                    w1719 = enum32{"Settings", "Recording", "Analysis"}."Recording" ("Main tab control")
                    w1710 = enum32{"Settings", "Recording", "Analysis"}."Analysis" ("Main tab control")
                    n956 = property on="Diagram at recording" class="Pict"() -> ("Bounds"=w1708:T14)  [unwired: 2 in, 2 out]
                    n957 = property on="Main tab control" class="TabCtl (strict)"("Value"=w1710) -> (error out=w1714:errorcluster, "Pages"=w1709:refnum<vi>[])  [unwired: 2 in, 1 out]
                    n958 = To Long Integer(number=w1710) -> (32bit integer=w1711:i32)
                    n959 = Index Array(array=w1709, index=w1711) -> (element=w1712:refnum<vi>)
                    n960 = property class="Page"(reference=w1712, error in=w1714, "PageEnb"=T26."Page Disabled & Grayed" ("Page Enabled State")) -> (error out=w1721:errorcluster)  [unwired: 1 out]
                    n961 = property on="Main tab control" class="TabCtl (strict)"(error in=w1721, "Value"=w1719) -> (error out=w1715:errorcluster, "Pages"=w1720:refnum<vi>[])  [unwired: 1 in, 1 out]
                    n962 = To Long Integer(number=w1719) -> (32bit integer=w1718:i32)
                    n963 = Index Array(array=w1720, index=w1718) -> (element=w1717:refnum<vi>)
                    n964 = property class="Page"(reference=w1717, error in=w1715, "PageEnb"=T26."Page Disabled & Grayed" ("Page Enabled State")) -> (error out=w1728:errorcluster)  [unwired: 1 out]
                    n965 = property on="Main tab control" class="TabCtl (strict)"(error in=w1728, "Value"=w1723) -> (error out=w1727:errorcluster, "Pages"=w1722:refnum<vi>[])  [unwired: 1 in, 1 out]
                    n966 = To Long Integer(number=w1723) -> (32bit integer=w1724:i32)
                    n967 = Index Array(array=w1722, index=w1724) -> (element=w1725:refnum<vi>)
                    n968 = property class="Page"(reference=w1725, error in=w1727, "PageEnb"=T26."Page Enabled" ("Page Enabled State")) -> (error out=w1707:errorcluster)  [unwired: 1 out]
                    n969 = property on="Back to Settings" class="Bool"(error in=w1707, "Visible"=FALSE) -> ()  [unwired: 1 in, 2 out]
                  }
                }
              }
            }
          }
          frame Enabled {
          }
        }
        n970 = event shown="[1] \"Zones (analysis)\", \"Show full track (analysis)\": Value Change" {
          selector: _ -> [_ _ _]
          dyn-events: _ -> [_ _ _]
          timeout: 0 -> [_ _ _]
          tunnel: "Zones (analysis)" -> [_ w1686 _]
          tunnel: "Show full track (analysis)" -> [_ w1685 _]
          event Timeout {
            n971 = event-data() -> ()  [unwired: 1 in, 3 out]
          }
          event "Zones (analysis)", "Show full track (analysis)": Value Change {
            n972 = event-data() -> ()  [unwired: 1 in, 6 out]
            n973 = Build Array(w1686, w1685) -> (w1684:bool[])
            n974 = Boolean Array To Number(Boolean array=w1684) -> (number=w1683:u32)
            n975 = case shown="0, Default" w1683 {
              frame 0, Default {
                n976 = property on="Map index (analysis)" class="DigNum (strict)"("Value"=1 ("Map index (analysis)")) -> ()  [unwired: 2 in, 2 out]
                n977 = property on="Show heatmap (analysis)" class="Bool (strict)"("Value"=FALSE ("Show full track (analysis)")) -> ()  [unwired: 2 in, 2 out]
              }
              frame 1 {
                n978 = property on="Map index (analysis)" class="DigNum (strict)"("Value"=0 ("Map index (analysis)")) -> ()  [unwired: 2 in, 2 out]
                n979 = property on="Show heatmap (analysis)" class="Bool (strict)"("Value"=FALSE ("Show full track (analysis)")) -> ()  [unwired: 2 in, 2 out]
              }
              frame 2 {
                n980 = property on="Map index (analysis)" class="DigNum (strict)"("Value"=4 ("Map index (analysis)")) -> ()  [unwired: 2 in, 2 out]
                n981 = property on="Show heatmap (analysis)" class="Bool (strict)"("Value"=FALSE ("Show full track (analysis)")) -> ()  [unwired: 2 in, 2 out]
              }
              frame 3 {
                n982 = property on="Map index (analysis)" class="DigNum (strict)"("Value"=3 ("Map index (analysis)")) -> ()  [unwired: 2 in, 2 out]
                n983 = property on="Show heatmap (analysis)" class="Bool (strict)"("Value"=FALSE ("Show full track (analysis)")) -> ()  [unwired: 2 in, 2 out]
              }
            }
          }
          event "Show heatmap (analysis)": Value Change {
            n984 = event-data() -> ("NewVal"=w1695:bool)  [unwired: 1 in, 5 out]
            n985 = case shown="True" w1695 {
              frame False {
                n986 = property on="Map index (analysis)" class="DigNum (strict)"("Value"=0 ("Map index (analysis)")) -> ()  [unwired: 2 in, 2 out]
                n987 = property on="Zones (analysis)" class="Bool (strict)"("Value"=TRUE ("Zones (analysis)")) -> ()  [unwired: 2 in, 2 out]
              }
              frame True {
                n988 = property on="Map index (analysis)" class="DigNum (strict)"("Value"=2 ("Map index (analysis)")) -> ()  [unwired: 2 in, 2 out]
                n989 = property on="Zones (analysis)" class="Bool (strict)"("Value"=FALSE ("Show full track (analysis)")) -> ()  [unwired: 2 in, 2 out]
                n990 = property on="Show full track (analysis)" class="Bool (strict)"("Value"=TRUE ("Show full track (analysis)")) -> ()  [unwired: 2 in, 2 out]
              }
            }
          }
        }
        n991 = global read "SW_Globals.vi" "Diagram no zones"() -> (w1667:picture)
        n992 = global read "SW_Globals.vi" "Full track with no zones"() -> (w1661:picture)
        n993 = global read "SW_Globals.vi" "Full track with zones"() -> (w1665:picture)
        n994 = global read "SW_Globals.vi" "Density map"() -> (w1666:picture)
        n995 = Get Notifier Status(notifier=w1681) -> (current notification=w1679:bool)  [unwired: 1 in, 4 out]
        n996 = Get Notifier Status(notifier=w1674) -> (current notification=w1671:bool)  [unwired: 1 in, 4 out]
        n997 = global read "SW_Globals.vi" "Diagram"() -> (w1668:picture)
        n998 = Build Array(w1668, w1667, w1666, w1665, w1661) -> (w1664:picture[])
        n999 = Not(x=w1671) -> (.not. x?=w1673:bool)
        n1000 = Index Array(array=w1664, index="Map index (analysis)") -> (element=w1663:picture)
        n1001 = Or(x=w1673, y=w1679) -> (x .or. y?=w1675:bool)
        n1002 = And(x=w1679, y="Play/Pause") -> (x .and. y?=w1682:bool)
        n1003 = Not(x="Play/Pause") -> (.not. x?=w1677:bool)
        n1004 = And(x=w1675, y=w1677) -> (x .and. y?=w1676:bool)
        n1005 = case shown="True" w1682 {
          tunnel: w1663 -> [w1768 w1815]
          tunnel: "Zones (analysis)" -> [_ w1814]
          tunnel: [w1768 w1813] -> w1680
          tunnel: w1670 -> [_ w1793]
          frame False {
          }
          frame True {
            n1006 = disable-structure shown="Disabled" {
              frame Disabled {
                (unwired) "%<%H:%M:%S%3u%p%d.%m.%Y>T" ("format string")
                n1007 = Get Date/Time In Seconds() -> (seconds since 1Jan1904=w1835:timestamp)
                n1008 = Scan From String(default 1=w1835) -> ()  [unwired: 5 in, 3 out]
              }
              frame Enabled {
              }
            }
            n1009 = Divide(x=u32 1000, y=w1793) -> (x/y=w1795:dbl)
            n1010 = local read "TTL outputs"() -> (w1783:u8[])
            n1011 = local read "TTL inputs"() -> (w1784:u8[])
            n1012 = Multiply(x=w1795, y="Trace in analysis, s") -> (x*y=w1786:dbl)
            n1013 = local read "Absolute timestamp (rec)"() -> (w1802:dbl[])
            n1014 = local read "Relative timestamp (rec)"() -> (w1811:dbl[])
            n1015 = local read "alpha rot. angle"() -> (w1830:dbl[])
            n1016 = property on="Timeline" class="Slide (strict)"("DisabledEnum"=T9."Enabled" ("Disabled")) -> (error out=w1804:errorcluster)  [unwired: 2 in, 1 out]
            n1017 = local read "Index of the last recorded timepoint"() -> (w1807:i32)
            n1018 = local read "Zones preference array (loaded)"() -> (w1798:dbl[][])
            n1019 = local read "X coord"() -> (w1832:dbl[])
            n1020 = local read "Y coord"() -> (w1831:dbl[])
            n1021 = property on="Open File" class="Bool"(error in=w1804, "DisabledEnum"=T9."Disabled and Grayed Out" ("Disabled")) -> ()  [unwired: 1 in, 2 out]
            n1022 = feedback #5(0.0125 ("String")) -> (w1820:dbl)
            n1023 = Select(t=FALSE, s=w1814, f=TRUE) -> (s? t:f=w1825:bool)
            n1024 = feedback #6(u16 3 ("Value")) -> (w1791:u16)
            n1025 = feedback #7(0) -> (w1782:u32)
            n1026 = Index Array(array=w1784, index=w1782) -> (element=w1781:u8)
            n1027 = Index Array(array=w1783, index=w1782) -> (element=w1780:u8)
            n1028 = Number To Boolean Array(number=w1781) -> (Boolean array=w1779:bool[])
            n1029 = Number To Boolean Array(number=w1780) -> (Boolean array=w1778:bool[])
            n1030 = Or(x=w1779, y=w1778) -> (x .or. y?=w1770:bool[])
            n1031 = Index Array(array=w1770, index=0) -> (element=→"TTL IO 1 (analysis)":bool)
            n1032 = Index Array(array=w1770, index=1) -> (element=→"TTL IO 2 (analysis)":bool)
            n1033 = Index Array(array=w1770, index=2) -> (element=→"TTL IO 3 (analysis)":bool)
            n1034 = Index Array(array=w1770, index=3) -> (element=→"TTL IO 4 (analysis)":bool)
            n1035 = Index Array(array=w1802, index=w1782) -> (element=w1801:dbl)
            n1036 = Index Array(array=w1830, index=w1782) -> (element=w1829:dbl)
            n1037 = Index Array(array=w1811, index=w1782) -> (element=w1803:dbl)
            n1038 = feedback-in #5(w1803) -> ()
            n1039 = property on="Recorded timestamp" class="DigNum (strict)"("Value"=w1803) -> ()  [unwired: 2 in, 2 out]
            n1040 = Subtract(x=w1803, y=w1820) -> (x-y=w1819:dbl)
            n1041 = Index Array(array=w1798, index (row)=w1782) -> (element=→"Zones allocation (normalized) in analysis":dbl[])  [unwired: 1 in]
            n1042 = Index Array(array=w1832, index=w1782) -> (element=w1824:dbl)
            n1043 = Index Array(array=w1831, index=w1782) -> (element=w1823:dbl)
            n1044 = To Time Stamp(1:w1801) -> (0:w1800:timestamp)
            n1045 = property on="Recorded at time" class="AbsTime (strict)"("Value"=w1800) -> ()  [unwired: 2 in, 2 out]
            n1046 = event shown="[1] \"Timeline\": Value Change" {
              selector: _ -> [_ _ _]
              dyn-events: _ -> [_ _ _]
              timeout: 1 -> [_ _ _]
              tunnel: w1803 -> [w1844 _ _]
              tunnel: w1782 -> [w1843 _ w1856]
              tunnel: [w1842 w1854 w1856] -> w1810
              tunnel: w1811 -> [_ _ _]
              tunnel: w1807 -> [_ w1847 _]
              tunnel: [w1836 w1845 w1855] -> w1789
              tunnel: w1791 -> [_ w1845 w1855]
              event Timeout {
                n1047 = event-data() -> ()  [unwired: 1 in, 3 out]
                n1048 = property on="Timeline" class="Slide (strict)"("Value"=w1844) -> ()  [unwired: 2 in, 2 out]
                n1049 = property on="Speed" class="Ring (strict)"() -> ("RingText.Text"=w1840:string, "Strings []"=w1841:string[], "StringsAndValues[]"=w1838:T33)  [unwired: 2 in, 2 out]
                n1050 = Search 1D Array(1D array=w1841, element=w1840) -> (index of element=w1839:i32)  [unwired: 1 in]
                n1051 = Index Array(array=w1838, index=w1839) -> (element=w1837:cluster{"String":string, "Value":u16})
                n1052 = Unbundle(w1837) -> ("Value"=w1836:u16)  [unwired: 1 out]
                n1053 = Add(x=w1836, y=w1843) -> (x+y=w1842:u32)
              }
              event "Timeline": Value Change {
                n1054 = event-data() -> ("NewVal"=w1852:dbl)  [unwired: 1 in, 5 out]
                n1055 = property on="Timeline" class="Slide (strict)"() -> ("Scale.Maximum"=w1853:dbl, "Scale.Minimum"=w1851:dbl)  [unwired: 2 in, 2 out]
                n1056 = Subtract(x=w1852, y=w1851) -> (x-y=w1850:dbl)
                n1057 = Subtract(x=w1853, y=w1851) -> (x-y=w1849:dbl)
                n1058 = Divide(x=w1850, y=w1849) -> (x/y=w1848:dbl)
                "ceil(x): smallest int >= x" <- w1848
                n1059 = Multiply(x=w1848, y=w1847) -> (x*y=w1846:dbl)
                n1060 = To Unsigned Long Integer(number=w1846) -> (unsigned 32bit integer=w1854:u32)
              }
              event "Multiplyer of chart RX 2": Value Change {
                n1061 = event-data() -> ("NewVal"=w1857:u8)  [unwired: 1 in, 5 out]
                n1062 = Multiply(x=w1857, y=10.0) -> (x*y=w1858:dbl)
                n1063 = property on="Mouse speed 2" class="WFChart (strict)"() -> (error out=w1859:errorcluster, "XScale.Maximum"=w1862:dbl)  [unwired: 2 in, 1 out]
                n1064 = Subtract(x=w1862, y=w1858) -> (x-y=w1860:dbl)
                n1065 = property on="Mouse speed 2" class="WFChart (strict)"(error in=w1859, "XScale.Minimum"=w1860) -> ()  [unwired: 1 in, 2 out]
              }
            }
            n1066 = call "FL_Calc_speed_on_the_fly.vi"("Y coord, mm"=w1823, "X coord, mm"=w1824, "Time per frame, s"=w1819) -> ("Mouse speed, mm/s"=w1817:dbl)
            "Mouse speed digi 2" <- w1817
            n1067 = To Time Stamp(1:w1803) -> (0:w1821:timestamp)
            n1068 = Build Array(w1817) -> (w1822:dbl[])
            n1069 = Bundle By Name("t0"=w1821, "Y"=w1822) -> (→"Mouse speed 2":waveform(dbl))  [unwired: 1 in]
            n1070 = feedback-in #6(w1789) -> ()
            n1071 = Greater Or Equal?(x=w1810, y=w1807) -> (x >= y?=w1799:bool)
            n1072 = Divide(x=w1789, y=u16 3) -> (x/y=w1785:dbl)
            n1073 = Divide(x=w1786, y=w1785) -> (x/y=w1787:dbl)
            n1074 = Select(t=u32 0, s=w1799, f=w1810) -> (s? t:f=w1809:u32)
            n1075 = feedback-in #7(w1809) -> ()
            n1076 = property on="Diagram at analysis" class="Pict"() -> ("Bounds"=w1834:T14)  [unwired: 2 in, 2 out]
            n1077 = local read "Pixels per mm"() -> (w1833:dbl)
            n1078 = Round To Nearest(number=w1787) -> (nearest integer value=w1792:dbl)
            n1079 = call "SW_Draw_mouse_br.vi"("Input picture (background)"=w1815, "Size of the image"=w1834, "Pixels per mm"=w1833, "Mouse coord cartesian X, mm"=w1824, "Mouse coord cartesian Y, mm"=w1823, "Mouse angle of rotation, deg"=w1829, "Show mouse lineout"=w1825, "Trace length, samples"=w1792) -> ("Output picture (with mouse overlay)"=w1813:picture)  [unwired: 6 in, 1 out]
          }
        }
        "Diagram at analysis" <- w1680
        n1080 = case shown="True" w1676 {
          tunnel: w1672 -> [_ w1731]
          frame False {
          }
          frame True {
            n1081 = case "Open new file" shown="True" "Open File" {
              tunnel: w1731 -> [_ w1734]
              frame False {
              }
              frame True {
                n1082 = global read "SW_Globals.vi" "Cluster of paths"() -> (w1735:T18)
                n1083 = Unbundle By Name(w1735) -> ("Final csv output path"=w1745:path)
                n1084 = Strip Path(path=w1745) -> (stripped path=w1744:path)  [unwired: 1 out]
                n1085 = Strip Path(path=w1744) -> (stripped path=w1741:path)  [unwired: 1 out]
                n1086 = call "File Dialog"("start path"=w1741, "button label"="Open track", "pattern (all files)"="*.csv; *.tsv") -> ("selected path"=w1736:path, "exists"=w1740:bool, "cancelled"=w1738:bool)  [unwired: 9 in, 1 out]
                n1087 = Not(x=w1738) -> (.not. x?=w1739:bool)
                n1088 = And(x=w1740, y=w1739) -> (x .and. y?=w1737:bool)
                n1089 = case shown="True" w1737 {
                  tunnel: w1736 -> [_ w1750]
                  tunnel: w1735 -> [_ w1749]
                  tunnel: w1734 -> [_ w1746]
                  frame False {
                  }
                  frame True {
                    n1090 = flat-sequence {
                      tunnel: w1750 -> [w1752]
                      tunnel: [w1752] -> w1748
                      tunnel: [w1751] -> w1747
                      tunnel: w1749 -> [w1760]
                      tunnel: w1748 -> [w1759]
                      tunnel: w1747 -> [w1758]
                      tunnel: w1746 -> [w1767]
                      frame #0 {
                        n1091 = call <vilib>:"Get File Extension.vi"("file"=w1752) -> ("filename without extension"=w1756:string)  [unwired: 6 in, 4 out]
                        n1092 = Concatenate Strings(w1756, ".trset" ("string")) -> (w1753:string)
                        n1093 = Strip Path(path=w1752) -> (stripped path=w1754:path)  [unwired: 1 out]
                        n1094 = Build Path(base path=w1754, name or relative path=w1753) -> (appended path=w1751:path)
                        "Settings file path" <- w1751
                        "Track path" <- w1752
                      }
                      frame #1 {
                        n1095 = Bundle By Name(cluster=w1760, "Final csv output path"=w1759, "Recording settings output path"=w1758) -> (w1757:T18)
                        n1096 = global write "SW_Globals.vi" "Cluster of paths"(w1757) -> ()
                      }
                      frame #2 {
                        n1097 = Unbundle By Name(w1767) -> ("Final CSV saved"=w1763:refnum<notifier>, "Data loaded"=w1766:refnum<notifier>, "Has been recorded"=w1761:refnum<notifier>)
                        n1098 = Send Notification(notification=TRUE, notifier=w1763) -> ()  [unwired: 1 in, 2 out]
                        n1099 = Send Notification(notification=FALSE, notifier=w1766) -> ()  [unwired: 1 in, 2 out]
                        n1100 = Send Notification(notification=TRUE, notifier=w1761) -> ()  [unwired: 1 in, 2 out]
                      }
                    }
                  }
                }
              }
            }
            n1101 = property on="Open File" class="Bool"("DisabledEnum"=T9."Enabled" ("Disabled")) -> (error out=w1729:errorcluster)  [unwired: 2 in, 1 out]
            n1102 = property on="Timeline" class="Slide (strict)"(error in=w1729, "DisabledEnum"=T9."Disabled and Grayed Out" ("Disabled")) -> ()  [unwired: 1 in, 2 out]
          }
        }
      }
    }
    n1103 = Wait Until Next ms Multiple(millisecond multiple=w992) -> ()  [unwired: 1 out]
    n1104 = Unbundle By Name(w988) -> ("Complete stop"=w983:refnum<notifier>)
    n1105 = Send Notification(notification="Stop Button", notifier=w983) -> (notifier out=w979:refnum<notifier>, error out=w980:errorcluster)  [unwired: 1 in]
    n1106 = Get Notifier Status(notifier=w979, error in (no error)=w980) -> (current notification=w981:bool)  [unwired: 4 out]
    n1107 = Or(x="Stop Button", y=w981) -> (x .or. y?=w982:bool)
  }
